vi "NIMS_NS_iir_comb.vi"(5 "Function name":string, 6 "Line number":i32, 7 "Number of outputs requested":i32, 8 "error in (no error)":errorcluster, 11 "[A]":variant[](array[variant])) -> (0 "error out":errorcluster, 3 "[funct(A)]":variant[](array[variant]))   [LabVIEW 2017]
uses:
  <vilib>/imath/engines/lvmath/Functions/Error Handling/error.ctl
  <instcachedir>/0/NIMS_RunTimeType_From StrictType (excl LVString)_1019F277F0A747EDBCA0F6C52CA54500.lvgen/NIMS_RunTimeType_From StrictType (excl LVString)_1019F277F0A747EDBCA0F6C52CA54500_000.vi
  <instcachedir>/0/NIMS_Get Scalar_w Error_1987D997E87247DDAC16EA23A5E9E4FC.lvgen/NIMS_Get Scalar_w Error_1987D997E87247DDAC16EA23A5E9E4FC_000.vi
  <instcachedir>/0/NIMS_Get Scalar_w Error_1987D997E87247DDAC16EA23A5E9E4FC.lvgen/NIMS_Get Scalar_w Error_1987D997E87247DDAC16EA23A5E9E4FC_003.vi
  <instcachedir>/0/NIMS_Get Row Vector_w Error - Matrix_7ECCFA0649AF47C08F6F0C496599EB01.lvgen/NIMS_Get Row Vector_w Error - Matrix_7ECCFA0649AF47C08F6F0C496599EB01_000.vi
  <instcachedir>/0/NIMS_Complex To Real_BE01396FDE034E8E94CEBBA1E368668D.lvgen/NIMS_Complex To Real_BE01396FDE034E8E94CEBBA1E368668D_000.vi
  <instcachedir>/0/NIMS_RunTimeType_To Numeric_1CBDAFC4EFAD4045A1DE52278D16738D.lvgen/NIMS_RunTimeType_To Numeric_1CBDAFC4EFAD4045A1DE52278D16738D_000.vi
  <vilib>/addons/Digital Filter Design/NI_DigFilter_MathScript.lvlib
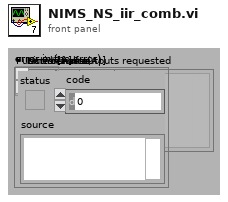
[diagram p1: front panel]
types:
  T1 = typedef "error.ctl" = enum16{"No Error", "Problem", "Input type must not be void", "Incorrect number of parameters", "Function not defined for non-numeric types", "An output variable of the user-defined function is undefined", "Function only defined for character arrays", "Function not defined for boolean, character, or single precision", "Function not defined for complex types", "Not a valid operation", "Inputs must be scalar", "Input matrices are not the same size", "Function only available on RT", "Input matrices must be nonnegative integers of the same type", "Arguments must be non-negative integers less than bitmax", "Number to complement must be less than 2^N", "Bit to get is outside range", "Bit to set is outside range", "Input must be real type ", "At least one parameter must be scalar", "Unable to display plug-in data on RT", "Function not defined for higher dimensional matrices", "Invalid attributes", "Wrong Type of Input Arguments", "Wrong Argument Option", "Invalid file identifier", "Indices must be real positive integers", "The variable is not a matrix data type.", "Number of elements must be the same for indices and values", "You cannot replace elements of a matrix with non-matrix data types.", "Cannot resize a 2D matrix with a linear index", "Unknown variable or symbol", "Indices out of range", "Empty matrix deletion can not be used with two indices", "Number of rows and columns must be the same for indices and values.", "Complex cannot be converted to Boolean", "Char cannot be converted to Boolean", "int64 cannot be converted to Boolean", "uint64 cannot be converted to Boolean", "You cannot convert a Boolean to a character.", "Incompatible input size in 3D surface function", "All rows must have the same number of columns", "Incompatible types", "Invalid matrix dimensions", "Dimension must be 1 or 2", "Base must be an integer between 2 and 36", "Invalid input", "Square matrix required", "Function 'timerstart' must be called before 'timerstop'", "Arguments must be positive real", "Step must not be zero", "Wrong number of input arguments", "Wrong number of output arguments", "Too many index arguments", "Input scalar must be >= 0", "Input scalar must be positive", "Input scalar must not be 0", "Input scalar must be in range [0,1]", "Can't use conditionally defined variable that's undefined", "Input must be a vector", "RT Exec Trace Toolkit not licensed", "Empty vector error", "All elements must be in domain [-1,1]", "All real elements of input vector must be >= 0", "All elements of input vector must be positive", "Values of input vectors are not compatible", "DAQmx not installed", "Input vector must be an increasing vector", "Dereferenced field does not exist within the struct", "A vector or matrix of structures must be indexed before it can be dereferenced", "Lenths of two input vectors are not compatible", "Invalid fieldname", "Empty matrix error", "Cannot use '.' on a type other than Struct", "Unused074", "Data type of the struct's field name is invalid", "Using . to dereference data that is not a struct", "Input struct contains invalid type ", "Size of input matrix is incompatible with input size", "Invalid format specifier", "Could not find field within struct", "Bad permutation array", "Mismatched fieldnames", "ode: User Function could not be opened", "ode: User Function signature does not meet ode requirements", "Unused085", "RunTime: MathScript could not be compiled", "Unknown function", "Only scalars and strings supported", "ode: User Function signature has incorrect number of inputs", "ode:User Function signature has incorrect number of outputs", "Range is too large", "End used without variable", "Function not available (RTE)", "Custom user error", "Arguments must be integers less than bitmax", "Shared library not found", "Header file not found", "Shared library already loaded", "Shared library not loaded", "Shared library function not found", "Shared library string return problem", "Problem calling shared library function", "Problem loading shared library from OS", "Problem parsing shared library header file", "Shared library incompatible types", "Shared library unsupported return type", "Shared library function not exported", "Shared library unsupported input type", "Problem unloading shared library from OS", "Function only available from UI", "Function specified in argument is missing", "An internal error has occurred", "Invalid object", "Invalid property", "Read-only property", "A break command has occurred", "A continue command has occurred", "A return command has occurred", "ode: times parameter invalid", "Function specified in argument has incorrect signature", "Function not found in file", "Reserved keyword cannot be defined as variable", "Reserved keyword cannot be defined as a function or script", "Arguments must be string literals", "Function not supported on this platform", "All columns must have the same number of rows", "Function ignored in RTE warning", "Cannot use : as a parameter that is not a variable", "Output can't be coerced to requested type", "Function not supported on current target", "Variable dependent on an unwired function input", "Unused132", "Unused133", "Unused134", "Unused135", "Unused136", "Unused137", "Unused138", "Unused139", "Global/Persistent must only take constants as arguments.", "Varargin must be last input in the function definition.", "Varargout must be last output in the function definition.", "Invalid output type. Cannot output a cell array of any type other than string.", "Invalid output type. Type is a dynamic struct.", "Invalid output type. Type is a struct that has a field whose type is not known until run-time", "Invalid output type. Type is a struct that has a field which is a plot object.", "MathScript parser DLL missing", "MathScript requires LabVIEW Full", "MathScript license is invalid or missing", "Varargout not supported except in assignments."}
  T2 = typedef "NIMS_CH_character datatype.ctl" = cluster{"Numeric":u8}
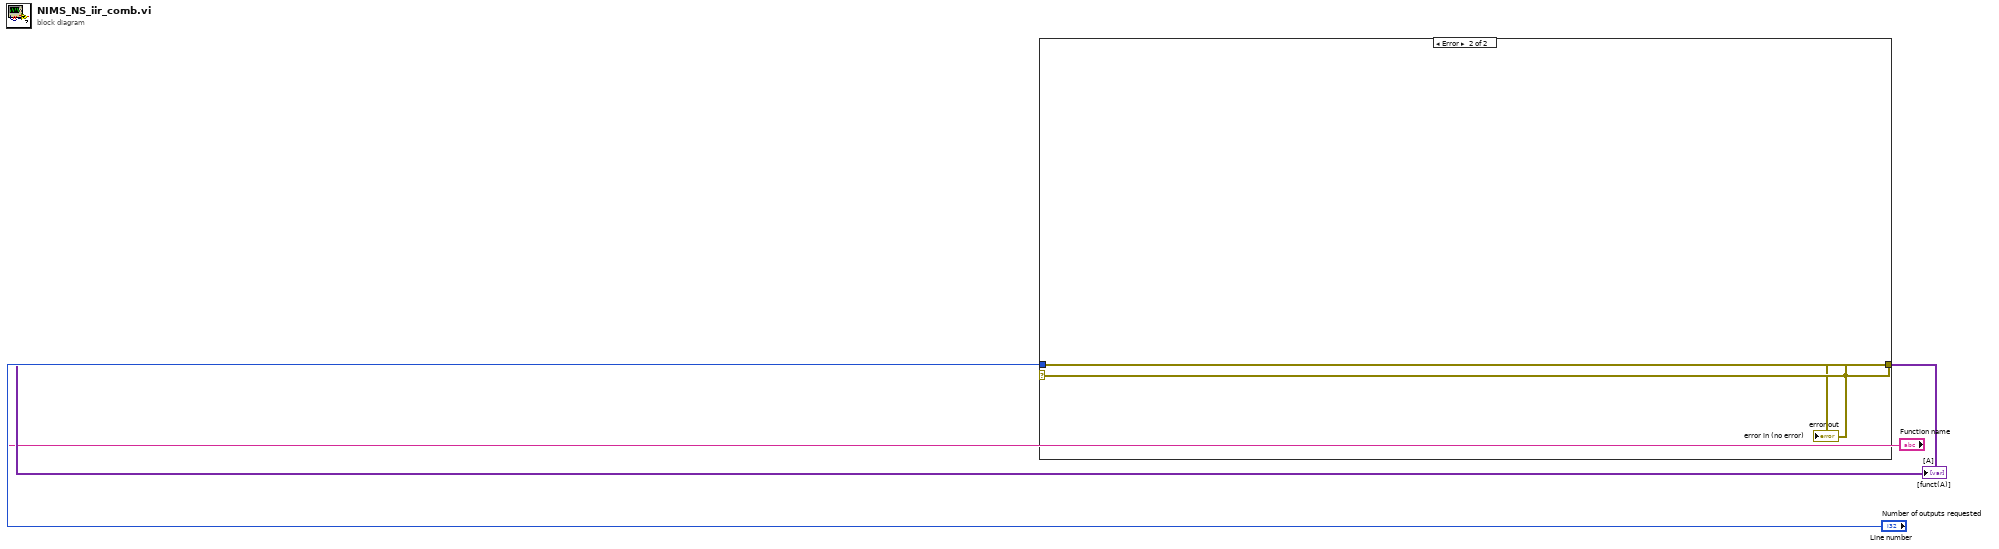
[diagram p0: block diagram]
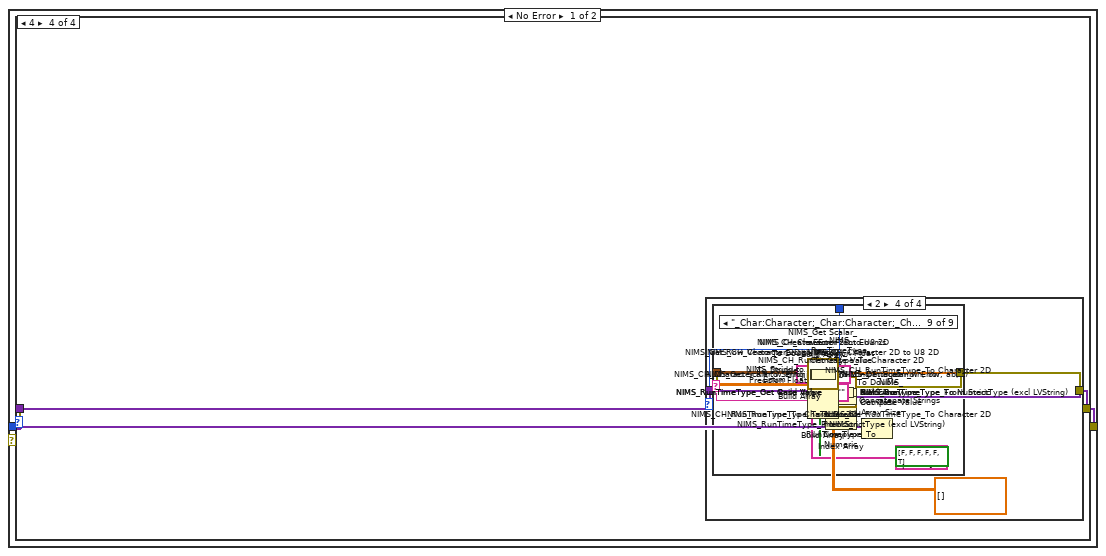
[diagram p2: hidden frame]
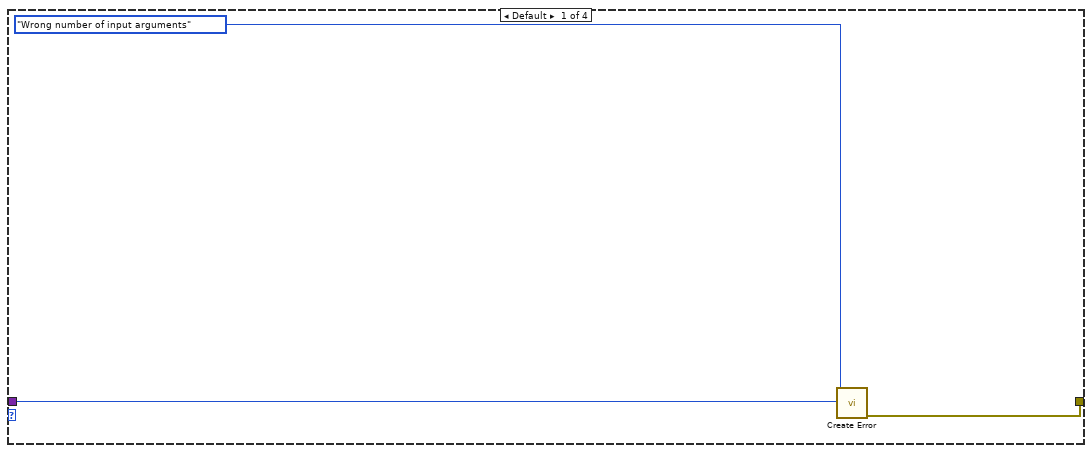
[diagram p3: hidden frame]
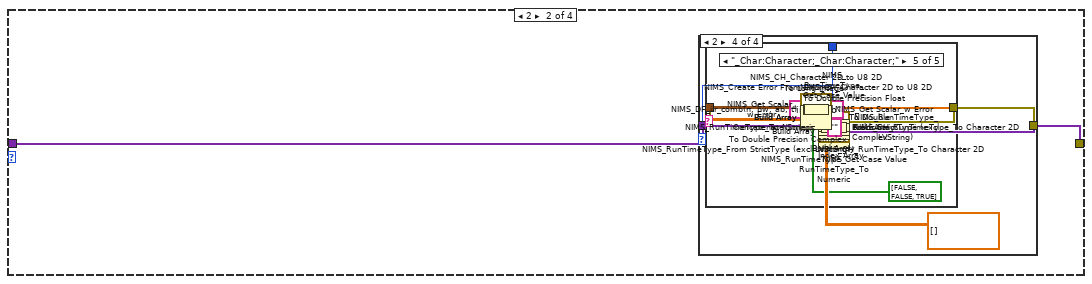
[diagram p4: hidden frame]
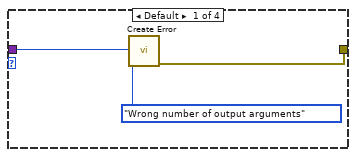
[diagram p5: hidden frame]
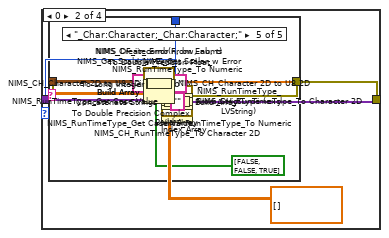
[diagram p6: hidden frame]
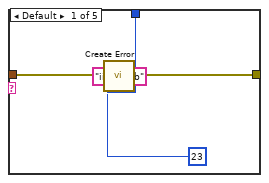
[diagram p7: hidden frame]
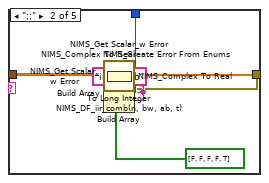
[diagram p8: hidden frame]
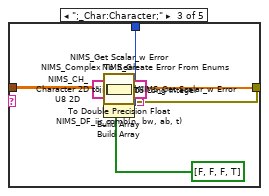
[diagram p9: hidden frame]
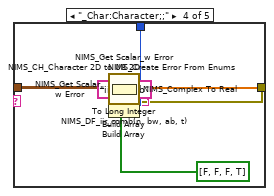
[diagram p10: hidden frame]
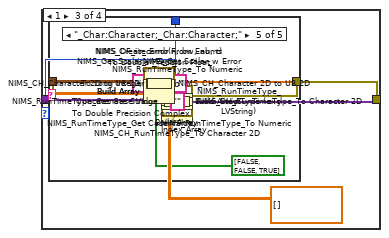
[diagram p11: hidden frame]
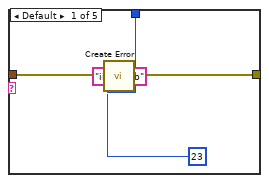
[diagram p12: hidden frame]
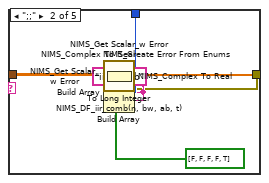
[diagram p13: hidden frame]
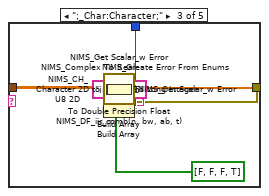
[diagram p14: hidden frame]
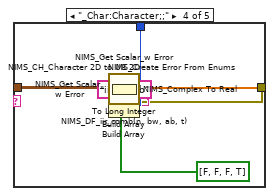
[diagram p15: hidden frame]
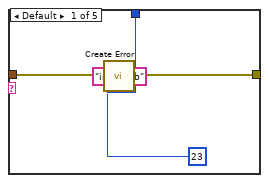
[diagram p16: hidden frame]
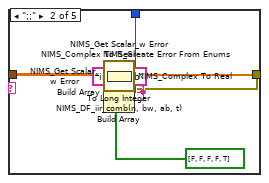
[diagram p17: hidden frame]
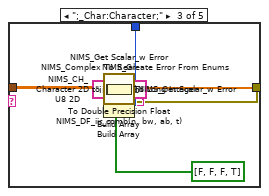
[diagram p18: hidden frame]
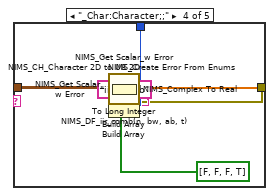
[diagram p19: hidden frame]
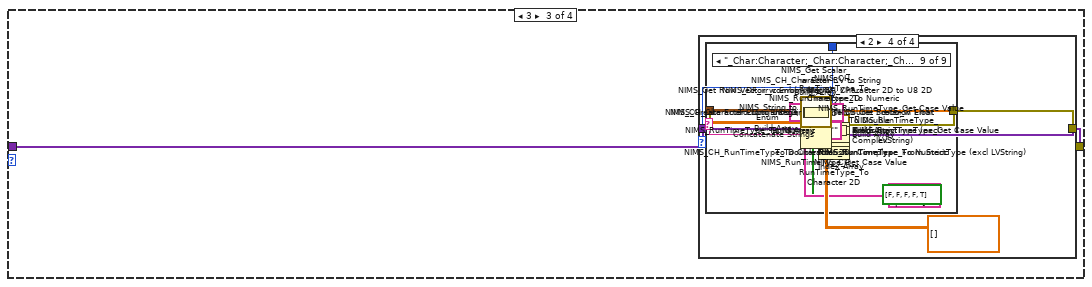
[diagram p20: hidden frame]
diagram:
  n1 = case shown="Error" "error in (no error)" {
    selector: "error in (no error)" -> [_ w2027]
    tunnel: [w15 _] -> w4
    tunnel: [w14 w2027] -> w3
    tunnel: "error in (no error)" -> [w13 _]
    tunnel: "Number of outputs requested" -> [w12 _]
    tunnel: "[A]" -> [w11 _]
    tunnel: "Function name" -> [w10 _]
    tunnel: "Line number" -> [w9 _]
    frame No Error {
      n2 = Array Size(array=w11) -> (size(s)=w8:i32)
      n3 = case shown="4" w8 {
        tunnel: [_ w27 w372 w1126] -> w15
        tunnel: w10 -> [w19 w24 w369 w1123]
        tunnel: w9 -> [w20 w25 w370 w1124]
        tunnel: w13 -> [w17 w23 w368 w1122]
        tunnel: [w16 w22 w367 w1121] -> w14
        tunnel: w12 -> [_ w21 w366 w1120]
        tunnel: w11 -> [_ w26 w371 w1125]
        frame Default {
          n4 = call <vilib>:"Create Error.vi"("Function name"=w19, "error in (no error)"=w17, "Error Enum"=error."Wrong number of input arguments", "Line number"=w20) -> ("error out"=w16:errorcluster)  [unwired: 6 in, 1 out]
        }
        frame 2 {
          n5 = case shown="2" w21 {
            tunnel: [_ w33 w141 w249] -> w27
            tunnel: w24 -> [w31 _ _ _]
            tunnel: w25 -> [w32 w52 w160 w273]
            tunnel: w23 -> [w29 w50 w158 w271]
            tunnel: [w28 w39 w147 w260] -> w22
            tunnel: w26 -> [_ w53 w161 w274]
            frame Default {
              n6 = call <vilib>:"Create Error.vi"("Function name"=w31, "error in (no error)"=w29, "Error Enum"=error."Wrong number of output arguments", "Line number"=w32) -> ("error out"=w28:errorcluster)  [unwired: 6 in, 1 out]
            }
            frame 0 {
              n7 = Index Array(array=w53) -> (element #1=w49:variant, element #2=w44:variant)  [unwired: 2 in]
              n8 = call <vilib>:"NIMS_RunTimeType_Get Case Value.vi"("Data In"=w44) -> ("Case Value"=w40:string)  [unwired: 9 in, 1 out]
              n9 = call <vilib>:"NIMS_CH_RunTimeType_To Character 2D.vi"("Variant"=w44) -> ("data"=w41:T2[][])  [unwired: 1 in]
              n10 = call-generic <vilib>:"NIMS_RunTimeType_To Numeric.vi"("DataType"=cdb[][] [], "Variant"=w44) -> ("data"=w42:cdb[][])  [unwired: 1 in]
              n11 = call <vilib>:"NIMS_RunTimeType_Get Case Value.vi"("Data In"=w49) -> ("Case Value"=w45:string)  [unwired: 9 in, 1 out]
              n12 = call <vilib>:"NIMS_CH_RunTimeType_To Character 2D.vi"("Variant"=w49) -> ("data"=w46:T2[][])  [unwired: 1 in]
              n13 = call-generic <vilib>:"NIMS_RunTimeType_To Numeric.vi"("DataType"=cdb[][] [], "Variant"=w49) -> ("data"=w47:cdb[][])  [unwired: 1 in]
              n14 = Concatenate Strings(w45, w40) -> (w51:string)
              n15 = case shown="\"_Char:Character;_Char:Character;\"" w51 {
                tunnel: w50 -> [w55 w64 w85 w106 w126]
                tunnel: [_ w59 w80 w101 w121] -> w38
                tunnel: [w54 w60 w81 w102 w122] -> w39
                tunnel: w47 -> [_ w78 w99 _ _]
                tunnel: w46 -> [_ _ _ w119 w139]
                tunnel: w42 -> [_ w74 _ w115 _]
                tunnel: w41 -> [_ _ w95 _ w135]
                tunnel: w52 -> [w58 w67 w88 w109 w129]
                frame Default {
                  n16 = call <vilib>:"Create Error.vi"("Function name"="iir_comb", "error in (no error)"=w55, "Error Enum"=23, "Line number"=w58) -> ("error out"=w54:errorcluster)  [unwired: 6 in, 1 out]
                }
                frame ";;" {
                  w62 = "iir_comb"
                  n17 = call-generic <vilib>:"NIMS_Complex To Real.vi"("A"=w74) -> ("Error Enum"=w70:T1, "Real(A)"=w73:dbl[][])  [unwired: 8 in, 1 out]
                  n18 = call-generic <vilib>:"NIMS_Get Scalar_w Error.vi"("A"=w73) -> ("Error Enum"=w69:T1, "Scalar"=w75:dbl)  [unwired: 8 in, 1 out]
                  n19 = call-generic <vilib>:"NIMS_Complex To Real.vi"("A"=w78) -> ("Error Enum"=w72:T1, "Real(A)"=w77:dbl[][])  [unwired: 8 in, 1 out]
                  n20 = To Long Integer(number=w77) -> (32bit integer=w76:i32[][])
                  n21 = call-generic <vilib>:"NIMS_Get Scalar_w Error.vi"("A"=w76) -> ("Error Enum"=w71:T1, "Scalar"=w79:i32)  [unwired: 8 in, 1 out]
                  n22 = call <vilib>:"NIMS_DF_iir_comb(n, bw, ab, t).vi"("bw"=w75, "n"=w79) -> ("error"=w68:i32, "b"=w59:dbl[])  [unwired: 7 in, 1 out]
                  n23 = Build Array(w62, w62, w62, w62, "iir_comb") -> (w65:string[])
                  n24 = Build Array(w72, w71, w70, w69, w68) -> (w66:i32[])
                  n25 = call <vilib>:"NIMS_Create Error From Enums.vi"("Error Code"=bool[] [FALSE, FALSE, FALSE, FALSE, TRUE], "error in (no error)"=w64, "Line no"=w67, "Error Enums"=w66, "Function names"=w65) -> ("error out"=w60:errorcluster)  [unwired: 6 in]
                }
                frame ";_Char:Character;" {
                  w83 = "iir_comb"
                  n26 = call <vilib>:"NIMS_CH_Character 2D to U8 2D.vi"("Character 2D array"=w95) -> ("U8 2D array"=w94:u8[][])  [unwired: 10 in]
                  n27 = To Double Precision Float(number=w94) -> (double precision float=w93:dbl[][])
                  n28 = call-generic <vilib>:"NIMS_Get Scalar_w Error.vi"("A"=w93) -> ("Error Enum"=w90:T1, "Scalar"=w96:dbl)  [unwired: 8 in, 1 out]
                  n29 = call-generic <vilib>:"NIMS_Complex To Real.vi"("A"=w99) -> ("Error Enum"=w92:T1, "Real(A)"=w98:dbl[][])  [unwired: 8 in, 1 out]
                  n30 = To Long Integer(number=w98) -> (32bit integer=w97:i32[][])
                  n31 = call-generic <vilib>:"NIMS_Get Scalar_w Error.vi"("A"=w97) -> ("Error Enum"=w91:T1, "Scalar"=w100:i32)  [unwired: 8 in, 1 out]
                  n32 = call <vilib>:"NIMS_DF_iir_comb(n, bw, ab, t).vi"("bw"=w96, "n"=w100) -> ("error"=w89:i32, "b"=w80:dbl[])  [unwired: 7 in, 1 out]
                  n33 = Build Array(w83, w83, w83, "iir_comb") -> (w86:string[])
                  n34 = Build Array(w92, w91, w90, w89) -> (w87:i32[])
                  n35 = call <vilib>:"NIMS_Create Error From Enums.vi"("Error Code"=bool[] [FALSE, FALSE, FALSE, TRUE], "error in (no error)"=w85, "Line no"=w88, "Error Enums"=w87, "Function names"=w86) -> ("error out"=w81:errorcluster)  [unwired: 6 in]
                }
                frame "_Char:Character;;" {
                  w104 = "iir_comb"
                  n36 = call-generic <vilib>:"NIMS_Complex To Real.vi"("A"=w115) -> ("Error Enum"=w112:T1, "Real(A)"=w114:dbl[][])  [unwired: 8 in, 1 out]
                  n37 = call-generic <vilib>:"NIMS_Get Scalar_w Error.vi"("A"=w114) -> ("Error Enum"=w111:T1, "Scalar"=w116:dbl)  [unwired: 8 in, 1 out]
                  n38 = call <vilib>:"NIMS_CH_Character 2D to U8 2D.vi"("Character 2D array"=w119) -> ("U8 2D array"=w118:u8[][])  [unwired: 10 in]
                  n39 = To Long Integer(number=w118) -> (32bit integer=w117:i32[][])
                  n40 = call-generic <vilib>:"NIMS_Get Scalar_w Error.vi"("A"=w117) -> ("Error Enum"=w113:T1, "Scalar"=w120:i32)  [unwired: 8 in, 1 out]
                  n41 = call <vilib>:"NIMS_DF_iir_comb(n, bw, ab, t).vi"("bw"=w116, "n"=w120) -> ("error"=w110:i32, "b"=w101:dbl[])  [unwired: 7 in, 1 out]
                  n42 = Build Array(w104, w104, w104, "iir_comb") -> (w107:string[])
                  n43 = Build Array(w113, w112, w111, w110) -> (w108:i32[])
                  n44 = call <vilib>:"NIMS_Create Error From Enums.vi"("Error Code"=bool[] [FALSE, FALSE, FALSE, TRUE], "error in (no error)"=w106, "Line no"=w109, "Error Enums"=w108, "Function names"=w107) -> ("error out"=w102:errorcluster)  [unwired: 6 in]
                }
                frame "_Char:Character;_Char:Character;" {
                  w124 = "iir_comb"
                  n45 = call <vilib>:"NIMS_CH_Character 2D to U8 2D.vi"("Character 2D array"=w135) -> ("U8 2D array"=w134:u8[][])  [unwired: 10 in]
                  n46 = To Double Precision Float(number=w134) -> (double precision float=w133:dbl[][])
                  n47 = call-generic <vilib>:"NIMS_Get Scalar_w Error.vi"("A"=w133) -> ("Error Enum"=w131:T1, "Scalar"=w136:dbl)  [unwired: 8 in, 1 out]
                  n48 = call <vilib>:"NIMS_CH_Character 2D to U8 2D.vi"("Character 2D array"=w139) -> ("U8 2D array"=w138:u8[][])  [unwired: 10 in]
                  n49 = To Long Integer(number=w138) -> (32bit integer=w137:i32[][])
                  n50 = call-generic <vilib>:"NIMS_Get Scalar_w Error.vi"("A"=w137) -> ("Error Enum"=w132:T1, "Scalar"=w140:i32)  [unwired: 8 in, 1 out]
                  n51 = call <vilib>:"NIMS_DF_iir_comb(n, bw, ab, t).vi"("bw"=w136, "n"=w140) -> ("error"=w130:i32, "b"=w121:dbl[])  [unwired: 7 in, 1 out]
                  n52 = Build Array(w124, w124, "iir_comb") -> (w127:string[])
                  n53 = Build Array(w132, w131, w130) -> (w128:i32[])
                  n54 = call <vilib>:"NIMS_Create Error From Enums.vi"("Error Code"=bool[] [FALSE, FALSE, TRUE], "error in (no error)"=w126, "Line no"=w129, "Error Enums"=w128, "Function names"=w127) -> ("error out"=w122:errorcluster)  [unwired: 6 in]
                }
              }
              n55 = Build Array(w38) -> (w37:dbl[][])
              n56 = To Double Precision Complex(1:w37) -> (0:w36:cdb[][])
              n57 = call-generic <vilib>:"NIMS_RunTimeType_From StrictType (excl LVString).vi"("Plug-In Name"="", "Data In"=w36) -> ("Data Out"=w34:variant)  [unwired: 2 in]
              n58 = Build Array(w34) -> (w33:variant[])
            }
            frame 1 {
              n59 = Index Array(array=w161) -> (element #1=w157:variant, element #2=w152:variant)  [unwired: 2 in]
              n60 = call <vilib>:"NIMS_RunTimeType_Get Case Value.vi"("Data In"=w152) -> ("Case Value"=w148:string)  [unwired: 9 in, 1 out]
              n61 = call <vilib>:"NIMS_CH_RunTimeType_To Character 2D.vi"("Variant"=w152) -> ("data"=w149:T2[][])  [unwired: 1 in]
              n62 = call-generic <vilib>:"NIMS_RunTimeType_To Numeric.vi"("DataType"=cdb[][] [], "Variant"=w152) -> ("data"=w150:cdb[][])  [unwired: 1 in]
              n63 = call <vilib>:"NIMS_RunTimeType_Get Case Value.vi"("Data In"=w157) -> ("Case Value"=w153:string)  [unwired: 9 in, 1 out]
              n64 = call <vilib>:"NIMS_CH_RunTimeType_To Character 2D.vi"("Variant"=w157) -> ("data"=w154:T2[][])  [unwired: 1 in]
              n65 = call-generic <vilib>:"NIMS_RunTimeType_To Numeric.vi"("DataType"=cdb[][] [], "Variant"=w157) -> ("data"=w155:cdb[][])  [unwired: 1 in]
              n66 = Concatenate Strings(w153, w148) -> (w159:string)
              n67 = case shown="\"_Char:Character;_Char:Character;\"" w159 {
                tunnel: w158 -> [w163 w172 w193 w214 w234]
                tunnel: [_ w167 w188 w209 w229] -> w146
                tunnel: [w162 w168 w189 w210 w230] -> w147
                tunnel: w155 -> [_ w186 w207 _ _]
                tunnel: w154 -> [_ _ _ w227 w247]
                tunnel: w150 -> [_ w182 _ w223 _]
                tunnel: w149 -> [_ _ w203 _ w243]
                tunnel: w160 -> [w166 w175 w196 w217 w237]
                frame Default {
                  n68 = call <vilib>:"Create Error.vi"("Function name"="iir_comb", "error in (no error)"=w163, "Error Enum"=23, "Line number"=w166) -> ("error out"=w162:errorcluster)  [unwired: 6 in, 1 out]
                }
                frame ";;" {
                  w170 = "iir_comb"
                  n69 = call-generic <vilib>:"NIMS_Complex To Real.vi"("A"=w182) -> ("Error Enum"=w178:T1, "Real(A)"=w181:dbl[][])  [unwired: 8 in, 1 out]
                  n70 = call-generic <vilib>:"NIMS_Get Scalar_w Error.vi"("A"=w181) -> ("Error Enum"=w177:T1, "Scalar"=w183:dbl)  [unwired: 8 in, 1 out]
                  n71 = call-generic <vilib>:"NIMS_Complex To Real.vi"("A"=w186) -> ("Error Enum"=w180:T1, "Real(A)"=w185:dbl[][])  [unwired: 8 in, 1 out]
                  n72 = To Long Integer(number=w185) -> (32bit integer=w184:i32[][])
                  n73 = call-generic <vilib>:"NIMS_Get Scalar_w Error.vi"("A"=w184) -> ("Error Enum"=w179:T1, "Scalar"=w187:i32)  [unwired: 8 in, 1 out]
                  n74 = call <vilib>:"NIMS_DF_iir_comb(n, bw, ab, t).vi"("bw"=w183, "n"=w187) -> ("error"=w176:i32, "b"=w167:dbl[])  [unwired: 7 in, 1 out]
                  n75 = Build Array(w170, w170, w170, w170, "iir_comb") -> (w173:string[])
                  n76 = Build Array(w180, w179, w178, w177, w176) -> (w174:i32[])
                  n77 = call <vilib>:"NIMS_Create Error From Enums.vi"("Error Code"=bool[] [FALSE, FALSE, FALSE, FALSE, TRUE], "error in (no error)"=w172, "Line no"=w175, "Error Enums"=w174, "Function names"=w173) -> ("error out"=w168:errorcluster)  [unwired: 6 in]
                }
                frame ";_Char:Character;" {
                  w191 = "iir_comb"
                  n78 = call <vilib>:"NIMS_CH_Character 2D to U8 2D.vi"("Character 2D array"=w203) -> ("U8 2D array"=w202:u8[][])  [unwired: 10 in]
                  n79 = To Double Precision Float(number=w202) -> (double precision float=w201:dbl[][])
                  n80 = call-generic <vilib>:"NIMS_Get Scalar_w Error.vi"("A"=w201) -> ("Error Enum"=w198:T1, "Scalar"=w204:dbl)  [unwired: 8 in, 1 out]
                  n81 = call-generic <vilib>:"NIMS_Complex To Real.vi"("A"=w207) -> ("Error Enum"=w200:T1, "Real(A)"=w206:dbl[][])  [unwired: 8 in, 1 out]
                  n82 = To Long Integer(number=w206) -> (32bit integer=w205:i32[][])
                  n83 = call-generic <vilib>:"NIMS_Get Scalar_w Error.vi"("A"=w205) -> ("Error Enum"=w199:T1, "Scalar"=w208:i32)  [unwired: 8 in, 1 out]
                  n84 = call <vilib>:"NIMS_DF_iir_comb(n, bw, ab, t).vi"("bw"=w204, "n"=w208) -> ("error"=w197:i32, "b"=w188:dbl[])  [unwired: 7 in, 1 out]
                  n85 = Build Array(w191, w191, w191, "iir_comb") -> (w194:string[])
                  n86 = Build Array(w200, w199, w198, w197) -> (w195:i32[])
                  n87 = call <vilib>:"NIMS_Create Error From Enums.vi"("Error Code"=bool[] [FALSE, FALSE, FALSE, TRUE], "error in (no error)"=w193, "Line no"=w196, "Error Enums"=w195, "Function names"=w194) -> ("error out"=w189:errorcluster)  [unwired: 6 in]
                }
                frame "_Char:Character;;" {
                  w212 = "iir_comb"
                  n88 = call-generic <vilib>:"NIMS_Complex To Real.vi"("A"=w223) -> ("Error Enum"=w220:T1, "Real(A)"=w222:dbl[][])  [unwired: 8 in, 1 out]
                  n89 = call-generic <vilib>:"NIMS_Get Scalar_w Error.vi"("A"=w222) -> ("Error Enum"=w219:T1, "Scalar"=w224:dbl)  [unwired: 8 in, 1 out]
                  n90 = call <vilib>:"NIMS_CH_Character 2D to U8 2D.vi"("Character 2D array"=w227) -> ("U8 2D array"=w226:u8[][])  [unwired: 10 in]
                  n91 = To Long Integer(number=w226) -> (32bit integer=w225:i32[][])
                  n92 = call-generic <vilib>:"NIMS_Get Scalar_w Error.vi"("A"=w225) -> ("Error Enum"=w221:T1, "Scalar"=w228:i32)  [unwired: 8 in, 1 out]
                  n93 = call <vilib>:"NIMS_DF_iir_comb(n, bw, ab, t).vi"("bw"=w224, "n"=w228) -> ("error"=w218:i32, "b"=w209:dbl[])  [unwired: 7 in, 1 out]
                  n94 = Build Array(w212, w212, w212, "iir_comb") -> (w215:string[])
                  n95 = Build Array(w221, w220, w219, w218) -> (w216:i32[])
                  n96 = call <vilib>:"NIMS_Create Error From Enums.vi"("Error Code"=bool[] [FALSE, FALSE, FALSE, TRUE], "error in (no error)"=w214, "Line no"=w217, "Error Enums"=w216, "Function names"=w215) -> ("error out"=w210:errorcluster)  [unwired: 6 in]
                }
                frame "_Char:Character;_Char:Character;" {
                  w232 = "iir_comb"
                  n97 = call <vilib>:"NIMS_CH_Character 2D to U8 2D.vi"("Character 2D array"=w243) -> ("U8 2D array"=w242:u8[][])  [unwired: 10 in]
                  n98 = To Double Precision Float(number=w242) -> (double precision float=w241:dbl[][])
                  n99 = call-generic <vilib>:"NIMS_Get Scalar_w Error.vi"("A"=w241) -> ("Error Enum"=w239:T1, "Scalar"=w244:dbl)  [unwired: 8 in, 1 out]
                  n100 = call <vilib>:"NIMS_CH_Character 2D to U8 2D.vi"("Character 2D array"=w247) -> ("U8 2D array"=w246:u8[][])  [unwired: 10 in]
                  n101 = To Long Integer(number=w246) -> (32bit integer=w245:i32[][])
                  n102 = call-generic <vilib>:"NIMS_Get Scalar_w Error.vi"("A"=w245) -> ("Error Enum"=w240:T1, "Scalar"=w248:i32)  [unwired: 8 in, 1 out]
                  n103 = call <vilib>:"NIMS_DF_iir_comb(n, bw, ab, t).vi"("bw"=w244, "n"=w248) -> ("error"=w238:i32, "b"=w229:dbl[])  [unwired: 7 in, 1 out]
                  n104 = Build Array(w232, w232, "iir_comb") -> (w235:string[])
                  n105 = Build Array(w240, w239, w238) -> (w236:i32[])
                  n106 = call <vilib>:"NIMS_Create Error From Enums.vi"("Error Code"=bool[] [FALSE, FALSE, TRUE], "error in (no error)"=w234, "Line no"=w237, "Error Enums"=w236, "Function names"=w235) -> ("error out"=w230:errorcluster)  [unwired: 6 in]
                }
              }
              n107 = Build Array(w146) -> (w145:dbl[][])
              n108 = To Double Precision Complex(1:w145) -> (0:w144:cdb[][])
              n109 = call-generic <vilib>:"NIMS_RunTimeType_From StrictType (excl LVString).vi"("Plug-In Name"="", "Data In"=w144) -> ("Data Out"=w142:variant)  [unwired: 2 in]
              n110 = Build Array(w142) -> (w141:variant[])
            }
            frame 2 {
              n111 = Index Array(array=w274) -> (element #1=w270:variant, element #2=w265:variant)  [unwired: 2 in]
              n112 = call <vilib>:"NIMS_RunTimeType_Get Case Value.vi"("Data In"=w265) -> ("Case Value"=w261:string)  [unwired: 9 in, 1 out]
              n113 = call <vilib>:"NIMS_CH_RunTimeType_To Character 2D.vi"("Variant"=w265) -> ("data"=w262:T2[][])  [unwired: 1 in]
              n114 = call-generic <vilib>:"NIMS_RunTimeType_To Numeric.vi"("DataType"=cdb[][] [], "Variant"=w265) -> ("data"=w263:cdb[][])  [unwired: 1 in]
              n115 = call <vilib>:"NIMS_RunTimeType_Get Case Value.vi"("Data In"=w270) -> ("Case Value"=w266:string)  [unwired: 9 in, 1 out]
              n116 = call <vilib>:"NIMS_CH_RunTimeType_To Character 2D.vi"("Variant"=w270) -> ("data"=w267:T2[][])  [unwired: 1 in]
              n117 = call-generic <vilib>:"NIMS_RunTimeType_To Numeric.vi"("DataType"=cdb[][] [], "Variant"=w270) -> ("data"=w268:cdb[][])  [unwired: 1 in]
              n118 = Concatenate Strings(w266, w261) -> (w272:string)
              n119 = case shown="\"_Char:Character;_Char:Character;\"" w272 {
                tunnel: w271 -> [w276 w286 w308 w330 w351]
                tunnel: [_ w281 w303 w325 w346] -> w259
                tunnel: [_ w280 w302 w324 w345] -> w255
                tunnel: [w275 w282 w304 w326 w347] -> w260
                tunnel: w268 -> [_ w300 w322 _ _]
                tunnel: w267 -> [_ _ _ w343 w364]
                tunnel: w263 -> [_ w296 _ w339 _]
                tunnel: w262 -> [_ _ w318 _ w360]
                tunnel: w273 -> [w279 w289 w311 w333 w354]
                frame Default {
                  n120 = call <vilib>:"Create Error.vi"("Function name"="iir_comb", "error in (no error)"=w276, "Error Enum"=23, "Line number"=w279) -> ("error out"=w275:errorcluster)  [unwired: 6 in, 1 out]
                }
                frame ";;" {
                  w284 = "iir_comb"
                  n121 = call-generic <vilib>:"NIMS_Complex To Real.vi"("A"=w296) -> ("Error Enum"=w292:T1, "Real(A)"=w295:dbl[][])  [unwired: 8 in, 1 out]
                  n122 = call-generic <vilib>:"NIMS_Get Scalar_w Error.vi"("A"=w295) -> ("Error Enum"=w291:T1, "Scalar"=w297:dbl)  [unwired: 8 in, 1 out]
                  n123 = call-generic <vilib>:"NIMS_Complex To Real.vi"("A"=w300) -> ("Error Enum"=w294:T1, "Real(A)"=w299:dbl[][])  [unwired: 8 in, 1 out]
                  n124 = To Long Integer(number=w299) -> (32bit integer=w298:i32[][])
                  n125 = call-generic <vilib>:"NIMS_Get Scalar_w Error.vi"("A"=w298) -> ("Error Enum"=w293:T1, "Scalar"=w301:i32)  [unwired: 8 in, 1 out]
                  n126 = call <vilib>:"NIMS_DF_iir_comb(n, bw, ab, t).vi"("bw"=w297, "n"=w301) -> ("error"=w290:i32, "a"=w280:dbl[], "b"=w281:dbl[])  [unwired: 7 in]
                  n127 = Build Array(w284, w284, w284, w284, "iir_comb") -> (w287:string[])
                  n128 = Build Array(w294, w293, w292, w291, w290) -> (w288:i32[])
                  n129 = call <vilib>:"NIMS_Create Error From Enums.vi"("Error Code"=bool[] [FALSE, FALSE, FALSE, FALSE, TRUE], "error in (no error)"=w286, "Line no"=w289, "Error Enums"=w288, "Function names"=w287) -> ("error out"=w282:errorcluster)  [unwired: 6 in]
                }
                frame ";_Char:Character;" {
                  w306 = "iir_comb"
                  n130 = call <vilib>:"NIMS_CH_Character 2D to U8 2D.vi"("Character 2D array"=w318) -> ("U8 2D array"=w317:u8[][])  [unwired: 10 in]
                  n131 = To Double Precision Float(number=w317) -> (double precision float=w316:dbl[][])
                  n132 = call-generic <vilib>:"NIMS_Get Scalar_w Error.vi"("A"=w316) -> ("Error Enum"=w313:T1, "Scalar"=w319:dbl)  [unwired: 8 in, 1 out]
                  n133 = call-generic <vilib>:"NIMS_Complex To Real.vi"("A"=w322) -> ("Error Enum"=w315:T1, "Real(A)"=w321:dbl[][])  [unwired: 8 in, 1 out]
                  n134 = To Long Integer(number=w321) -> (32bit integer=w320:i32[][])
                  n135 = call-generic <vilib>:"NIMS_Get Scalar_w Error.vi"("A"=w320) -> ("Error Enum"=w314:T1, "Scalar"=w323:i32)  [unwired: 8 in, 1 out]
                  n136 = call <vilib>:"NIMS_DF_iir_comb(n, bw, ab, t).vi"("bw"=w319, "n"=w323) -> ("error"=w312:i32, "a"=w302:dbl[], "b"=w303:dbl[])  [unwired: 7 in]
                  n137 = Build Array(w306, w306, w306, "iir_comb") -> (w309:string[])
                  n138 = Build Array(w315, w314, w313, w312) -> (w310:i32[])
                  n139 = call <vilib>:"NIMS_Create Error From Enums.vi"("Error Code"=bool[] [FALSE, FALSE, FALSE, TRUE], "error in (no error)"=w308, "Line no"=w311, "Error Enums"=w310, "Function names"=w309) -> ("error out"=w304:errorcluster)  [unwired: 6 in]
                }
                frame "_Char:Character;;" {
                  w328 = "iir_comb"
                  n140 = call-generic <vilib>:"NIMS_Complex To Real.vi"("A"=w339) -> ("Error Enum"=w336:T1, "Real(A)"=w338:dbl[][])  [unwired: 8 in, 1 out]
                  n141 = call-generic <vilib>:"NIMS_Get Scalar_w Error.vi"("A"=w338) -> ("Error Enum"=w335:T1, "Scalar"=w340:dbl)  [unwired: 8 in, 1 out]
                  n142 = call <vilib>:"NIMS_CH_Character 2D to U8 2D.vi"("Character 2D array"=w343) -> ("U8 2D array"=w342:u8[][])  [unwired: 10 in]
                  n143 = To Long Integer(number=w342) -> (32bit integer=w341:i32[][])
                  n144 = call-generic <vilib>:"NIMS_Get Scalar_w Error.vi"("A"=w341) -> ("Error Enum"=w337:T1, "Scalar"=w344:i32)  [unwired: 8 in, 1 out]
                  n145 = call <vilib>:"NIMS_DF_iir_comb(n, bw, ab, t).vi"("bw"=w340, "n"=w344) -> ("error"=w334:i32, "a"=w324:dbl[], "b"=w325:dbl[])  [unwired: 7 in]
                  n146 = Build Array(w328, w328, w328, "iir_comb") -> (w331:string[])
                  n147 = Build Array(w337, w336, w335, w334) -> (w332:i32[])
                  n148 = call <vilib>:"NIMS_Create Error From Enums.vi"("Error Code"=bool[] [FALSE, FALSE, FALSE, TRUE], "error in (no error)"=w330, "Line no"=w333, "Error Enums"=w332, "Function names"=w331) -> ("error out"=w326:errorcluster)  [unwired: 6 in]
                }
                frame "_Char:Character;_Char:Character;" {
                  w349 = "iir_comb"
                  n149 = call <vilib>:"NIMS_CH_Character 2D to U8 2D.vi"("Character 2D array"=w360) -> ("U8 2D array"=w359:u8[][])  [unwired: 10 in]
                  n150 = To Double Precision Float(number=w359) -> (double precision float=w358:dbl[][])
                  n151 = call-generic <vilib>:"NIMS_Get Scalar_w Error.vi"("A"=w358) -> ("Error Enum"=w356:T1, "Scalar"=w361:dbl)  [unwired: 8 in, 1 out]
                  n152 = call <vilib>:"NIMS_CH_Character 2D to U8 2D.vi"("Character 2D array"=w364) -> ("U8 2D array"=w363:u8[][])  [unwired: 10 in]
                  n153 = To Long Integer(number=w363) -> (32bit integer=w362:i32[][])
                  n154 = call-generic <vilib>:"NIMS_Get Scalar_w Error.vi"("A"=w362) -> ("Error Enum"=w357:T1, "Scalar"=w365:i32)  [unwired: 8 in, 1 out]
                  n155 = call <vilib>:"NIMS_DF_iir_comb(n, bw, ab, t).vi"("bw"=w361, "n"=w365) -> ("error"=w355:i32, "a"=w345:dbl[], "b"=w346:dbl[])  [unwired: 7 in]
                  n156 = Build Array(w349, w349, "iir_comb") -> (w352:string[])
                  n157 = Build Array(w357, w356, w355) -> (w353:i32[])
                  n158 = call <vilib>:"NIMS_Create Error From Enums.vi"("Error Code"=bool[] [FALSE, FALSE, TRUE], "error in (no error)"=w351, "Line no"=w354, "Error Enums"=w353, "Function names"=w352) -> ("error out"=w347:errorcluster)  [unwired: 6 in]
                }
              }
              n159 = Build Array(w255) -> (w254:dbl[][])
              n160 = To Double Precision Complex(1:w254) -> (0:w253:cdb[][])
              n161 = call-generic <vilib>:"NIMS_RunTimeType_From StrictType (excl LVString).vi"("Plug-In Name"="", "Data In"=w253) -> ("Data Out"=w250:variant)  [unwired: 2 in]
              n162 = Build Array(w259) -> (w258:dbl[][])
              n163 = To Double Precision Complex(1:w258) -> (0:w257:cdb[][])
              n164 = call-generic <vilib>:"NIMS_RunTimeType_From StrictType (excl LVString).vi"("Plug-In Name"="", "Data In"=w257) -> ("Data Out"=w251:variant)  [unwired: 2 in]
              n165 = Build Array(w251, w250) -> (w249:variant[])
            }
          }
        }
        frame 3 {
          n166 = case shown="2" w366 {
            tunnel: [_ w378 w621 w864] -> w372
            tunnel: w369 -> [w376 _ _ _]
            tunnel: w370 -> [w377 w402 w645 w893]
            tunnel: w368 -> [w374 w400 w643 w891]
            tunnel: [w373 w384 w627 w875] -> w367
            tunnel: w371 -> [_ w403 w646 w894]
            frame Default {
              n167 = call <vilib>:"Create Error.vi"("Function name"=w376, "error in (no error)"=w374, "Error Enum"=error."Wrong number of output arguments", "Line number"=w377) -> ("error out"=w373:errorcluster)  [unwired: 6 in, 1 out]
            }
            frame 0 {
              n168 = Index Array(array=w403) -> (element #1=w399:variant, element #2=w394:variant, element #3=w389:variant)  [unwired: 3 in]
              n169 = call <vilib>:"NIMS_RunTimeType_Get Case Value.vi"("Data In"=w389) -> ("Case Value"=w385:string)  [unwired: 9 in, 1 out]
              n170 = call <vilib>:"NIMS_CH_RunTimeType_To Character 2D.vi"("Variant"=w389) -> ("data"=w386:T2[][])  [unwired: 1 in]
              n171 = call-generic <vilib>:"NIMS_RunTimeType_To Numeric.vi"("DataType"=cdb[][] [], "Variant"=w389) -> ("data"=w387:cdb[][])  [unwired: 1 in]
              n172 = call <vilib>:"NIMS_RunTimeType_Get Case Value.vi"("Data In"=w394) -> ("Case Value"=w390:string)  [unwired: 9 in, 1 out]
              n173 = call <vilib>:"NIMS_CH_RunTimeType_To Character 2D.vi"("Variant"=w394) -> ("data"=w391:T2[][])  [unwired: 1 in]
              n174 = call-generic <vilib>:"NIMS_RunTimeType_To Numeric.vi"("DataType"=cdb[][] [], "Variant"=w394) -> ("data"=w392:cdb[][])  [unwired: 1 in]
              n175 = call <vilib>:"NIMS_RunTimeType_Get Case Value.vi"("Data In"=w399) -> ("Case Value"=w395:string)  [unwired: 9 in, 1 out]
              n176 = call <vilib>:"NIMS_CH_RunTimeType_To Character 2D.vi"("Variant"=w399) -> ("data"=w396:T2[][])  [unwired: 1 in]
              n177 = call-generic <vilib>:"NIMS_RunTimeType_To Numeric.vi"("DataType"=cdb[][] [], "Variant"=w399) -> ("data"=w397:cdb[][])  [unwired: 1 in]
              n178 = Concatenate Strings(w395, w390, w385) -> (w401:string)
              n179 = case shown="\"_Char:Character;_Char:Character;_Char:Character;\"" w401 {
                tunnel: w400 -> [w405 w414 w440 w468 w494 w522 w547 w574 w599]
                tunnel: [_ w409 w435 w463 w489 w517 w542 w569 w594] -> w383
                tunnel: [w404 w410 w436 w464 w490 w518 w543 w570 w595] -> w384
                tunnel: w397 -> [_ w433 w461 w487 w515 _ _ _ _]
                tunnel: w396 -> [_ _ _ _ _ w540 w567 w592 w619]
                tunnel: w392 -> [_ w429 w457 _ _ w536 w563 _ _]
                tunnel: w391 -> [_ _ _ w483 w511 _ _ w588 w615]
                tunnel: w387 -> [_ w426 _ w479 _ w533 _ w584 _]
                tunnel: w386 -> [_ _ w453 _ w506 _ w559 _ w610]
                tunnel: w402 -> [w408 w417 w443 w471 w497 w525 w550 w577 w602]
                frame Default {
                  n180 = call <vilib>:"Create Error.vi"("Function name"="iir_comb", "error in (no error)"=w405, "Error Enum"=23, "Line number"=w408) -> ("error out"=w404:errorcluster)  [unwired: 6 in, 1 out]
                }
                frame ";;;" {
                  w412 = "iir_comb"
                  n181 = call-generic <vilib>:"NIMS_Complex To Real.vi"("A"=w426) -> ("Error Enum"=w420:T1, "Real(A)"=w425:dbl[][])  [unwired: 8 in, 1 out]
                  n182 = call-generic <vilib>:"NIMS_Get Scalar_w Error.vi"("A"=w425) -> ("Error Enum"=w419:T1, "Scalar"=w427:dbl)  [unwired: 8 in, 1 out]
                  n183 = call-generic <vilib>:"NIMS_Complex To Real.vi"("A"=w429) -> ("Error Enum"=w422:T1, "Real(A)"=w428:dbl[][])  [unwired: 8 in, 1 out]
                  n184 = call-generic <vilib>:"NIMS_Get Scalar_w Error.vi"("A"=w428) -> ("Error Enum"=w421:T1, "Scalar"=w430:dbl)  [unwired: 8 in, 1 out]
                  n185 = call-generic <vilib>:"NIMS_Complex To Real.vi"("A"=w433) -> ("Error Enum"=w424:T1, "Real(A)"=w432:dbl[][])  [unwired: 8 in, 1 out]
                  n186 = To Long Integer(number=w432) -> (32bit integer=w431:i32[][])
                  n187 = call-generic <vilib>:"NIMS_Get Scalar_w Error.vi"("A"=w431) -> ("Error Enum"=w423:T1, "Scalar"=w434:i32)  [unwired: 8 in, 1 out]
                  n188 = call <vilib>:"NIMS_DF_iir_comb(n, bw, ab, t).vi"("ab"=w427, "bw"=w430, "n"=w434) -> ("error"=w418:i32, "b"=w409:dbl[])  [unwired: 6 in, 1 out]
                  n189 = Build Array(w412, w412, w412, w412, w412, w412, "iir_comb") -> (w415:string[])
                  n190 = Build Array(w424, w423, w422, w421, w420, w419, w418) -> (w416:i32[])
                  n191 = call <vilib>:"NIMS_Create Error From Enums.vi"("Error Code"=bool[] [FALSE, FALSE, FALSE, FALSE, FALSE, FALSE, TRUE], "error in (no error)"=w414, "Line no"=w417, "Error Enums"=w416, "Function names"=w415) -> ("error out"=w410:errorcluster)  [unwired: 6 in]
                }
                frame ";;_Char:Character;" {
                  w438 = "iir_comb"
                  n192 = call-generic <vilib>:"NIMS_Get Row Vector_w Error - Matrix.vi"("A"=w453) -> ("Error Enum"=w446:T1, "Row Vector"=w452:T2[])  [unwired: 8 in, 1 out]
                  n193 = call <vilib>:"NIMS_CH_Character RV to String.vi"("Character array"=w452) -> ("String"=w454:string)  [unwired: 10 in]
                  n194 = call <vilib>:"NIMS_String to Enum.vi"("Input String"=w454, "Enum choices"=string[] ["notch", "peak"] ("Enum Options")) -> ("Error Enum"=w445:T1, "Enum Index"=w455:i32)  [unwired: 8 in]
                  n195 = call-generic <vilib>:"NIMS_Complex To Real.vi"("A"=w457) -> ("Error Enum"=w448:T1, "Real(A)"=w456:dbl[][])  [unwired: 8 in, 1 out]
                  n196 = call-generic <vilib>:"NIMS_Get Scalar_w Error.vi"("A"=w456) -> ("Error Enum"=w447:T1, "Scalar"=w458:dbl)  [unwired: 8 in, 1 out]
                  n197 = call-generic <vilib>:"NIMS_Complex To Real.vi"("A"=w461) -> ("Error Enum"=w450:T1, "Real(A)"=w460:dbl[][])  [unwired: 8 in, 1 out]
                  n198 = To Long Integer(number=w460) -> (32bit integer=w459:i32[][])
                  n199 = call-generic <vilib>:"NIMS_Get Scalar_w Error.vi"("A"=w459) -> ("Error Enum"=w449:T1, "Scalar"=w462:i32)  [unwired: 8 in, 1 out]
                  n200 = call <vilib>:"NIMS_DF_iir_comb(n, bw, t).vi"("type"=w455, "bw"=w458, "n"=w462) -> ("error"=w444:i32, "b"=w435:dbl[])  [unwired: 6 in, 1 out]
                  n201 = Build Array(w438, w438, w438, w438, w438, w438, "iir_comb") -> (w441:string[])
                  n202 = Build Array(w450, w449, w448, w447, w446, w445, w444) -> (w442:i32[])
                  n203 = call <vilib>:"NIMS_Create Error From Enums.vi"("Error Code"=bool[] [FALSE, FALSE, FALSE, FALSE, FALSE, FALSE, TRUE], "error in (no error)"=w440, "Line no"=w443, "Error Enums"=w442, "Function names"=w441) -> ("error out"=w436:errorcluster)  [unwired: 6 in]
                }
                frame ";_Char:Character;;" {
                  w466 = "iir_comb"
                  n204 = call-generic <vilib>:"NIMS_Complex To Real.vi"("A"=w479) -> ("Error Enum"=w474:T1, "Real(A)"=w478:dbl[][])  [unwired: 8 in, 1 out]
                  n205 = call-generic <vilib>:"NIMS_Get Scalar_w Error.vi"("A"=w478) -> ("Error Enum"=w473:T1, "Scalar"=w480:dbl)  [unwired: 8 in, 1 out]
                  n206 = call <vilib>:"NIMS_CH_Character 2D to U8 2D.vi"("Character 2D array"=w483) -> ("U8 2D array"=w482:u8[][])  [unwired: 10 in]
                  n207 = To Double Precision Float(number=w482) -> (double precision float=w481:dbl[][])
                  n208 = call-generic <vilib>:"NIMS_Get Scalar_w Error.vi"("A"=w481) -> ("Error Enum"=w475:T1, "Scalar"=w484:dbl)  [unwired: 8 in, 1 out]
                  n209 = call-generic <vilib>:"NIMS_Complex To Real.vi"("A"=w487) -> ("Error Enum"=w477:T1, "Real(A)"=w486:dbl[][])  [unwired: 8 in, 1 out]
                  n210 = To Long Integer(number=w486) -> (32bit integer=w485:i32[][])
                  n211 = call-generic <vilib>:"NIMS_Get Scalar_w Error.vi"("A"=w485) -> ("Error Enum"=w476:T1, "Scalar"=w488:i32)  [unwired: 8 in, 1 out]
                  n212 = call <vilib>:"NIMS_DF_iir_comb(n, bw, ab, t).vi"("ab"=w480, "bw"=w484, "n"=w488) -> ("error"=w472:i32, "b"=w463:dbl[])  [unwired: 6 in, 1 out]
                  n213 = Build Array(w466, w466, w466, w466, w466, "iir_comb") -> (w469:string[])
                  n214 = Build Array(w477, w476, w475, w474, w473, w472) -> (w470:i32[])
                  n215 = call <vilib>:"NIMS_Create Error From Enums.vi"("Error Code"=bool[] [FALSE, FALSE, FALSE, FALSE, FALSE, TRUE], "error in (no error)"=w468, "Line no"=w471, "Error Enums"=w470, "Function names"=w469) -> ("error out"=w464:errorcluster)  [unwired: 6 in]
                }
                frame ";_Char:Character;_Char:Character;" {
                  w492 = "iir_comb"
                  n216 = call-generic <vilib>:"NIMS_Get Row Vector_w Error - Matrix.vi"("A"=w506) -> ("Error Enum"=w500:T1, "Row Vector"=w505:T2[])  [unwired: 8 in, 1 out]
                  n217 = call <vilib>:"NIMS_CH_Character RV to String.vi"("Character array"=w505) -> ("String"=w507:string)  [unwired: 10 in]
                  n218 = call <vilib>:"NIMS_String to Enum.vi"("Input String"=w507, "Enum choices"=string[] ["notch", "peak"] ("Enum Options")) -> ("Error Enum"=w499:T1, "Enum Index"=w508:i32)  [unwired: 8 in]
                  n219 = call <vilib>:"NIMS_CH_Character 2D to U8 2D.vi"("Character 2D array"=w511) -> ("U8 2D array"=w510:u8[][])  [unwired: 10 in]
                  n220 = To Double Precision Float(number=w510) -> (double precision float=w509:dbl[][])
                  n221 = call-generic <vilib>:"NIMS_Get Scalar_w Error.vi"("A"=w509) -> ("Error Enum"=w501:T1, "Scalar"=w512:dbl)  [unwired: 8 in, 1 out]
                  n222 = call-generic <vilib>:"NIMS_Complex To Real.vi"("A"=w515) -> ("Error Enum"=w503:T1, "Real(A)"=w514:dbl[][])  [unwired: 8 in, 1 out]
                  n223 = To Long Integer(number=w514) -> (32bit integer=w513:i32[][])
                  n224 = call-generic <vilib>:"NIMS_Get Scalar_w Error.vi"("A"=w513) -> ("Error Enum"=w502:T1, "Scalar"=w516:i32)  [unwired: 8 in, 1 out]
                  n225 = call <vilib>:"NIMS_DF_iir_comb(n, bw, t).vi"("type"=w508, "bw"=w512, "n"=w516) -> ("error"=w498:i32, "b"=w489:dbl[])  [unwired: 6 in, 1 out]
                  n226 = Build Array(w492, w492, w492, w492, w492, "iir_comb") -> (w495:string[])
                  n227 = Build Array(w503, w502, w501, w500, w499, w498) -> (w496:i32[])
                  n228 = call <vilib>:"NIMS_Create Error From Enums.vi"("Error Code"=bool[] [FALSE, FALSE, FALSE, FALSE, FALSE, TRUE], "error in (no error)"=w494, "Line no"=w497, "Error Enums"=w496, "Function names"=w495) -> ("error out"=w490:errorcluster)  [unwired: 6 in]
                }
                frame "_Char:Character;;;" {
                  w520 = "iir_comb"
                  n229 = call-generic <vilib>:"NIMS_Complex To Real.vi"("A"=w533) -> ("Error Enum"=w528:T1, "Real(A)"=w532:dbl[][])  [unwired: 8 in, 1 out]
                  n230 = call-generic <vilib>:"NIMS_Get Scalar_w Error.vi"("A"=w532) -> ("Error Enum"=w527:T1, "Scalar"=w534:dbl)  [unwired: 8 in, 1 out]
                  n231 = call-generic <vilib>:"NIMS_Complex To Real.vi"("A"=w536) -> ("Error Enum"=w530:T1, "Real(A)"=w535:dbl[][])  [unwired: 8 in, 1 out]
                  n232 = call-generic <vilib>:"NIMS_Get Scalar_w Error.vi"("A"=w535) -> ("Error Enum"=w529:T1, "Scalar"=w537:dbl)  [unwired: 8 in, 1 out]
                  n233 = call <vilib>:"NIMS_CH_Character 2D to U8 2D.vi"("Character 2D array"=w540) -> ("U8 2D array"=w539:u8[][])  [unwired: 10 in]
                  n234 = To Long Integer(number=w539) -> (32bit integer=w538:i32[][])
                  n235 = call-generic <vilib>:"NIMS_Get Scalar_w Error.vi"("A"=w538) -> ("Error Enum"=w531:T1, "Scalar"=w541:i32)  [unwired: 8 in, 1 out]
                  n236 = call <vilib>:"NIMS_DF_iir_comb(n, bw, ab, t).vi"("ab"=w534, "bw"=w537, "n"=w541) -> ("error"=w526:i32, "b"=w517:dbl[])  [unwired: 6 in, 1 out]
                  n237 = Build Array(w520, w520, w520, w520, w520, "iir_comb") -> (w523:string[])
                  n238 = Build Array(w531, w530, w529, w528, w527, w526) -> (w524:i32[])
                  n239 = call <vilib>:"NIMS_Create Error From Enums.vi"("Error Code"=bool[] [FALSE, FALSE, FALSE, FALSE, FALSE, TRUE], "error in (no error)"=w522, "Line no"=w525, "Error Enums"=w524, "Function names"=w523) -> ("error out"=w518:errorcluster)  [unwired: 6 in]
                }
                frame "_Char:Character;;_Char:Character;" {
                  w545 = "iir_comb"
                  n240 = call-generic <vilib>:"NIMS_Get Row Vector_w Error - Matrix.vi"("A"=w559) -> ("Error Enum"=w553:T1, "Row Vector"=w558:T2[])  [unwired: 8 in, 1 out]
                  n241 = call <vilib>:"NIMS_CH_Character RV to String.vi"("Character array"=w558) -> ("String"=w560:string)  [unwired: 10 in]
                  n242 = call <vilib>:"NIMS_String to Enum.vi"("Input String"=w560, "Enum choices"=string[] ["notch", "peak"] ("Enum Options")) -> ("Error Enum"=w552:T1, "Enum Index"=w561:i32)  [unwired: 8 in]
                  n243 = call-generic <vilib>:"NIMS_Complex To Real.vi"("A"=w563) -> ("Error Enum"=w555:T1, "Real(A)"=w562:dbl[][])  [unwired: 8 in, 1 out]
                  n244 = call-generic <vilib>:"NIMS_Get Scalar_w Error.vi"("A"=w562) -> ("Error Enum"=w554:T1, "Scalar"=w564:dbl)  [unwired: 8 in, 1 out]
                  n245 = call <vilib>:"NIMS_CH_Character 2D to U8 2D.vi"("Character 2D array"=w567) -> ("U8 2D array"=w566:u8[][])  [unwired: 10 in]
                  n246 = To Long Integer(number=w566) -> (32bit integer=w565:i32[][])
                  n247 = call-generic <vilib>:"NIMS_Get Scalar_w Error.vi"("A"=w565) -> ("Error Enum"=w556:T1, "Scalar"=w568:i32)  [unwired: 8 in, 1 out]
                  n248 = call <vilib>:"NIMS_DF_iir_comb(n, bw, t).vi"("type"=w561, "bw"=w564, "n"=w568) -> ("error"=w551:i32, "b"=w542:dbl[])  [unwired: 6 in, 1 out]
                  n249 = Build Array(w545, w545, w545, w545, w545, "iir_comb") -> (w548:string[])
                  n250 = Build Array(w556, w555, w554, w553, w552, w551) -> (w549:i32[])
                  n251 = call <vilib>:"NIMS_Create Error From Enums.vi"("Error Code"=bool[] [FALSE, FALSE, FALSE, FALSE, FALSE, TRUE], "error in (no error)"=w547, "Line no"=w550, "Error Enums"=w549, "Function names"=w548) -> ("error out"=w543:errorcluster)  [unwired: 6 in]
                }
                frame "_Char:Character;_Char:Character;;" {
                  w572 = "iir_comb"
                  n252 = call-generic <vilib>:"NIMS_Complex To Real.vi"("A"=w584) -> ("Error Enum"=w580:T1, "Real(A)"=w583:dbl[][])  [unwired: 8 in, 1 out]
                  n253 = call-generic <vilib>:"NIMS_Get Scalar_w Error.vi"("A"=w583) -> ("Error Enum"=w579:T1, "Scalar"=w585:dbl)  [unwired: 8 in, 1 out]
                  n254 = call <vilib>:"NIMS_CH_Character 2D to U8 2D.vi"("Character 2D array"=w588) -> ("U8 2D array"=w587:u8[][])  [unwired: 10 in]
                  n255 = To Double Precision Float(number=w587) -> (double precision float=w586:dbl[][])
                  n256 = call-generic <vilib>:"NIMS_Get Scalar_w Error.vi"("A"=w586) -> ("Error Enum"=w581:T1, "Scalar"=w589:dbl)  [unwired: 8 in, 1 out]
                  n257 = call <vilib>:"NIMS_CH_Character 2D to U8 2D.vi"("Character 2D array"=w592) -> ("U8 2D array"=w591:u8[][])  [unwired: 10 in]
                  n258 = To Long Integer(number=w591) -> (32bit integer=w590:i32[][])
                  n259 = call-generic <vilib>:"NIMS_Get Scalar_w Error.vi"("A"=w590) -> ("Error Enum"=w582:T1, "Scalar"=w593:i32)  [unwired: 8 in, 1 out]
                  n260 = call <vilib>:"NIMS_DF_iir_comb(n, bw, ab, t).vi"("ab"=w585, "bw"=w589, "n"=w593) -> ("error"=w578:i32, "b"=w569:dbl[])  [unwired: 6 in, 1 out]
                  n261 = Build Array(w572, w572, w572, w572, "iir_comb") -> (w575:string[])
                  n262 = Build Array(w582, w581, w580, w579, w578) -> (w576:i32[])
                  n263 = call <vilib>:"NIMS_Create Error From Enums.vi"("Error Code"=bool[] [FALSE, FALSE, FALSE, FALSE, TRUE], "error in (no error)"=w574, "Line no"=w577, "Error Enums"=w576, "Function names"=w575) -> ("error out"=w570:errorcluster)  [unwired: 6 in]
                }
                frame "_Char:Character;_Char:Character;_Char:Character;" {
                  w597 = "iir_comb"
                  n264 = call-generic <vilib>:"NIMS_Get Row Vector_w Error - Matrix.vi"("A"=w610) -> ("Error Enum"=w605:T1, "Row Vector"=w609:T2[])  [unwired: 8 in, 1 out]
                  n265 = call <vilib>:"NIMS_CH_Character RV to String.vi"("Character array"=w609) -> ("String"=w611:string)  [unwired: 10 in]
                  n266 = call <vilib>:"NIMS_String to Enum.vi"("Input String"=w611, "Enum choices"=string[] ["notch", "peak"] ("Enum Options")) -> ("Error Enum"=w604:T1, "Enum Index"=w612:i32)  [unwired: 8 in]
                  n267 = call <vilib>:"NIMS_CH_Character 2D to U8 2D.vi"("Character 2D array"=w615) -> ("U8 2D array"=w614:u8[][])  [unwired: 10 in]
                  n268 = To Double Precision Float(number=w614) -> (double precision float=w613:dbl[][])
                  n269 = call-generic <vilib>:"NIMS_Get Scalar_w Error.vi"("A"=w613) -> ("Error Enum"=w606:T1, "Scalar"=w616:dbl)  [unwired: 8 in, 1 out]
                  n270 = call <vilib>:"NIMS_CH_Character 2D to U8 2D.vi"("Character 2D array"=w619) -> ("U8 2D array"=w618:u8[][])  [unwired: 10 in]
                  n271 = To Long Integer(number=w618) -> (32bit integer=w617:i32[][])
                  n272 = call-generic <vilib>:"NIMS_Get Scalar_w Error.vi"("A"=w617) -> ("Error Enum"=w607:T1, "Scalar"=w620:i32)  [unwired: 8 in, 1 out]
                  n273 = call <vilib>:"NIMS_DF_iir_comb(n, bw, t).vi"("type"=w612, "bw"=w616, "n"=w620) -> ("error"=w603:i32, "b"=w594:dbl[])  [unwired: 6 in, 1 out]
                  n274 = Build Array(w597, w597, w597, w597, "iir_comb") -> (w600:string[])
                  n275 = Build Array(w607, w606, w605, w604, w603) -> (w601:i32[])
                  n276 = call <vilib>:"NIMS_Create Error From Enums.vi"("Error Code"=bool[] [FALSE, FALSE, FALSE, FALSE, TRUE], "error in (no error)"=w599, "Line no"=w602, "Error Enums"=w601, "Function names"=w600) -> ("error out"=w595:errorcluster)  [unwired: 6 in]
                }
              }
              n277 = Build Array(w383) -> (w382:dbl[][])
              n278 = To Double Precision Complex(1:w382) -> (0:w381:cdb[][])
              n279 = call-generic <vilib>:"NIMS_RunTimeType_From StrictType (excl LVString).vi"("Plug-In Name"="", "Data In"=w381) -> ("Data Out"=w379:variant)  [unwired: 2 in]
              n280 = Build Array(w379) -> (w378:variant[])
            }
            frame 1 {
              n281 = Index Array(array=w646) -> (element #1=w642:variant, element #2=w637:variant, element #3=w632:variant)  [unwired: 3 in]
              n282 = call <vilib>:"NIMS_RunTimeType_Get Case Value.vi"("Data In"=w632) -> ("Case Value"=w628:string)  [unwired: 9 in, 1 out]
              n283 = call <vilib>:"NIMS_CH_RunTimeType_To Character 2D.vi"("Variant"=w632) -> ("data"=w629:T2[][])  [unwired: 1 in]
              n284 = call-generic <vilib>:"NIMS_RunTimeType_To Numeric.vi"("DataType"=cdb[][] [], "Variant"=w632) -> ("data"=w630:cdb[][])  [unwired: 1 in]
              n285 = call <vilib>:"NIMS_RunTimeType_Get Case Value.vi"("Data In"=w637) -> ("Case Value"=w633:string)  [unwired: 9 in, 1 out]
              n286 = call <vilib>:"NIMS_CH_RunTimeType_To Character 2D.vi"("Variant"=w637) -> ("data"=w634:T2[][])  [unwired: 1 in]
              n287 = call-generic <vilib>:"NIMS_RunTimeType_To Numeric.vi"("DataType"=cdb[][] [], "Variant"=w637) -> ("data"=w635:cdb[][])  [unwired: 1 in]
              n288 = call <vilib>:"NIMS_RunTimeType_Get Case Value.vi"("Data In"=w642) -> ("Case Value"=w638:string)  [unwired: 9 in, 1 out]
              n289 = call <vilib>:"NIMS_CH_RunTimeType_To Character 2D.vi"("Variant"=w642) -> ("data"=w639:T2[][])  [unwired: 1 in]
              n290 = call-generic <vilib>:"NIMS_RunTimeType_To Numeric.vi"("DataType"=cdb[][] [], "Variant"=w642) -> ("data"=w640:cdb[][])  [unwired: 1 in]
              n291 = Concatenate Strings(w638, w633, w628) -> (w644:string)
              n292 = case shown="\"_Char:Character;_Char:Character;_Char:Character;\"" w644 {
                tunnel: w643 -> [w648 w657 w683 w711 w737 w765 w790 w817 w842]
                tunnel: [_ w652 w678 w706 w732 w760 w785 w812 w837] -> w626
                tunnel: [w647 w653 w679 w707 w733 w761 w786 w813 w838] -> w627
                tunnel: w640 -> [_ w676 w704 w730 w758 _ _ _ _]
                tunnel: w639 -> [_ _ _ _ _ w783 w810 w835 w862]
                tunnel: w635 -> [_ w672 w700 _ _ w779 w806 _ _]
                tunnel: w634 -> [_ _ _ w726 w754 _ _ w831 w858]
                tunnel: w630 -> [_ w669 _ w722 _ w776 _ w827 _]
                tunnel: w629 -> [_ _ w696 _ w749 _ w802 _ w853]
                tunnel: w645 -> [w651 w660 w686 w714 w740 w768 w793 w820 w845]
                frame Default {
                  n293 = call <vilib>:"Create Error.vi"("Function name"="iir_comb", "error in (no error)"=w648, "Error Enum"=23, "Line number"=w651) -> ("error out"=w647:errorcluster)  [unwired: 6 in, 1 out]
                }
                frame ";;;" {
                  w655 = "iir_comb"
                  n294 = call-generic <vilib>:"NIMS_Complex To Real.vi"("A"=w669) -> ("Error Enum"=w663:T1, "Real(A)"=w668:dbl[][])  [unwired: 8 in, 1 out]
                  n295 = call-generic <vilib>:"NIMS_Get Scalar_w Error.vi"("A"=w668) -> ("Error Enum"=w662:T1, "Scalar"=w670:dbl)  [unwired: 8 in, 1 out]
                  n296 = call-generic <vilib>:"NIMS_Complex To Real.vi"("A"=w672) -> ("Error Enum"=w665:T1, "Real(A)"=w671:dbl[][])  [unwired: 8 in, 1 out]
                  n297 = call-generic <vilib>:"NIMS_Get Scalar_w Error.vi"("A"=w671) -> ("Error Enum"=w664:T1, "Scalar"=w673:dbl)  [unwired: 8 in, 1 out]
                  n298 = call-generic <vilib>:"NIMS_Complex To Real.vi"("A"=w676) -> ("Error Enum"=w667:T1, "Real(A)"=w675:dbl[][])  [unwired: 8 in, 1 out]
                  n299 = To Long Integer(number=w675) -> (32bit integer=w674:i32[][])
                  n300 = call-generic <vilib>:"NIMS_Get Scalar_w Error.vi"("A"=w674) -> ("Error Enum"=w666:T1, "Scalar"=w677:i32)  [unwired: 8 in, 1 out]
                  n301 = call <vilib>:"NIMS_DF_iir_comb(n, bw, ab, t).vi"("ab"=w670, "bw"=w673, "n"=w677) -> ("error"=w661:i32, "b"=w652:dbl[])  [unwired: 6 in, 1 out]
                  n302 = Build Array(w655, w655, w655, w655, w655, w655, "iir_comb") -> (w658:string[])
                  n303 = Build Array(w667, w666, w665, w664, w663, w662, w661) -> (w659:i32[])
                  n304 = call <vilib>:"NIMS_Create Error From Enums.vi"("Error Code"=bool[] [FALSE, FALSE, FALSE, FALSE, FALSE, FALSE, TRUE], "error in (no error)"=w657, "Line no"=w660, "Error Enums"=w659, "Function names"=w658) -> ("error out"=w653:errorcluster)  [unwired: 6 in]
                }
                frame ";;_Char:Character;" {
                  w681 = "iir_comb"
                  n305 = call-generic <vilib>:"NIMS_Get Row Vector_w Error - Matrix.vi"("A"=w696) -> ("Error Enum"=w689:T1, "Row Vector"=w695:T2[])  [unwired: 8 in, 1 out]
                  n306 = call <vilib>:"NIMS_CH_Character RV to String.vi"("Character array"=w695) -> ("String"=w697:string)  [unwired: 10 in]
                  n307 = call <vilib>:"NIMS_String to Enum.vi"("Input String"=w697, "Enum choices"=string[] ["notch", "peak"] ("Enum Options")) -> ("Error Enum"=w688:T1, "Enum Index"=w698:i32)  [unwired: 8 in]
                  n308 = call-generic <vilib>:"NIMS_Complex To Real.vi"("A"=w700) -> ("Error Enum"=w691:T1, "Real(A)"=w699:dbl[][])  [unwired: 8 in, 1 out]
                  n309 = call-generic <vilib>:"NIMS_Get Scalar_w Error.vi"("A"=w699) -> ("Error Enum"=w690:T1, "Scalar"=w701:dbl)  [unwired: 8 in, 1 out]
                  n310 = call-generic <vilib>:"NIMS_Complex To Real.vi"("A"=w704) -> ("Error Enum"=w693:T1, "Real(A)"=w703:dbl[][])  [unwired: 8 in, 1 out]
                  n311 = To Long Integer(number=w703) -> (32bit integer=w702:i32[][])
                  n312 = call-generic <vilib>:"NIMS_Get Scalar_w Error.vi"("A"=w702) -> ("Error Enum"=w692:T1, "Scalar"=w705:i32)  [unwired: 8 in, 1 out]
                  n313 = call <vilib>:"NIMS_DF_iir_comb(n, bw, t).vi"("type"=w698, "bw"=w701, "n"=w705) -> ("error"=w687:i32, "b"=w678:dbl[])  [unwired: 6 in, 1 out]
                  n314 = Build Array(w681, w681, w681, w681, w681, w681, "iir_comb") -> (w684:string[])
                  n315 = Build Array(w693, w692, w691, w690, w689, w688, w687) -> (w685:i32[])
                  n316 = call <vilib>:"NIMS_Create Error From Enums.vi"("Error Code"=bool[] [FALSE, FALSE, FALSE, FALSE, FALSE, FALSE, TRUE], "error in (no error)"=w683, "Line no"=w686, "Error Enums"=w685, "Function names"=w684) -> ("error out"=w679:errorcluster)  [unwired: 6 in]
                }
                frame ";_Char:Character;;" {
                  w709 = "iir_comb"
                  n317 = call-generic <vilib>:"NIMS_Complex To Real.vi"("A"=w722) -> ("Error Enum"=w717:T1, "Real(A)"=w721:dbl[][])  [unwired: 8 in, 1 out]
                  n318 = call-generic <vilib>:"NIMS_Get Scalar_w Error.vi"("A"=w721) -> ("Error Enum"=w716:T1, "Scalar"=w723:dbl)  [unwired: 8 in, 1 out]
                  n319 = call <vilib>:"NIMS_CH_Character 2D to U8 2D.vi"("Character 2D array"=w726) -> ("U8 2D array"=w725:u8[][])  [unwired: 10 in]
                  n320 = To Double Precision Float(number=w725) -> (double precision float=w724:dbl[][])
                  n321 = call-generic <vilib>:"NIMS_Get Scalar_w Error.vi"("A"=w724) -> ("Error Enum"=w718:T1, "Scalar"=w727:dbl)  [unwired: 8 in, 1 out]
                  n322 = call-generic <vilib>:"NIMS_Complex To Real.vi"("A"=w730) -> ("Error Enum"=w720:T1, "Real(A)"=w729:dbl[][])  [unwired: 8 in, 1 out]
                  n323 = To Long Integer(number=w729) -> (32bit integer=w728:i32[][])
                  n324 = call-generic <vilib>:"NIMS_Get Scalar_w Error.vi"("A"=w728) -> ("Error Enum"=w719:T1, "Scalar"=w731:i32)  [unwired: 8 in, 1 out]
                  n325 = call <vilib>:"NIMS_DF_iir_comb(n, bw, ab, t).vi"("ab"=w723, "bw"=w727, "n"=w731) -> ("error"=w715:i32, "b"=w706:dbl[])  [unwired: 6 in, 1 out]
                  n326 = Build Array(w709, w709, w709, w709, w709, "iir_comb") -> (w712:string[])
                  n327 = Build Array(w720, w719, w718, w717, w716, w715) -> (w713:i32[])
                  n328 = call <vilib>:"NIMS_Create Error From Enums.vi"("Error Code"=bool[] [FALSE, FALSE, FALSE, FALSE, FALSE, TRUE], "error in (no error)"=w711, "Line no"=w714, "Error Enums"=w713, "Function names"=w712) -> ("error out"=w707:errorcluster)  [unwired: 6 in]
                }
                frame ";_Char:Character;_Char:Character;" {
                  w735 = "iir_comb"
                  n329 = call-generic <vilib>:"NIMS_Get Row Vector_w Error - Matrix.vi"("A"=w749) -> ("Error Enum"=w743:T1, "Row Vector"=w748:T2[])  [unwired: 8 in, 1 out]
                  n330 = call <vilib>:"NIMS_CH_Character RV to String.vi"("Character array"=w748) -> ("String"=w750:string)  [unwired: 10 in]
                  n331 = call <vilib>:"NIMS_String to Enum.vi"("Input String"=w750, "Enum choices"=string[] ["notch", "peak"] ("Enum Options")) -> ("Error Enum"=w742:T1, "Enum Index"=w751:i32)  [unwired: 8 in]
                  n332 = call <vilib>:"NIMS_CH_Character 2D to U8 2D.vi"("Character 2D array"=w754) -> ("U8 2D array"=w753:u8[][])  [unwired: 10 in]
                  n333 = To Double Precision Float(number=w753) -> (double precision float=w752:dbl[][])
                  n334 = call-generic <vilib>:"NIMS_Get Scalar_w Error.vi"("A"=w752) -> ("Error Enum"=w744:T1, "Scalar"=w755:dbl)  [unwired: 8 in, 1 out]
                  n335 = call-generic <vilib>:"NIMS_Complex To Real.vi"("A"=w758) -> ("Error Enum"=w746:T1, "Real(A)"=w757:dbl[][])  [unwired: 8 in, 1 out]
                  n336 = To Long Integer(number=w757) -> (32bit integer=w756:i32[][])
                  n337 = call-generic <vilib>:"NIMS_Get Scalar_w Error.vi"("A"=w756) -> ("Error Enum"=w745:T1, "Scalar"=w759:i32)  [unwired: 8 in, 1 out]
                  n338 = call <vilib>:"NIMS_DF_iir_comb(n, bw, t).vi"("type"=w751, "bw"=w755, "n"=w759) -> ("error"=w741:i32, "b"=w732:dbl[])  [unwired: 6 in, 1 out]
                  n339 = Build Array(w735, w735, w735, w735, w735, "iir_comb") -> (w738:string[])
                  n340 = Build Array(w746, w745, w744, w743, w742, w741) -> (w739:i32[])
                  n341 = call <vilib>:"NIMS_Create Error From Enums.vi"("Error Code"=bool[] [FALSE, FALSE, FALSE, FALSE, FALSE, TRUE], "error in (no error)"=w737, "Line no"=w740, "Error Enums"=w739, "Function names"=w738) -> ("error out"=w733:errorcluster)  [unwired: 6 in]
                }
                frame "_Char:Character;;;" {
                  w763 = "iir_comb"
                  n342 = call-generic <vilib>:"NIMS_Complex To Real.vi"("A"=w776) -> ("Error Enum"=w771:T1, "Real(A)"=w775:dbl[][])  [unwired: 8 in, 1 out]
                  n343 = call-generic <vilib>:"NIMS_Get Scalar_w Error.vi"("A"=w775) -> ("Error Enum"=w770:T1, "Scalar"=w777:dbl)  [unwired: 8 in, 1 out]
                  n344 = call-generic <vilib>:"NIMS_Complex To Real.vi"("A"=w779) -> ("Error Enum"=w773:T1, "Real(A)"=w778:dbl[][])  [unwired: 8 in, 1 out]
                  n345 = call-generic <vilib>:"NIMS_Get Scalar_w Error.vi"("A"=w778) -> ("Error Enum"=w772:T1, "Scalar"=w780:dbl)  [unwired: 8 in, 1 out]
                  n346 = call <vilib>:"NIMS_CH_Character 2D to U8 2D.vi"("Character 2D array"=w783) -> ("U8 2D array"=w782:u8[][])  [unwired: 10 in]
                  n347 = To Long Integer(number=w782) -> (32bit integer=w781:i32[][])
                  n348 = call-generic <vilib>:"NIMS_Get Scalar_w Error.vi"("A"=w781) -> ("Error Enum"=w774:T1, "Scalar"=w784:i32)  [unwired: 8 in, 1 out]
                  n349 = call <vilib>:"NIMS_DF_iir_comb(n, bw, ab, t).vi"("ab"=w777, "bw"=w780, "n"=w784) -> ("error"=w769:i32, "b"=w760:dbl[])  [unwired: 6 in, 1 out]
                  n350 = Build Array(w763, w763, w763, w763, w763, "iir_comb") -> (w766:string[])
                  n351 = Build Array(w774, w773, w772, w771, w770, w769) -> (w767:i32[])
                  n352 = call <vilib>:"NIMS_Create Error From Enums.vi"("Error Code"=bool[] [FALSE, FALSE, FALSE, FALSE, FALSE, TRUE], "error in (no error)"=w765, "Line no"=w768, "Error Enums"=w767, "Function names"=w766) -> ("error out"=w761:errorcluster)  [unwired: 6 in]
                }
                frame "_Char:Character;;_Char:Character;" {
                  w788 = "iir_comb"
                  n353 = call-generic <vilib>:"NIMS_Get Row Vector_w Error - Matrix.vi"("A"=w802) -> ("Error Enum"=w796:T1, "Row Vector"=w801:T2[])  [unwired: 8 in, 1 out]
                  n354 = call <vilib>:"NIMS_CH_Character RV to String.vi"("Character array"=w801) -> ("String"=w803:string)  [unwired: 10 in]
                  n355 = call <vilib>:"NIMS_String to Enum.vi"("Input String"=w803, "Enum choices"=string[] ["notch", "peak"] ("Enum Options")) -> ("Error Enum"=w795:T1, "Enum Index"=w804:i32)  [unwired: 8 in]
                  n356 = call-generic <vilib>:"NIMS_Complex To Real.vi"("A"=w806) -> ("Error Enum"=w798:T1, "Real(A)"=w805:dbl[][])  [unwired: 8 in, 1 out]
                  n357 = call-generic <vilib>:"NIMS_Get Scalar_w Error.vi"("A"=w805) -> ("Error Enum"=w797:T1, "Scalar"=w807:dbl)  [unwired: 8 in, 1 out]
                  n358 = call <vilib>:"NIMS_CH_Character 2D to U8 2D.vi"("Character 2D array"=w810) -> ("U8 2D array"=w809:u8[][])  [unwired: 10 in]
                  n359 = To Long Integer(number=w809) -> (32bit integer=w808:i32[][])
                  n360 = call-generic <vilib>:"NIMS_Get Scalar_w Error.vi"("A"=w808) -> ("Error Enum"=w799:T1, "Scalar"=w811:i32)  [unwired: 8 in, 1 out]
                  n361 = call <vilib>:"NIMS_DF_iir_comb(n, bw, t).vi"("type"=w804, "bw"=w807, "n"=w811) -> ("error"=w794:i32, "b"=w785:dbl[])  [unwired: 6 in, 1 out]
                  n362 = Build Array(w788, w788, w788, w788, w788, "iir_comb") -> (w791:string[])
                  n363 = Build Array(w799, w798, w797, w796, w795, w794) -> (w792:i32[])
                  n364 = call <vilib>:"NIMS_Create Error From Enums.vi"("Error Code"=bool[] [FALSE, FALSE, FALSE, FALSE, FALSE, TRUE], "error in (no error)"=w790, "Line no"=w793, "Error Enums"=w792, "Function names"=w791) -> ("error out"=w786:errorcluster)  [unwired: 6 in]
                }
                frame "_Char:Character;_Char:Character;;" {
                  w815 = "iir_comb"
                  n365 = call-generic <vilib>:"NIMS_Complex To Real.vi"("A"=w827) -> ("Error Enum"=w823:T1, "Real(A)"=w826:dbl[][])  [unwired: 8 in, 1 out]
                  n366 = call-generic <vilib>:"NIMS_Get Scalar_w Error.vi"("A"=w826) -> ("Error Enum"=w822:T1, "Scalar"=w828:dbl)  [unwired: 8 in, 1 out]
                  n367 = call <vilib>:"NIMS_CH_Character 2D to U8 2D.vi"("Character 2D array"=w831) -> ("U8 2D array"=w830:u8[][])  [unwired: 10 in]
                  n368 = To Double Precision Float(number=w830) -> (double precision float=w829:dbl[][])
                  n369 = call-generic <vilib>:"NIMS_Get Scalar_w Error.vi"("A"=w829) -> ("Error Enum"=w824:T1, "Scalar"=w832:dbl)  [unwired: 8 in, 1 out]
                  n370 = call <vilib>:"NIMS_CH_Character 2D to U8 2D.vi"("Character 2D array"=w835) -> ("U8 2D array"=w834:u8[][])  [unwired: 10 in]
                  n371 = To Long Integer(number=w834) -> (32bit integer=w833:i32[][])
                  n372 = call-generic <vilib>:"NIMS_Get Scalar_w Error.vi"("A"=w833) -> ("Error Enum"=w825:T1, "Scalar"=w836:i32)  [unwired: 8 in, 1 out]
                  n373 = call <vilib>:"NIMS_DF_iir_comb(n, bw, ab, t).vi"("ab"=w828, "bw"=w832, "n"=w836) -> ("error"=w821:i32, "b"=w812:dbl[])  [unwired: 6 in, 1 out]
                  n374 = Build Array(w815, w815, w815, w815, "iir_comb") -> (w818:string[])
                  n375 = Build Array(w825, w824, w823, w822, w821) -> (w819:i32[])
                  n376 = call <vilib>:"NIMS_Create Error From Enums.vi"("Error Code"=bool[] [FALSE, FALSE, FALSE, FALSE, TRUE], "error in (no error)"=w817, "Line no"=w820, "Error Enums"=w819, "Function names"=w818) -> ("error out"=w813:errorcluster)  [unwired: 6 in]
                }
                frame "_Char:Character;_Char:Character;_Char:Character;" {
                  w840 = "iir_comb"
                  n377 = call-generic <vilib>:"NIMS_Get Row Vector_w Error - Matrix.vi"("A"=w853) -> ("Error Enum"=w848:T1, "Row Vector"=w852:T2[])  [unwired: 8 in, 1 out]
                  n378 = call <vilib>:"NIMS_CH_Character RV to String.vi"("Character array"=w852) -> ("String"=w854:string)  [unwired: 10 in]
                  n379 = call <vilib>:"NIMS_String to Enum.vi"("Input String"=w854, "Enum choices"=string[] ["notch", "peak"] ("Enum Options")) -> ("Error Enum"=w847:T1, "Enum Index"=w855:i32)  [unwired: 8 in]
                  n380 = call <vilib>:"NIMS_CH_Character 2D to U8 2D.vi"("Character 2D array"=w858) -> ("U8 2D array"=w857:u8[][])  [unwired: 10 in]
                  n381 = To Double Precision Float(number=w857) -> (double precision float=w856:dbl[][])
                  n382 = call-generic <vilib>:"NIMS_Get Scalar_w Error.vi"("A"=w856) -> ("Error Enum"=w849:T1, "Scalar"=w859:dbl)  [unwired: 8 in, 1 out]
                  n383 = call <vilib>:"NIMS_CH_Character 2D to U8 2D.vi"("Character 2D array"=w862) -> ("U8 2D array"=w861:u8[][])  [unwired: 10 in]
                  n384 = To Long Integer(number=w861) -> (32bit integer=w860:i32[][])
                  n385 = call-generic <vilib>:"NIMS_Get Scalar_w Error.vi"("A"=w860) -> ("Error Enum"=w850:T1, "Scalar"=w863:i32)  [unwired: 8 in, 1 out]
                  n386 = call <vilib>:"NIMS_DF_iir_comb(n, bw, t).vi"("type"=w855, "bw"=w859, "n"=w863) -> ("error"=w846:i32, "b"=w837:dbl[])  [unwired: 6 in, 1 out]
                  n387 = Build Array(w840, w840, w840, w840, "iir_comb") -> (w843:string[])
                  n388 = Build Array(w850, w849, w848, w847, w846) -> (w844:i32[])
                  n389 = call <vilib>:"NIMS_Create Error From Enums.vi"("Error Code"=bool[] [FALSE, FALSE, FALSE, FALSE, TRUE], "error in (no error)"=w842, "Line no"=w845, "Error Enums"=w844, "Function names"=w843) -> ("error out"=w838:errorcluster)  [unwired: 6 in]
                }
              }
              n390 = Build Array(w626) -> (w625:dbl[][])
              n391 = To Double Precision Complex(1:w625) -> (0:w624:cdb[][])
              n392 = call-generic <vilib>:"NIMS_RunTimeType_From StrictType (excl LVString).vi"("Plug-In Name"="", "Data In"=w624) -> ("Data Out"=w622:variant)  [unwired: 2 in]
              n393 = Build Array(w622) -> (w621:variant[])
            }
            frame 2 {
              n394 = Index Array(array=w894) -> (element #1=w890:variant, element #2=w885:variant, element #3=w880:variant)  [unwired: 3 in]
              n395 = call <vilib>:"NIMS_RunTimeType_Get Case Value.vi"("Data In"=w880) -> ("Case Value"=w876:string)  [unwired: 9 in, 1 out]
              n396 = call <vilib>:"NIMS_CH_RunTimeType_To Character 2D.vi"("Variant"=w880) -> ("data"=w877:T2[][])  [unwired: 1 in]
              n397 = call-generic <vilib>:"NIMS_RunTimeType_To Numeric.vi"("DataType"=cdb[][] [], "Variant"=w880) -> ("data"=w878:cdb[][])  [unwired: 1 in]
              n398 = call <vilib>:"NIMS_RunTimeType_Get Case Value.vi"("Data In"=w885) -> ("Case Value"=w881:string)  [unwired: 9 in, 1 out]
              n399 = call <vilib>:"NIMS_CH_RunTimeType_To Character 2D.vi"("Variant"=w885) -> ("data"=w882:T2[][])  [unwired: 1 in]
              n400 = call-generic <vilib>:"NIMS_RunTimeType_To Numeric.vi"("DataType"=cdb[][] [], "Variant"=w885) -> ("data"=w883:cdb[][])  [unwired: 1 in]
              n401 = call <vilib>:"NIMS_RunTimeType_Get Case Value.vi"("Data In"=w890) -> ("Case Value"=w886:string)  [unwired: 9 in, 1 out]
              n402 = call <vilib>:"NIMS_CH_RunTimeType_To Character 2D.vi"("Variant"=w890) -> ("data"=w887:T2[][])  [unwired: 1 in]
              n403 = call-generic <vilib>:"NIMS_RunTimeType_To Numeric.vi"("DataType"=cdb[][] [], "Variant"=w890) -> ("data"=w888:cdb[][])  [unwired: 1 in]
              n404 = Concatenate Strings(w886, w881, w876) -> (w892:string)
              n405 = case shown="\"_Char:Character;_Char:Character;_Char:Character;\"" w892 {
                tunnel: w891 -> [w896 w906 w933 w962 w989 w1018 w1044 w1072 w1098]
                tunnel: [_ w901 w928 w957 w984 w1013 w1039 w1067 w1093] -> w874
                tunnel: [_ w900 w927 w956 w983 w1012 w1038 w1066 w1092] -> w870
                tunnel: [w895 w902 w929 w958 w985 w1014 w1040 w1068 w1094] -> w875
                tunnel: w888 -> [_ w925 w954 w981 w1010 _ _ _ _]
                tunnel: w887 -> [_ _ _ _ _ w1036 w1064 w1090 w1118]
                tunnel: w883 -> [_ w921 w950 _ _ w1032 w1060 _ _]
                tunnel: w882 -> [_ _ _ w977 w1006 _ _ w1086 w1114]
                tunnel: w878 -> [_ w918 _ w973 _ w1029 _ w1082 _]
                tunnel: w877 -> [_ _ w946 _ w1001 _ w1056 _ w1109]
                tunnel: w893 -> [w899 w909 w936 w965 w992 w1021 w1047 w1075 w1101]
                frame Default {
                  n406 = call <vilib>:"Create Error.vi"("Function name"="iir_comb", "error in (no error)"=w896, "Error Enum"=23, "Line number"=w899) -> ("error out"=w895:errorcluster)  [unwired: 6 in, 1 out]
                }
                frame ";;;" {
                  w904 = "iir_comb"
                  n407 = call-generic <vilib>:"NIMS_Complex To Real.vi"("A"=w918) -> ("Error Enum"=w912:T1, "Real(A)"=w917:dbl[][])  [unwired: 8 in, 1 out]
                  n408 = call-generic <vilib>:"NIMS_Get Scalar_w Error.vi"("A"=w917) -> ("Error Enum"=w911:T1, "Scalar"=w919:dbl)  [unwired: 8 in, 1 out]
                  n409 = call-generic <vilib>:"NIMS_Complex To Real.vi"("A"=w921) -> ("Error Enum"=w914:T1, "Real(A)"=w920:dbl[][])  [unwired: 8 in, 1 out]
                  n410 = call-generic <vilib>:"NIMS_Get Scalar_w Error.vi"("A"=w920) -> ("Error Enum"=w913:T1, "Scalar"=w922:dbl)  [unwired: 8 in, 1 out]
                  n411 = call-generic <vilib>:"NIMS_Complex To Real.vi"("A"=w925) -> ("Error Enum"=w916:T1, "Real(A)"=w924:dbl[][])  [unwired: 8 in, 1 out]
                  n412 = To Long Integer(number=w924) -> (32bit integer=w923:i32[][])
                  n413 = call-generic <vilib>:"NIMS_Get Scalar_w Error.vi"("A"=w923) -> ("Error Enum"=w915:T1, "Scalar"=w926:i32)  [unwired: 8 in, 1 out]
                  n414 = call <vilib>:"NIMS_DF_iir_comb(n, bw, ab, t).vi"("ab"=w919, "bw"=w922, "n"=w926) -> ("error"=w910:i32, "a"=w900:dbl[], "b"=w901:dbl[])  [unwired: 6 in]
                  n415 = Build Array(w904, w904, w904, w904, w904, w904, "iir_comb") -> (w907:string[])
                  n416 = Build Array(w916, w915, w914, w913, w912, w911, w910) -> (w908:i32[])
                  n417 = call <vilib>:"NIMS_Create Error From Enums.vi"("Error Code"=bool[] [FALSE, FALSE, FALSE, FALSE, FALSE, FALSE, TRUE], "error in (no error)"=w906, "Line no"=w909, "Error Enums"=w908, "Function names"=w907) -> ("error out"=w902:errorcluster)  [unwired: 6 in]
                }
                frame ";;_Char:Character;" {
                  w931 = "iir_comb"
                  n418 = call-generic <vilib>:"NIMS_Get Row Vector_w Error - Matrix.vi"("A"=w946) -> ("Error Enum"=w939:T1, "Row Vector"=w945:T2[])  [unwired: 8 in, 1 out]
                  n419 = call <vilib>:"NIMS_CH_Character RV to String.vi"("Character array"=w945) -> ("String"=w947:string)  [unwired: 10 in]
                  n420 = call <vilib>:"NIMS_String to Enum.vi"("Input String"=w947, "Enum choices"=string[] ["notch", "peak"] ("Enum Options")) -> ("Error Enum"=w938:T1, "Enum Index"=w948:i32)  [unwired: 8 in]
                  n421 = call-generic <vilib>:"NIMS_Complex To Real.vi"("A"=w950) -> ("Error Enum"=w941:T1, "Real(A)"=w949:dbl[][])  [unwired: 8 in, 1 out]
                  n422 = call-generic <vilib>:"NIMS_Get Scalar_w Error.vi"("A"=w949) -> ("Error Enum"=w940:T1, "Scalar"=w951:dbl)  [unwired: 8 in, 1 out]
                  n423 = call-generic <vilib>:"NIMS_Complex To Real.vi"("A"=w954) -> ("Error Enum"=w943:T1, "Real(A)"=w953:dbl[][])  [unwired: 8 in, 1 out]
                  n424 = To Long Integer(number=w953) -> (32bit integer=w952:i32[][])
                  n425 = call-generic <vilib>:"NIMS_Get Scalar_w Error.vi"("A"=w952) -> ("Error Enum"=w942:T1, "Scalar"=w955:i32)  [unwired: 8 in, 1 out]
                  n426 = call <vilib>:"NIMS_DF_iir_comb(n, bw, t).vi"("type"=w948, "bw"=w951, "n"=w955) -> ("error"=w937:i32, "a"=w927:dbl[], "b"=w928:dbl[])  [unwired: 6 in]
                  n427 = Build Array(w931, w931, w931, w931, w931, w931, "iir_comb") -> (w934:string[])
                  n428 = Build Array(w943, w942, w941, w940, w939, w938, w937) -> (w935:i32[])
                  n429 = call <vilib>:"NIMS_Create Error From Enums.vi"("Error Code"=bool[] [FALSE, FALSE, FALSE, FALSE, FALSE, FALSE, TRUE], "error in (no error)"=w933, "Line no"=w936, "Error Enums"=w935, "Function names"=w934) -> ("error out"=w929:errorcluster)  [unwired: 6 in]
                }
                frame ";_Char:Character;;" {
                  w960 = "iir_comb"
                  n430 = call-generic <vilib>:"NIMS_Complex To Real.vi"("A"=w973) -> ("Error Enum"=w968:T1, "Real(A)"=w972:dbl[][])  [unwired: 8 in, 1 out]
                  n431 = call-generic <vilib>:"NIMS_Get Scalar_w Error.vi"("A"=w972) -> ("Error Enum"=w967:T1, "Scalar"=w974:dbl)  [unwired: 8 in, 1 out]
                  n432 = call <vilib>:"NIMS_CH_Character 2D to U8 2D.vi"("Character 2D array"=w977) -> ("U8 2D array"=w976:u8[][])  [unwired: 10 in]
                  n433 = To Double Precision Float(number=w976) -> (double precision float=w975:dbl[][])
                  n434 = call-generic <vilib>:"NIMS_Get Scalar_w Error.vi"("A"=w975) -> ("Error Enum"=w969:T1, "Scalar"=w978:dbl)  [unwired: 8 in, 1 out]
                  n435 = call-generic <vilib>:"NIMS_Complex To Real.vi"("A"=w981) -> ("Error Enum"=w971:T1, "Real(A)"=w980:dbl[][])  [unwired: 8 in, 1 out]
                  n436 = To Long Integer(number=w980) -> (32bit integer=w979:i32[][])
                  n437 = call-generic <vilib>:"NIMS_Get Scalar_w Error.vi"("A"=w979) -> ("Error Enum"=w970:T1, "Scalar"=w982:i32)  [unwired: 8 in, 1 out]
                  n438 = call <vilib>:"NIMS_DF_iir_comb(n, bw, ab, t).vi"("ab"=w974, "bw"=w978, "n"=w982) -> ("error"=w966:i32, "a"=w956:dbl[], "b"=w957:dbl[])  [unwired: 6 in]
                  n439 = Build Array(w960, w960, w960, w960, w960, "iir_comb") -> (w963:string[])
                  n440 = Build Array(w971, w970, w969, w968, w967, w966) -> (w964:i32[])
                  n441 = call <vilib>:"NIMS_Create Error From Enums.vi"("Error Code"=bool[] [FALSE, FALSE, FALSE, FALSE, FALSE, TRUE], "error in (no error)"=w962, "Line no"=w965, "Error Enums"=w964, "Function names"=w963) -> ("error out"=w958:errorcluster)  [unwired: 6 in]
                }
                frame ";_Char:Character;_Char:Character;" {
                  w987 = "iir_comb"
                  n442 = call-generic <vilib>:"NIMS_Get Row Vector_w Error - Matrix.vi"("A"=w1001) -> ("Error Enum"=w995:T1, "Row Vector"=w1000:T2[])  [unwired: 8 in, 1 out]
                  n443 = call <vilib>:"NIMS_CH_Character RV to String.vi"("Character array"=w1000) -> ("String"=w1002:string)  [unwired: 10 in]
                  n444 = call <vilib>:"NIMS_String to Enum.vi"("Input String"=w1002, "Enum choices"=string[] ["notch", "peak"] ("Enum Options")) -> ("Error Enum"=w994:T1, "Enum Index"=w1003:i32)  [unwired: 8 in]
                  n445 = call <vilib>:"NIMS_CH_Character 2D to U8 2D.vi"("Character 2D array"=w1006) -> ("U8 2D array"=w1005:u8[][])  [unwired: 10 in]
                  n446 = To Double Precision Float(number=w1005) -> (double precision float=w1004:dbl[][])
                  n447 = call-generic <vilib>:"NIMS_Get Scalar_w Error.vi"("A"=w1004) -> ("Error Enum"=w996:T1, "Scalar"=w1007:dbl)  [unwired: 8 in, 1 out]
                  n448 = call-generic <vilib>:"NIMS_Complex To Real.vi"("A"=w1010) -> ("Error Enum"=w998:T1, "Real(A)"=w1009:dbl[][])  [unwired: 8 in, 1 out]
                  n449 = To Long Integer(number=w1009) -> (32bit integer=w1008:i32[][])
                  n450 = call-generic <vilib>:"NIMS_Get Scalar_w Error.vi"("A"=w1008) -> ("Error Enum"=w997:T1, "Scalar"=w1011:i32)  [unwired: 8 in, 1 out]
                  n451 = call <vilib>:"NIMS_DF_iir_comb(n, bw, t).vi"("type"=w1003, "bw"=w1007, "n"=w1011) -> ("error"=w993:i32, "a"=w983:dbl[], "b"=w984:dbl[])  [unwired: 6 in]
                  n452 = Build Array(w987, w987, w987, w987, w987, "iir_comb") -> (w990:string[])
                  n453 = Build Array(w998, w997, w996, w995, w994, w993) -> (w991:i32[])
                  n454 = call <vilib>:"NIMS_Create Error From Enums.vi"("Error Code"=bool[] [FALSE, FALSE, FALSE, FALSE, FALSE, TRUE], "error in (no error)"=w989, "Line no"=w992, "Error Enums"=w991, "Function names"=w990) -> ("error out"=w985:errorcluster)  [unwired: 6 in]
                }
                frame "_Char:Character;;;" {
                  w1016 = "iir_comb"
                  n455 = call-generic <vilib>:"NIMS_Complex To Real.vi"("A"=w1029) -> ("Error Enum"=w1024:T1, "Real(A)"=w1028:dbl[][])  [unwired: 8 in, 1 out]
                  n456 = call-generic <vilib>:"NIMS_Get Scalar_w Error.vi"("A"=w1028) -> ("Error Enum"=w1023:T1, "Scalar"=w1030:dbl)  [unwired: 8 in, 1 out]
                  n457 = call-generic <vilib>:"NIMS_Complex To Real.vi"("A"=w1032) -> ("Error Enum"=w1026:T1, "Real(A)"=w1031:dbl[][])  [unwired: 8 in, 1 out]
                  n458 = call-generic <vilib>:"NIMS_Get Scalar_w Error.vi"("A"=w1031) -> ("Error Enum"=w1025:T1, "Scalar"=w1033:dbl)  [unwired: 8 in, 1 out]
                  n459 = call <vilib>:"NIMS_CH_Character 2D to U8 2D.vi"("Character 2D array"=w1036) -> ("U8 2D array"=w1035:u8[][])  [unwired: 10 in]
                  n460 = To Long Integer(number=w1035) -> (32bit integer=w1034:i32[][])
                  n461 = call-generic <vilib>:"NIMS_Get Scalar_w Error.vi"("A"=w1034) -> ("Error Enum"=w1027:T1, "Scalar"=w1037:i32)  [unwired: 8 in, 1 out]
                  n462 = call <vilib>:"NIMS_DF_iir_comb(n, bw, ab, t).vi"("ab"=w1030, "bw"=w1033, "n"=w1037) -> ("error"=w1022:i32, "a"=w1012:dbl[], "b"=w1013:dbl[])  [unwired: 6 in]
                  n463 = Build Array(w1016, w1016, w1016, w1016, w1016, "iir_comb") -> (w1019:string[])
                  n464 = Build Array(w1027, w1026, w1025, w1024, w1023, w1022) -> (w1020:i32[])
                  n465 = call <vilib>:"NIMS_Create Error From Enums.vi"("Error Code"=bool[] [FALSE, FALSE, FALSE, FALSE, FALSE, TRUE], "error in (no error)"=w1018, "Line no"=w1021, "Error Enums"=w1020, "Function names"=w1019) -> ("error out"=w1014:errorcluster)  [unwired: 6 in]
                }
                frame "_Char:Character;;_Char:Character;" {
                  w1042 = "iir_comb"
                  n466 = call-generic <vilib>:"NIMS_Get Row Vector_w Error - Matrix.vi"("A"=w1056) -> ("Error Enum"=w1050:T1, "Row Vector"=w1055:T2[])  [unwired: 8 in, 1 out]
                  n467 = call <vilib>:"NIMS_CH_Character RV to String.vi"("Character array"=w1055) -> ("String"=w1057:string)  [unwired: 10 in]
                  n468 = call <vilib>:"NIMS_String to Enum.vi"("Input String"=w1057, "Enum choices"=string[] ["notch", "peak"] ("Enum Options")) -> ("Error Enum"=w1049:T1, "Enum Index"=w1058:i32)  [unwired: 8 in]
                  n469 = call-generic <vilib>:"NIMS_Complex To Real.vi"("A"=w1060) -> ("Error Enum"=w1052:T1, "Real(A)"=w1059:dbl[][])  [unwired: 8 in, 1 out]
                  n470 = call-generic <vilib>:"NIMS_Get Scalar_w Error.vi"("A"=w1059) -> ("Error Enum"=w1051:T1, "Scalar"=w1061:dbl)  [unwired: 8 in, 1 out]
                  n471 = call <vilib>:"NIMS_CH_Character 2D to U8 2D.vi"("Character 2D array"=w1064) -> ("U8 2D array"=w1063:u8[][])  [unwired: 10 in]
                  n472 = To Long Integer(number=w1063) -> (32bit integer=w1062:i32[][])
                  n473 = call-generic <vilib>:"NIMS_Get Scalar_w Error.vi"("A"=w1062) -> ("Error Enum"=w1053:T1, "Scalar"=w1065:i32)  [unwired: 8 in, 1 out]
                  n474 = call <vilib>:"NIMS_DF_iir_comb(n, bw, t).vi"("type"=w1058, "bw"=w1061, "n"=w1065) -> ("error"=w1048:i32, "a"=w1038:dbl[], "b"=w1039:dbl[])  [unwired: 6 in]
                  n475 = Build Array(w1042, w1042, w1042, w1042, w1042, "iir_comb") -> (w1045:string[])
                  n476 = Build Array(w1053, w1052, w1051, w1050, w1049, w1048) -> (w1046:i32[])
                  n477 = call <vilib>:"NIMS_Create Error From Enums.vi"("Error Code"=bool[] [FALSE, FALSE, FALSE, FALSE, FALSE, TRUE], "error in (no error)"=w1044, "Line no"=w1047, "Error Enums"=w1046, "Function names"=w1045) -> ("error out"=w1040:errorcluster)  [unwired: 6 in]
                }
                frame "_Char:Character;_Char:Character;;" {
                  w1070 = "iir_comb"
                  n478 = call-generic <vilib>:"NIMS_Complex To Real.vi"("A"=w1082) -> ("Error Enum"=w1078:T1, "Real(A)"=w1081:dbl[][])  [unwired: 8 in, 1 out]
                  n479 = call-generic <vilib>:"NIMS_Get Scalar_w Error.vi"("A"=w1081) -> ("Error Enum"=w1077:T1, "Scalar"=w1083:dbl)  [unwired: 8 in, 1 out]
                  n480 = call <vilib>:"NIMS_CH_Character 2D to U8 2D.vi"("Character 2D array"=w1086) -> ("U8 2D array"=w1085:u8[][])  [unwired: 10 in]
                  n481 = To Double Precision Float(number=w1085) -> (double precision float=w1084:dbl[][])
                  n482 = call-generic <vilib>:"NIMS_Get Scalar_w Error.vi"("A"=w1084) -> ("Error Enum"=w1079:T1, "Scalar"=w1087:dbl)  [unwired: 8 in, 1 out]
                  n483 = call <vilib>:"NIMS_CH_Character 2D to U8 2D.vi"("Character 2D array"=w1090) -> ("U8 2D array"=w1089:u8[][])  [unwired: 10 in]
                  n484 = To Long Integer(number=w1089) -> (32bit integer=w1088:i32[][])
                  n485 = call-generic <vilib>:"NIMS_Get Scalar_w Error.vi"("A"=w1088) -> ("Error Enum"=w1080:T1, "Scalar"=w1091:i32)  [unwired: 8 in, 1 out]
                  n486 = call <vilib>:"NIMS_DF_iir_comb(n, bw, ab, t).vi"("ab"=w1083, "bw"=w1087, "n"=w1091) -> ("error"=w1076:i32, "a"=w1066:dbl[], "b"=w1067:dbl[])  [unwired: 6 in]
                  n487 = Build Array(w1070, w1070, w1070, w1070, "iir_comb") -> (w1073:string[])
                  n488 = Build Array(w1080, w1079, w1078, w1077, w1076) -> (w1074:i32[])
                  n489 = call <vilib>:"NIMS_Create Error From Enums.vi"("Error Code"=bool[] [FALSE, FALSE, FALSE, FALSE, TRUE], "error in (no error)"=w1072, "Line no"=w1075, "Error Enums"=w1074, "Function names"=w1073) -> ("error out"=w1068:errorcluster)  [unwired: 6 in]
                }
                frame "_Char:Character;_Char:Character;_Char:Character;" {
                  w1096 = "iir_comb"
                  n490 = call-generic <vilib>:"NIMS_Get Row Vector_w Error - Matrix.vi"("A"=w1109) -> ("Error Enum"=w1104:T1, "Row Vector"=w1108:T2[])  [unwired: 8 in, 1 out]
                  n491 = call <vilib>:"NIMS_CH_Character RV to String.vi"("Character array"=w1108) -> ("String"=w1110:string)  [unwired: 10 in]
                  n492 = call <vilib>:"NIMS_String to Enum.vi"("Input String"=w1110, "Enum choices"=string[] ["notch", "peak"] ("Enum Options")) -> ("Error Enum"=w1103:T1, "Enum Index"=w1111:i32)  [unwired: 8 in]
                  n493 = call <vilib>:"NIMS_CH_Character 2D to U8 2D.vi"("Character 2D array"=w1114) -> ("U8 2D array"=w1113:u8[][])  [unwired: 10 in]
                  n494 = To Double Precision Float(number=w1113) -> (double precision float=w1112:dbl[][])
                  n495 = call-generic <vilib>:"NIMS_Get Scalar_w Error.vi"("A"=w1112) -> ("Error Enum"=w1105:T1, "Scalar"=w1115:dbl)  [unwired: 8 in, 1 out]
                  n496 = call <vilib>:"NIMS_CH_Character 2D to U8 2D.vi"("Character 2D array"=w1118) -> ("U8 2D array"=w1117:u8[][])  [unwired: 10 in]
                  n497 = To Long Integer(number=w1117) -> (32bit integer=w1116:i32[][])
                  n498 = call-generic <vilib>:"NIMS_Get Scalar_w Error.vi"("A"=w1116) -> ("Error Enum"=w1106:T1, "Scalar"=w1119:i32)  [unwired: 8 in, 1 out]
                  n499 = call <vilib>:"NIMS_DF_iir_comb(n, bw, t).vi"("type"=w1111, "bw"=w1115, "n"=w1119) -> ("error"=w1102:i32, "a"=w1092:dbl[], "b"=w1093:dbl[])  [unwired: 6 in]
                  n500 = Build Array(w1096, w1096, w1096, w1096, "iir_comb") -> (w1099:string[])
                  n501 = Build Array(w1106, w1105, w1104, w1103, w1102) -> (w1100:i32[])
                  n502 = call <vilib>:"NIMS_Create Error From Enums.vi"("Error Code"=bool[] [FALSE, FALSE, FALSE, FALSE, TRUE], "error in (no error)"=w1098, "Line no"=w1101, "Error Enums"=w1100, "Function names"=w1099) -> ("error out"=w1094:errorcluster)  [unwired: 6 in]
                }
              }
              n503 = Build Array(w870) -> (w869:dbl[][])
              n504 = To Double Precision Complex(1:w869) -> (0:w868:cdb[][])
              n505 = call-generic <vilib>:"NIMS_RunTimeType_From StrictType (excl LVString).vi"("Plug-In Name"="", "Data In"=w868) -> ("Data Out"=w865:variant)  [unwired: 2 in]
              n506 = Build Array(w874) -> (w873:dbl[][])
              n507 = To Double Precision Complex(1:w873) -> (0:w872:cdb[][])
              n508 = call-generic <vilib>:"NIMS_RunTimeType_From StrictType (excl LVString).vi"("Plug-In Name"="", "Data In"=w872) -> ("Data Out"=w866:variant)  [unwired: 2 in]
              n509 = Build Array(w866, w865) -> (w864:variant[])
            }
          }
        }
        frame 4 {
          n510 = case shown="2" w1120 {
            tunnel: [_ w1132 w1426 w1720] -> w1126
            tunnel: w1123 -> [w1130 _ _ _]
            tunnel: w1124 -> [w1131 w1159 w1453 w1752]
            tunnel: w1122 -> [w1128 w1157 w1451 w1750]
            tunnel: [w1127 w1138 w1432 w1731] -> w1121
            tunnel: w1125 -> [_ w1160 w1454 w1753]
            frame Default {
              n511 = call <vilib>:"Create Error.vi"("Function name"=w1130, "error in (no error)"=w1128, "Error Enum"=error."Wrong number of output arguments", "Line number"=w1131) -> ("error out"=w1127:errorcluster)  [unwired: 6 in, 1 out]
            }
            frame 0 {
              n512 = Index Array(array=w1160) -> (element #1=w1156:variant, element #2=w1151:variant, element #3=w1146:variant, element #4=w1141:variant)  [unwired: 4 in]
              n513 = call <vilib>:"NIMS_RunTimeType_Get Case Value.vi"("Data In"=w1141) -> ("Case Value"=w1139:string)  [unwired: 9 in, 1 out]
              n514 = call <vilib>:"NIMS_CH_RunTimeType_To Character 2D.vi"("Variant"=w1141) -> ("data"=w1140:T2[][])  [unwired: 1 in]
              n515 = call <vilib>:"NIMS_RunTimeType_Get Case Value.vi"("Data In"=w1146) -> ("Case Value"=w1142:string)  [unwired: 9 in, 1 out]
              n516 = call <vilib>:"NIMS_CH_RunTimeType_To Character 2D.vi"("Variant"=w1146) -> ("data"=w1143:T2[][])  [unwired: 1 in]
              n517 = call-generic <vilib>:"NIMS_RunTimeType_To Numeric.vi"("DataType"=cdb[][] [], "Variant"=w1146) -> ("data"=w1144:cdb[][])  [unwired: 1 in]
              n518 = call <vilib>:"NIMS_RunTimeType_Get Case Value.vi"("Data In"=w1151) -> ("Case Value"=w1147:string)  [unwired: 9 in, 1 out]
              n519 = call <vilib>:"NIMS_CH_RunTimeType_To Character 2D.vi"("Variant"=w1151) -> ("data"=w1148:T2[][])  [unwired: 1 in]
              n520 = call-generic <vilib>:"NIMS_RunTimeType_To Numeric.vi"("DataType"=cdb[][] [], "Variant"=w1151) -> ("data"=w1149:cdb[][])  [unwired: 1 in]
              n521 = call <vilib>:"NIMS_RunTimeType_Get Case Value.vi"("Data In"=w1156) -> ("Case Value"=w1152:string)  [unwired: 9 in, 1 out]
              n522 = call <vilib>:"NIMS_CH_RunTimeType_To Character 2D.vi"("Variant"=w1156) -> ("data"=w1153:T2[][])  [unwired: 1 in]
              n523 = call-generic <vilib>:"NIMS_RunTimeType_To Numeric.vi"("DataType"=cdb[][] [], "Variant"=w1156) -> ("data"=w1154:cdb[][])  [unwired: 1 in]
              n524 = Concatenate Strings(w1152, w1147, w1142, w1139) -> (w1158:string)
              n525 = case shown="\"_Char:Character;_Char:Character;_Char:Character;_Char:Character;\"" w1158 {
                tunnel: w1157 -> [w1162 w1171 w1204 w1237 w1270 w1303 w1335 w1367 w1399]
                tunnel: [_ w1166 w1199 w1232 w1265 w1298 w1330 w1362 w1394] -> w1137
                tunnel: [w1161 w1167 w1200 w1233 w1266 w1299 w1331 w1363 w1395] -> w1138
                tunnel: w1154 -> [_ w1197 w1230 w1263 w1296 _ _ _ _]
                tunnel: w1153 -> [_ _ _ _ _ w1328 w1360 w1392 w1424]
                tunnel: w1149 -> [_ w1193 w1226 _ _ w1324 w1356 _ _]
                tunnel: w1148 -> [_ _ _ w1259 w1292 _ _ w1388 w1420]
                tunnel: w1144 -> [_ w1190 _ w1255 _ w1321 _ w1384 _]
                tunnel: w1143 -> [_ _ w1223 _ w1288 _ w1353 _ w1416]
                tunnel: w1140 -> [_ w1186 w1218 w1251 w1283 w1317 w1348 w1380 w1411]
                tunnel: w1159 -> [w1165 w1174 w1207 w1240 w1273 w1306 w1338 w1370 w1402]
                frame Default {
                  n526 = call <vilib>:"Create Error.vi"("Function name"="iir_comb", "error in (no error)"=w1162, "Error Enum"=23, "Line number"=w1165) -> ("error out"=w1161:errorcluster)  [unwired: 6 in, 1 out]
                }
                frame ";;;_Char:Character;" {
                  w1169 = "iir_comb"
                  n527 = call-generic <vilib>:"NIMS_Get Row Vector_w Error - Matrix.vi"("A"=w1186) -> ("Error Enum"=w1177:T1, "Row Vector"=w1185:T2[])  [unwired: 8 in, 1 out]
                  n528 = call <vilib>:"NIMS_CH_Character RV to String.vi"("Character array"=w1185) -> ("String"=w1187:string)  [unwired: 10 in]
                  n529 = call <vilib>:"NIMS_String to Enum.vi"("Input String"=w1187, "Enum choices"=string[] ["notch", "peak"] ("Enum Options")) -> ("Error Enum"=w1176:T1, "Enum Index"=w1188:i32)  [unwired: 8 in]
                  n530 = call-generic <vilib>:"NIMS_Complex To Real.vi"("A"=w1190) -> ("Error Enum"=w1179:T1, "Real(A)"=w1189:dbl[][])  [unwired: 8 in, 1 out]
                  n531 = call-generic <vilib>:"NIMS_Get Scalar_w Error.vi"("A"=w1189) -> ("Error Enum"=w1178:T1, "Scalar"=w1191:dbl)  [unwired: 8 in, 1 out]
                  n532 = call-generic <vilib>:"NIMS_Complex To Real.vi"("A"=w1193) -> ("Error Enum"=w1181:T1, "Real(A)"=w1192:dbl[][])  [unwired: 8 in, 1 out]
                  n533 = call-generic <vilib>:"NIMS_Get Scalar_w Error.vi"("A"=w1192) -> ("Error Enum"=w1180:T1, "Scalar"=w1194:dbl)  [unwired: 8 in, 1 out]
                  n534 = call-generic <vilib>:"NIMS_Complex To Real.vi"("A"=w1197) -> ("Error Enum"=w1183:T1, "Real(A)"=w1196:dbl[][])  [unwired: 8 in, 1 out]
                  n535 = To Long Integer(number=w1196) -> (32bit integer=w1195:i32[][])
                  n536 = call-generic <vilib>:"NIMS_Get Scalar_w Error.vi"("A"=w1195) -> ("Error Enum"=w1182:T1, "Scalar"=w1198:i32)  [unwired: 8 in, 1 out]
                  n537 = call <vilib>:"NIMS_DF_iir_comb(n, bw, ab, t).vi"("type"=w1188, "ab"=w1191, "bw"=w1194, "n"=w1198) -> ("error"=w1175:i32, "b"=w1166:dbl[])  [unwired: 5 in, 1 out]
                  n538 = Build Array(w1169, w1169, w1169, w1169, w1169, w1169, w1169, w1169, "iir_comb") -> (w1172:string[])
                  n539 = Build Array(w1183, w1182, w1181, w1180, w1179, w1178, w1177, w1176, w1175) -> (w1173:i32[])
                  n540 = call <vilib>:"NIMS_Create Error From Enums.vi"("Error Code"=bool[] [FALSE, FALSE, FALSE, FALSE, FALSE, FALSE, FALSE, FALSE, TRUE], "error in (no error)"=w1171, "Line no"=w1174, "Error Enums"=w1173, "Function names"=w1172) -> ("error out"=w1167:errorcluster)  [unwired: 6 in]
                }
                frame ";;_Char:Character;_Char:Character;" {
                  w1202 = "iir_comb"
                  n541 = call-generic <vilib>:"NIMS_Get Row Vector_w Error - Matrix.vi"("A"=w1218) -> ("Error Enum"=w1210:T1, "Row Vector"=w1217:T2[])  [unwired: 8 in, 1 out]
                  n542 = call <vilib>:"NIMS_CH_Character RV to String.vi"("Character array"=w1217) -> ("String"=w1219:string)  [unwired: 10 in]
                  n543 = call <vilib>:"NIMS_String to Enum.vi"("Input String"=w1219, "Enum choices"=string[] ["notch", "peak"] ("Enum Options")) -> ("Error Enum"=w1209:T1, "Enum Index"=w1220:i32)  [unwired: 8 in]
                  n544 = call <vilib>:"NIMS_CH_Character 2D to U8 2D.vi"("Character 2D array"=w1223) -> ("U8 2D array"=w1222:u8[][])  [unwired: 10 in]
                  n545 = To Double Precision Float(number=w1222) -> (double precision float=w1221:dbl[][])
                  n546 = call-generic <vilib>:"NIMS_Get Scalar_w Error.vi"("A"=w1221) -> ("Error Enum"=w1211:T1, "Scalar"=w1224:dbl)  [unwired: 8 in, 1 out]
                  n547 = call-generic <vilib>:"NIMS_Complex To Real.vi"("A"=w1226) -> ("Error Enum"=w1213:T1, "Real(A)"=w1225:dbl[][])  [unwired: 8 in, 1 out]
                  n548 = call-generic <vilib>:"NIMS_Get Scalar_w Error.vi"("A"=w1225) -> ("Error Enum"=w1212:T1, "Scalar"=w1227:dbl)  [unwired: 8 in, 1 out]
                  n549 = call-generic <vilib>:"NIMS_Complex To Real.vi"("A"=w1230) -> ("Error Enum"=w1215:T1, "Real(A)"=w1229:dbl[][])  [unwired: 8 in, 1 out]
                  n550 = To Long Integer(number=w1229) -> (32bit integer=w1228:i32[][])
                  n551 = call-generic <vilib>:"NIMS_Get Scalar_w Error.vi"("A"=w1228) -> ("Error Enum"=w1214:T1, "Scalar"=w1231:i32)  [unwired: 8 in, 1 out]
                  n552 = call <vilib>:"NIMS_DF_iir_comb(n, bw, ab, t).vi"("type"=w1220, "ab"=w1224, "bw"=w1227, "n"=w1231) -> ("error"=w1208:i32, "b"=w1199:dbl[])  [unwired: 5 in, 1 out]
                  n553 = Build Array(w1202, w1202, w1202, w1202, w1202, w1202, w1202, "iir_comb") -> (w1205:string[])
                  n554 = Build Array(w1215, w1214, w1213, w1212, w1211, w1210, w1209, w1208) -> (w1206:i32[])
                  n555 = call <vilib>:"NIMS_Create Error From Enums.vi"("Error Code"=bool[] [FALSE, FALSE, FALSE, FALSE, FALSE, FALSE, FALSE, TRUE], "error in (no error)"=w1204, "Line no"=w1207, "Error Enums"=w1206, "Function names"=w1205) -> ("error out"=w1200:errorcluster)  [unwired: 6 in]
                }
                frame ";_Char:Character;;_Char:Character;" {
                  w1235 = "iir_comb"
                  n556 = call-generic <vilib>:"NIMS_Get Row Vector_w Error - Matrix.vi"("A"=w1251) -> ("Error Enum"=w1243:T1, "Row Vector"=w1250:T2[])  [unwired: 8 in, 1 out]
                  n557 = call <vilib>:"NIMS_CH_Character RV to String.vi"("Character array"=w1250) -> ("String"=w1252:string)  [unwired: 10 in]
                  n558 = call <vilib>:"NIMS_String to Enum.vi"("Input String"=w1252, "Enum choices"=string[] ["notch", "peak"] ("Enum Options")) -> ("Error Enum"=w1242:T1, "Enum Index"=w1253:i32)  [unwired: 8 in]
                  n559 = call-generic <vilib>:"NIMS_Complex To Real.vi"("A"=w1255) -> ("Error Enum"=w1245:T1, "Real(A)"=w1254:dbl[][])  [unwired: 8 in, 1 out]
                  n560 = call-generic <vilib>:"NIMS_Get Scalar_w Error.vi"("A"=w1254) -> ("Error Enum"=w1244:T1, "Scalar"=w1256:dbl)  [unwired: 8 in, 1 out]
                  n561 = call <vilib>:"NIMS_CH_Character 2D to U8 2D.vi"("Character 2D array"=w1259) -> ("U8 2D array"=w1258:u8[][])  [unwired: 10 in]
                  n562 = To Double Precision Float(number=w1258) -> (double precision float=w1257:dbl[][])
                  n563 = call-generic <vilib>:"NIMS_Get Scalar_w Error.vi"("A"=w1257) -> ("Error Enum"=w1246:T1, "Scalar"=w1260:dbl)  [unwired: 8 in, 1 out]
                  n564 = call-generic <vilib>:"NIMS_Complex To Real.vi"("A"=w1263) -> ("Error Enum"=w1248:T1, "Real(A)"=w1262:dbl[][])  [unwired: 8 in, 1 out]
                  n565 = To Long Integer(number=w1262) -> (32bit integer=w1261:i32[][])
                  n566 = call-generic <vilib>:"NIMS_Get Scalar_w Error.vi"("A"=w1261) -> ("Error Enum"=w1247:T1, "Scalar"=w1264:i32)  [unwired: 8 in, 1 out]
                  n567 = call <vilib>:"NIMS_DF_iir_comb(n, bw, ab, t).vi"("type"=w1253, "ab"=w1256, "bw"=w1260, "n"=w1264) -> ("error"=w1241:i32, "b"=w1232:dbl[])  [unwired: 5 in, 1 out]
                  n568 = Build Array(w1235, w1235, w1235, w1235, w1235, w1235, w1235, "iir_comb") -> (w1238:string[])
                  n569 = Build Array(w1248, w1247, w1246, w1245, w1244, w1243, w1242, w1241) -> (w1239:i32[])
                  n570 = call <vilib>:"NIMS_Create Error From Enums.vi"("Error Code"=bool[] [FALSE, FALSE, FALSE, FALSE, FALSE, FALSE, FALSE, TRUE], "error in (no error)"=w1237, "Line no"=w1240, "Error Enums"=w1239, "Function names"=w1238) -> ("error out"=w1233:errorcluster)  [unwired: 6 in]
                }
                frame ";_Char:Character;_Char:Character;_Char:Character;" {
                  w1268 = "iir_comb"
                  n571 = call-generic <vilib>:"NIMS_Get Row Vector_w Error - Matrix.vi"("A"=w1283) -> ("Error Enum"=w1276:T1, "Row Vector"=w1282:T2[])  [unwired: 8 in, 1 out]
                  n572 = call <vilib>:"NIMS_CH_Character RV to String.vi"("Character array"=w1282) -> ("String"=w1284:string)  [unwired: 10 in]
                  n573 = call <vilib>:"NIMS_String to Enum.vi"("Input String"=w1284, "Enum choices"=string[] ["notch", "peak"] ("Enum Options")) -> ("Error Enum"=w1275:T1, "Enum Index"=w1285:i32)  [unwired: 8 in]
                  n574 = call <vilib>:"NIMS_CH_Character 2D to U8 2D.vi"("Character 2D array"=w1288) -> ("U8 2D array"=w1287:u8[][])  [unwired: 10 in]
                  n575 = To Double Precision Float(number=w1287) -> (double precision float=w1286:dbl[][])
                  n576 = call-generic <vilib>:"NIMS_Get Scalar_w Error.vi"("A"=w1286) -> ("Error Enum"=w1277:T1, "Scalar"=w1289:dbl)  [unwired: 8 in, 1 out]
                  n577 = call <vilib>:"NIMS_CH_Character 2D to U8 2D.vi"("Character 2D array"=w1292) -> ("U8 2D array"=w1291:u8[][])  [unwired: 10 in]
                  n578 = To Double Precision Float(number=w1291) -> (double precision float=w1290:dbl[][])
                  n579 = call-generic <vilib>:"NIMS_Get Scalar_w Error.vi"("A"=w1290) -> ("Error Enum"=w1278:T1, "Scalar"=w1293:dbl)  [unwired: 8 in, 1 out]
                  n580 = call-generic <vilib>:"NIMS_Complex To Real.vi"("A"=w1296) -> ("Error Enum"=w1280:T1, "Real(A)"=w1295:dbl[][])  [unwired: 8 in, 1 out]
                  n581 = To Long Integer(number=w1295) -> (32bit integer=w1294:i32[][])
                  n582 = call-generic <vilib>:"NIMS_Get Scalar_w Error.vi"("A"=w1294) -> ("Error Enum"=w1279:T1, "Scalar"=w1297:i32)  [unwired: 8 in, 1 out]
                  n583 = call <vilib>:"NIMS_DF_iir_comb(n, bw, ab, t).vi"("type"=w1285, "ab"=w1289, "bw"=w1293, "n"=w1297) -> ("error"=w1274:i32, "b"=w1265:dbl[])  [unwired: 5 in, 1 out]
                  n584 = Build Array(w1268, w1268, w1268, w1268, w1268, w1268, "iir_comb") -> (w1271:string[])
                  n585 = Build Array(w1280, w1279, w1278, w1277, w1276, w1275, w1274) -> (w1272:i32[])
                  n586 = call <vilib>:"NIMS_Create Error From Enums.vi"("Error Code"=bool[] [FALSE, FALSE, FALSE, FALSE, FALSE, FALSE, TRUE], "error in (no error)"=w1270, "Line no"=w1273, "Error Enums"=w1272, "Function names"=w1271) -> ("error out"=w1266:errorcluster)  [unwired: 6 in]
                }
                frame "_Char:Character;;;_Char:Character;" {
                  w1301 = "iir_comb"
                  n587 = call-generic <vilib>:"NIMS_Get Row Vector_w Error - Matrix.vi"("A"=w1317) -> ("Error Enum"=w1309:T1, "Row Vector"=w1316:T2[])  [unwired: 8 in, 1 out]
                  n588 = call <vilib>:"NIMS_CH_Character RV to String.vi"("Character array"=w1316) -> ("String"=w1318:string)  [unwired: 10 in]
                  n589 = call <vilib>:"NIMS_String to Enum.vi"("Input String"=w1318, "Enum choices"=string[] ["notch", "peak"] ("Enum Options")) -> ("Error Enum"=w1308:T1, "Enum Index"=w1319:i32)  [unwired: 8 in]
                  n590 = call-generic <vilib>:"NIMS_Complex To Real.vi"("A"=w1321) -> ("Error Enum"=w1311:T1, "Real(A)"=w1320:dbl[][])  [unwired: 8 in, 1 out]
                  n591 = call-generic <vilib>:"NIMS_Get Scalar_w Error.vi"("A"=w1320) -> ("Error Enum"=w1310:T1, "Scalar"=w1322:dbl)  [unwired: 8 in, 1 out]
                  n592 = call-generic <vilib>:"NIMS_Complex To Real.vi"("A"=w1324) -> ("Error Enum"=w1313:T1, "Real(A)"=w1323:dbl[][])  [unwired: 8 in, 1 out]
                  n593 = call-generic <vilib>:"NIMS_Get Scalar_w Error.vi"("A"=w1323) -> ("Error Enum"=w1312:T1, "Scalar"=w1325:dbl)  [unwired: 8 in, 1 out]
                  n594 = call <vilib>:"NIMS_CH_Character 2D to U8 2D.vi"("Character 2D array"=w1328) -> ("U8 2D array"=w1327:u8[][])  [unwired: 10 in]
                  n595 = To Long Integer(number=w1327) -> (32bit integer=w1326:i32[][])
                  n596 = call-generic <vilib>:"NIMS_Get Scalar_w Error.vi"("A"=w1326) -> ("Error Enum"=w1314:T1, "Scalar"=w1329:i32)  [unwired: 8 in, 1 out]
                  n597 = call <vilib>:"NIMS_DF_iir_comb(n, bw, ab, t).vi"("type"=w1319, "ab"=w1322, "bw"=w1325, "n"=w1329) -> ("error"=w1307:i32, "b"=w1298:dbl[])  [unwired: 5 in, 1 out]
                  n598 = Build Array(w1301, w1301, w1301, w1301, w1301, w1301, w1301, "iir_comb") -> (w1304:string[])
                  n599 = Build Array(w1314, w1313, w1312, w1311, w1310, w1309, w1308, w1307) -> (w1305:i32[])
                  n600 = call <vilib>:"NIMS_Create Error From Enums.vi"("Error Code"=bool[] [FALSE, FALSE, FALSE, FALSE, FALSE, FALSE, FALSE, TRUE], "error in (no error)"=w1303, "Line no"=w1306, "Error Enums"=w1305, "Function names"=w1304) -> ("error out"=w1299:errorcluster)  [unwired: 6 in]
                }
                frame "_Char:Character;;_Char:Character;_Char:Character;" {
                  w1333 = "iir_comb"
                  n601 = call-generic <vilib>:"NIMS_Get Row Vector_w Error - Matrix.vi"("A"=w1348) -> ("Error Enum"=w1341:T1, "Row Vector"=w1347:T2[])  [unwired: 8 in, 1 out]
                  n602 = call <vilib>:"NIMS_CH_Character RV to String.vi"("Character array"=w1347) -> ("String"=w1349:string)  [unwired: 10 in]
                  n603 = call <vilib>:"NIMS_String to Enum.vi"("Input String"=w1349, "Enum choices"=string[] ["notch", "peak"] ("Enum Options")) -> ("Error Enum"=w1340:T1, "Enum Index"=w1350:i32)  [unwired: 8 in]
                  n604 = call <vilib>:"NIMS_CH_Character 2D to U8 2D.vi"("Character 2D array"=w1353) -> ("U8 2D array"=w1352:u8[][])  [unwired: 10 in]
                  n605 = To Double Precision Float(number=w1352) -> (double precision float=w1351:dbl[][])
                  n606 = call-generic <vilib>:"NIMS_Get Scalar_w Error.vi"("A"=w1351) -> ("Error Enum"=w1342:T1, "Scalar"=w1354:dbl)  [unwired: 8 in, 1 out]
                  n607 = call-generic <vilib>:"NIMS_Complex To Real.vi"("A"=w1356) -> ("Error Enum"=w1344:T1, "Real(A)"=w1355:dbl[][])  [unwired: 8 in, 1 out]
                  n608 = call-generic <vilib>:"NIMS_Get Scalar_w Error.vi"("A"=w1355) -> ("Error Enum"=w1343:T1, "Scalar"=w1357:dbl)  [unwired: 8 in, 1 out]
                  n609 = call <vilib>:"NIMS_CH_Character 2D to U8 2D.vi"("Character 2D array"=w1360) -> ("U8 2D array"=w1359:u8[][])  [unwired: 10 in]
                  n610 = To Long Integer(number=w1359) -> (32bit integer=w1358:i32[][])
                  n611 = call-generic <vilib>:"NIMS_Get Scalar_w Error.vi"("A"=w1358) -> ("Error Enum"=w1345:T1, "Scalar"=w1361:i32)  [unwired: 8 in, 1 out]
                  n612 = call <vilib>:"NIMS_DF_iir_comb(n, bw, ab, t).vi"("type"=w1350, "ab"=w1354, "bw"=w1357, "n"=w1361) -> ("error"=w1339:i32, "b"=w1330:dbl[])  [unwired: 5 in, 1 out]
                  n613 = Build Array(w1333, w1333, w1333, w1333, w1333, w1333, "iir_comb") -> (w1336:string[])
                  n614 = Build Array(w1345, w1344, w1343, w1342, w1341, w1340, w1339) -> (w1337:i32[])
                  n615 = call <vilib>:"NIMS_Create Error From Enums.vi"("Error Code"=bool[] [FALSE, FALSE, FALSE, FALSE, FALSE, FALSE, TRUE], "error in (no error)"=w1335, "Line no"=w1338, "Error Enums"=w1337, "Function names"=w1336) -> ("error out"=w1331:errorcluster)  [unwired: 6 in]
                }
                frame "_Char:Character;_Char:Character;;_Char:Character;" {
                  w1365 = "iir_comb"
                  n616 = call-generic <vilib>:"NIMS_Get Row Vector_w Error - Matrix.vi"("A"=w1380) -> ("Error Enum"=w1373:T1, "Row Vector"=w1379:T2[])  [unwired: 8 in, 1 out]
                  n617 = call <vilib>:"NIMS_CH_Character RV to String.vi"("Character array"=w1379) -> ("String"=w1381:string)  [unwired: 10 in]
                  n618 = call <vilib>:"NIMS_String to Enum.vi"("Input String"=w1381, "Enum choices"=string[] ["notch", "peak"] ("Enum Options")) -> ("Error Enum"=w1372:T1, "Enum Index"=w1382:i32)  [unwired: 8 in]
                  n619 = call-generic <vilib>:"NIMS_Complex To Real.vi"("A"=w1384) -> ("Error Enum"=w1375:T1, "Real(A)"=w1383:dbl[][])  [unwired: 8 in, 1 out]
                  n620 = call-generic <vilib>:"NIMS_Get Scalar_w Error.vi"("A"=w1383) -> ("Error Enum"=w1374:T1, "Scalar"=w1385:dbl)  [unwired: 8 in, 1 out]
                  n621 = call <vilib>:"NIMS_CH_Character 2D to U8 2D.vi"("Character 2D array"=w1388) -> ("U8 2D array"=w1387:u8[][])  [unwired: 10 in]
                  n622 = To Double Precision Float(number=w1387) -> (double precision float=w1386:dbl[][])
                  n623 = call-generic <vilib>:"NIMS_Get Scalar_w Error.vi"("A"=w1386) -> ("Error Enum"=w1376:T1, "Scalar"=w1389:dbl)  [unwired: 8 in, 1 out]
                  n624 = call <vilib>:"NIMS_CH_Character 2D to U8 2D.vi"("Character 2D array"=w1392) -> ("U8 2D array"=w1391:u8[][])  [unwired: 10 in]
                  n625 = To Long Integer(number=w1391) -> (32bit integer=w1390:i32[][])
                  n626 = call-generic <vilib>:"NIMS_Get Scalar_w Error.vi"("A"=w1390) -> ("Error Enum"=w1377:T1, "Scalar"=w1393:i32)  [unwired: 8 in, 1 out]
                  n627 = call <vilib>:"NIMS_DF_iir_comb(n, bw, ab, t).vi"("type"=w1382, "ab"=w1385, "bw"=w1389, "n"=w1393) -> ("error"=w1371:i32, "b"=w1362:dbl[])  [unwired: 5 in, 1 out]
                  n628 = Build Array(w1365, w1365, w1365, w1365, w1365, w1365, "iir_comb") -> (w1368:string[])
                  n629 = Build Array(w1377, w1376, w1375, w1374, w1373, w1372, w1371) -> (w1369:i32[])
                  n630 = call <vilib>:"NIMS_Create Error From Enums.vi"("Error Code"=bool[] [FALSE, FALSE, FALSE, FALSE, FALSE, FALSE, TRUE], "error in (no error)"=w1367, "Line no"=w1370, "Error Enums"=w1369, "Function names"=w1368) -> ("error out"=w1363:errorcluster)  [unwired: 6 in]
                }
                frame "_Char:Character;_Char:Character;_Char:Character;_Char:Character;" {
                  w1397 = "iir_comb"
                  n631 = call-generic <vilib>:"NIMS_Get Row Vector_w Error - Matrix.vi"("A"=w1411) -> ("Error Enum"=w1405:T1, "Row Vector"=w1410:T2[])  [unwired: 8 in, 1 out]
                  n632 = call <vilib>:"NIMS_CH_Character RV to String.vi"("Character array"=w1410) -> ("String"=w1412:string)  [unwired: 10 in]
                  n633 = call <vilib>:"NIMS_String to Enum.vi"("Input String"=w1412, "Enum choices"=string[] ["notch", "peak"] ("Enum Options")) -> ("Error Enum"=w1404:T1, "Enum Index"=w1413:i32)  [unwired: 8 in]
                  n634 = call <vilib>:"NIMS_CH_Character 2D to U8 2D.vi"("Character 2D array"=w1416) -> ("U8 2D array"=w1415:u8[][])  [unwired: 10 in]
                  n635 = To Double Precision Float(number=w1415) -> (double precision float=w1414:dbl[][])
                  n636 = call-generic <vilib>:"NIMS_Get Scalar_w Error.vi"("A"=w1414) -> ("Error Enum"=w1406:T1, "Scalar"=w1417:dbl)  [unwired: 8 in, 1 out]
                  n637 = call <vilib>:"NIMS_CH_Character 2D to U8 2D.vi"("Character 2D array"=w1420) -> ("U8 2D array"=w1419:u8[][])  [unwired: 10 in]
                  n638 = To Double Precision Float(number=w1419) -> (double precision float=w1418:dbl[][])
                  n639 = call-generic <vilib>:"NIMS_Get Scalar_w Error.vi"("A"=w1418) -> ("Error Enum"=w1407:T1, "Scalar"=w1421:dbl)  [unwired: 8 in, 1 out]
                  n640 = call <vilib>:"NIMS_CH_Character 2D to U8 2D.vi"("Character 2D array"=w1424) -> ("U8 2D array"=w1423:u8[][])  [unwired: 10 in]
                  n641 = To Long Integer(number=w1423) -> (32bit integer=w1422:i32[][])
                  n642 = call-generic <vilib>:"NIMS_Get Scalar_w Error.vi"("A"=w1422) -> ("Error Enum"=w1408:T1, "Scalar"=w1425:i32)  [unwired: 8 in, 1 out]
                  n643 = call <vilib>:"NIMS_DF_iir_comb(n, bw, ab, t).vi"("type"=w1413, "ab"=w1417, "bw"=w1421, "n"=w1425) -> ("error"=w1403:i32, "b"=w1394:dbl[])  [unwired: 5 in, 1 out]
                  n644 = Build Array(w1397, w1397, w1397, w1397, w1397, "iir_comb") -> (w1400:string[])
                  n645 = Build Array(w1408, w1407, w1406, w1405, w1404, w1403) -> (w1401:i32[])
                  n646 = call <vilib>:"NIMS_Create Error From Enums.vi"("Error Code"=bool[] [FALSE, FALSE, FALSE, FALSE, FALSE, TRUE], "error in (no error)"=w1399, "Line no"=w1402, "Error Enums"=w1401, "Function names"=w1400) -> ("error out"=w1395:errorcluster)  [unwired: 6 in]
                }
              }
              n647 = Build Array(w1137) -> (w1136:dbl[][])
              n648 = To Double Precision Complex(1:w1136) -> (0:w1135:cdb[][])
              n649 = call-generic <vilib>:"NIMS_RunTimeType_From StrictType (excl LVString).vi"("Plug-In Name"="", "Data In"=w1135) -> ("Data Out"=w1133:variant)  [unwired: 2 in]
              n650 = Build Array(w1133) -> (w1132:variant[])
            }
            frame 1 {
              n651 = Index Array(array=w1454) -> (element #1=w1450:variant, element #2=w1445:variant, element #3=w1440:variant, element #4=w1435:variant)  [unwired: 4 in]
              n652 = call <vilib>:"NIMS_RunTimeType_Get Case Value.vi"("Data In"=w1435) -> ("Case Value"=w1433:string)  [unwired: 9 in, 1 out]
              n653 = call <vilib>:"NIMS_CH_RunTimeType_To Character 2D.vi"("Variant"=w1435) -> ("data"=w1434:T2[][])  [unwired: 1 in]
              n654 = call <vilib>:"NIMS_RunTimeType_Get Case Value.vi"("Data In"=w1440) -> ("Case Value"=w1436:string)  [unwired: 9 in, 1 out]
              n655 = call <vilib>:"NIMS_CH_RunTimeType_To Character 2D.vi"("Variant"=w1440) -> ("data"=w1437:T2[][])  [unwired: 1 in]
              n656 = call-generic <vilib>:"NIMS_RunTimeType_To Numeric.vi"("DataType"=cdb[][] [], "Variant"=w1440) -> ("data"=w1438:cdb[][])  [unwired: 1 in]
              n657 = call <vilib>:"NIMS_RunTimeType_Get Case Value.vi"("Data In"=w1445) -> ("Case Value"=w1441:string)  [unwired: 9 in, 1 out]
              n658 = call <vilib>:"NIMS_CH_RunTimeType_To Character 2D.vi"("Variant"=w1445) -> ("data"=w1442:T2[][])  [unwired: 1 in]
              n659 = call-generic <vilib>:"NIMS_RunTimeType_To Numeric.vi"("DataType"=cdb[][] [], "Variant"=w1445) -> ("data"=w1443:cdb[][])  [unwired: 1 in]
              n660 = call <vilib>:"NIMS_RunTimeType_Get Case Value.vi"("Data In"=w1450) -> ("Case Value"=w1446:string)  [unwired: 9 in, 1 out]
              n661 = call <vilib>:"NIMS_CH_RunTimeType_To Character 2D.vi"("Variant"=w1450) -> ("data"=w1447:T2[][])  [unwired: 1 in]
              n662 = call-generic <vilib>:"NIMS_RunTimeType_To Numeric.vi"("DataType"=cdb[][] [], "Variant"=w1450) -> ("data"=w1448:cdb[][])  [unwired: 1 in]
              n663 = Concatenate Strings(w1446, w1441, w1436, w1433) -> (w1452:string)
              n664 = case shown="\"_Char:Character;_Char:Character;_Char:Character;_Char:Character;\"" w1452 {
                tunnel: w1451 -> [w1456 w1465 w1498 w1531 w1564 w1597 w1629 w1661 w1693]
                tunnel: [_ w1460 w1493 w1526 w1559 w1592 w1624 w1656 w1688] -> w1431
                tunnel: [w1455 w1461 w1494 w1527 w1560 w1593 w1625 w1657 w1689] -> w1432
                tunnel: w1448 -> [_ w1491 w1524 w1557 w1590 _ _ _ _]
                tunnel: w1447 -> [_ _ _ _ _ w1622 w1654 w1686 w1718]
                tunnel: w1443 -> [_ w1487 w1520 _ _ w1618 w1650 _ _]
                tunnel: w1442 -> [_ _ _ w1553 w1586 _ _ w1682 w1714]
                tunnel: w1438 -> [_ w1484 _ w1549 _ w1615 _ w1678 _]
                tunnel: w1437 -> [_ _ w1517 _ w1582 _ w1647 _ w1710]
                tunnel: w1434 -> [_ w1480 w1512 w1545 w1577 w1611 w1642 w1674 w1705]
                tunnel: w1453 -> [w1459 w1468 w1501 w1534 w1567 w1600 w1632 w1664 w1696]
                frame Default {
                  n665 = call <vilib>:"Create Error.vi"("Function name"="iir_comb", "error in (no error)"=w1456, "Error Enum"=23, "Line number"=w1459) -> ("error out"=w1455:errorcluster)  [unwired: 6 in, 1 out]
                }
                frame ";;;_Char:Character;" {
                  w1463 = "iir_comb"
                  n666 = call-generic <vilib>:"NIMS_Get Row Vector_w Error - Matrix.vi"("A"=w1480) -> ("Error Enum"=w1471:T1, "Row Vector"=w1479:T2[])  [unwired: 8 in, 1 out]
                  n667 = call <vilib>:"NIMS_CH_Character RV to String.vi"("Character array"=w1479) -> ("String"=w1481:string)  [unwired: 10 in]
                  n668 = call <vilib>:"NIMS_String to Enum.vi"("Input String"=w1481, "Enum choices"=string[] ["notch", "peak"] ("Enum Options")) -> ("Error Enum"=w1470:T1, "Enum Index"=w1482:i32)  [unwired: 8 in]
                  n669 = call-generic <vilib>:"NIMS_Complex To Real.vi"("A"=w1484) -> ("Error Enum"=w1473:T1, "Real(A)"=w1483:dbl[][])  [unwired: 8 in, 1 out]
                  n670 = call-generic <vilib>:"NIMS_Get Scalar_w Error.vi"("A"=w1483) -> ("Error Enum"=w1472:T1, "Scalar"=w1485:dbl)  [unwired: 8 in, 1 out]
                  n671 = call-generic <vilib>:"NIMS_Complex To Real.vi"("A"=w1487) -> ("Error Enum"=w1475:T1, "Real(A)"=w1486:dbl[][])  [unwired: 8 in, 1 out]
                  n672 = call-generic <vilib>:"NIMS_Get Scalar_w Error.vi"("A"=w1486) -> ("Error Enum"=w1474:T1, "Scalar"=w1488:dbl)  [unwired: 8 in, 1 out]
                  n673 = call-generic <vilib>:"NIMS_Complex To Real.vi"("A"=w1491) -> ("Error Enum"=w1477:T1, "Real(A)"=w1490:dbl[][])  [unwired: 8 in, 1 out]
                  n674 = To Long Integer(number=w1490) -> (32bit integer=w1489:i32[][])
                  n675 = call-generic <vilib>:"NIMS_Get Scalar_w Error.vi"("A"=w1489) -> ("Error Enum"=w1476:T1, "Scalar"=w1492:i32)  [unwired: 8 in, 1 out]
                  n676 = call <vilib>:"NIMS_DF_iir_comb(n, bw, ab, t).vi"("type"=w1482, "ab"=w1485, "bw"=w1488, "n"=w1492) -> ("error"=w1469:i32, "b"=w1460:dbl[])  [unwired: 5 in, 1 out]
                  n677 = Build Array(w1463, w1463, w1463, w1463, w1463, w1463, w1463, w1463, "iir_comb") -> (w1466:string[])
                  n678 = Build Array(w1477, w1476, w1475, w1474, w1473, w1472, w1471, w1470, w1469) -> (w1467:i32[])
                  n679 = call <vilib>:"NIMS_Create Error From Enums.vi"("Error Code"=bool[] [FALSE, FALSE, FALSE, FALSE, FALSE, FALSE, FALSE, FALSE, TRUE], "error in (no error)"=w1465, "Line no"=w1468, "Error Enums"=w1467, "Function names"=w1466) -> ("error out"=w1461:errorcluster)  [unwired: 6 in]
                }
                frame ";;_Char:Character;_Char:Character;" {
                  w1496 = "iir_comb"
                  n680 = call-generic <vilib>:"NIMS_Get Row Vector_w Error - Matrix.vi"("A"=w1512) -> ("Error Enum"=w1504:T1, "Row Vector"=w1511:T2[])  [unwired: 8 in, 1 out]
                  n681 = call <vilib>:"NIMS_CH_Character RV to String.vi"("Character array"=w1511) -> ("String"=w1513:string)  [unwired: 10 in]
                  n682 = call <vilib>:"NIMS_String to Enum.vi"("Input String"=w1513, "Enum choices"=string[] ["notch", "peak"] ("Enum Options")) -> ("Error Enum"=w1503:T1, "Enum Index"=w1514:i32)  [unwired: 8 in]
                  n683 = call <vilib>:"NIMS_CH_Character 2D to U8 2D.vi"("Character 2D array"=w1517) -> ("U8 2D array"=w1516:u8[][])  [unwired: 10 in]
                  n684 = To Double Precision Float(number=w1516) -> (double precision float=w1515:dbl[][])
                  n685 = call-generic <vilib>:"NIMS_Get Scalar_w Error.vi"("A"=w1515) -> ("Error Enum"=w1505:T1, "Scalar"=w1518:dbl)  [unwired: 8 in, 1 out]
                  n686 = call-generic <vilib>:"NIMS_Complex To Real.vi"("A"=w1520) -> ("Error Enum"=w1507:T1, "Real(A)"=w1519:dbl[][])  [unwired: 8 in, 1 out]
                  n687 = call-generic <vilib>:"NIMS_Get Scalar_w Error.vi"("A"=w1519) -> ("Error Enum"=w1506:T1, "Scalar"=w1521:dbl)  [unwired: 8 in, 1 out]
                  n688 = call-generic <vilib>:"NIMS_Complex To Real.vi"("A"=w1524) -> ("Error Enum"=w1509:T1, "Real(A)"=w1523:dbl[][])  [unwired: 8 in, 1 out]
                  n689 = To Long Integer(number=w1523) -> (32bit integer=w1522:i32[][])
                  n690 = call-generic <vilib>:"NIMS_Get Scalar_w Error.vi"("A"=w1522) -> ("Error Enum"=w1508:T1, "Scalar"=w1525:i32)  [unwired: 8 in, 1 out]
                  n691 = call <vilib>:"NIMS_DF_iir_comb(n, bw, ab, t).vi"("type"=w1514, "ab"=w1518, "bw"=w1521, "n"=w1525) -> ("error"=w1502:i32, "b"=w1493:dbl[])  [unwired: 5 in, 1 out]
                  n692 = Build Array(w1496, w1496, w1496, w1496, w1496, w1496, w1496, "iir_comb") -> (w1499:string[])
                  n693 = Build Array(w1509, w1508, w1507, w1506, w1505, w1504, w1503, w1502) -> (w1500:i32[])
                  n694 = call <vilib>:"NIMS_Create Error From Enums.vi"("Error Code"=bool[] [FALSE, FALSE, FALSE, FALSE, FALSE, FALSE, FALSE, TRUE], "error in (no error)"=w1498, "Line no"=w1501, "Error Enums"=w1500, "Function names"=w1499) -> ("error out"=w1494:errorcluster)  [unwired: 6 in]
                }
                frame ";_Char:Character;;_Char:Character;" {
                  w1529 = "iir_comb"
                  n695 = call-generic <vilib>:"NIMS_Get Row Vector_w Error - Matrix.vi"("A"=w1545) -> ("Error Enum"=w1537:T1, "Row Vector"=w1544:T2[])  [unwired: 8 in, 1 out]
                  n696 = call <vilib>:"NIMS_CH_Character RV to String.vi"("Character array"=w1544) -> ("String"=w1546:string)  [unwired: 10 in]
                  n697 = call <vilib>:"NIMS_String to Enum.vi"("Input String"=w1546, "Enum choices"=string[] ["notch", "peak"] ("Enum Options")) -> ("Error Enum"=w1536:T1, "Enum Index"=w1547:i32)  [unwired: 8 in]
                  n698 = call-generic <vilib>:"NIMS_Complex To Real.vi"("A"=w1549) -> ("Error Enum"=w1539:T1, "Real(A)"=w1548:dbl[][])  [unwired: 8 in, 1 out]
                  n699 = call-generic <vilib>:"NIMS_Get Scalar_w Error.vi"("A"=w1548) -> ("Error Enum"=w1538:T1, "Scalar"=w1550:dbl)  [unwired: 8 in, 1 out]
                  n700 = call <vilib>:"NIMS_CH_Character 2D to U8 2D.vi"("Character 2D array"=w1553) -> ("U8 2D array"=w1552:u8[][])  [unwired: 10 in]
                  n701 = To Double Precision Float(number=w1552) -> (double precision float=w1551:dbl[][])
                  n702 = call-generic <vilib>:"NIMS_Get Scalar_w Error.vi"("A"=w1551) -> ("Error Enum"=w1540:T1, "Scalar"=w1554:dbl)  [unwired: 8 in, 1 out]
                  n703 = call-generic <vilib>:"NIMS_Complex To Real.vi"("A"=w1557) -> ("Error Enum"=w1542:T1, "Real(A)"=w1556:dbl[][])  [unwired: 8 in, 1 out]
                  n704 = To Long Integer(number=w1556) -> (32bit integer=w1555:i32[][])
                  n705 = call-generic <vilib>:"NIMS_Get Scalar_w Error.vi"("A"=w1555) -> ("Error Enum"=w1541:T1, "Scalar"=w1558:i32)  [unwired: 8 in, 1 out]
                  n706 = call <vilib>:"NIMS_DF_iir_comb(n, bw, ab, t).vi"("type"=w1547, "ab"=w1550, "bw"=w1554, "n"=w1558) -> ("error"=w1535:i32, "b"=w1526:dbl[])  [unwired: 5 in, 1 out]
                  n707 = Build Array(w1529, w1529, w1529, w1529, w1529, w1529, w1529, "iir_comb") -> (w1532:string[])
                  n708 = Build Array(w1542, w1541, w1540, w1539, w1538, w1537, w1536, w1535) -> (w1533:i32[])
                  n709 = call <vilib>:"NIMS_Create Error From Enums.vi"("Error Code"=bool[] [FALSE, FALSE, FALSE, FALSE, FALSE, FALSE, FALSE, TRUE], "error in (no error)"=w1531, "Line no"=w1534, "Error Enums"=w1533, "Function names"=w1532) -> ("error out"=w1527:errorcluster)  [unwired: 6 in]
                }
                frame ";_Char:Character;_Char:Character;_Char:Character;" {
                  w1562 = "iir_comb"
                  n710 = call-generic <vilib>:"NIMS_Get Row Vector_w Error - Matrix.vi"("A"=w1577) -> ("Error Enum"=w1570:T1, "Row Vector"=w1576:T2[])  [unwired: 8 in, 1 out]
                  n711 = call <vilib>:"NIMS_CH_Character RV to String.vi"("Character array"=w1576) -> ("String"=w1578:string)  [unwired: 10 in]
                  n712 = call <vilib>:"NIMS_String to Enum.vi"("Input String"=w1578, "Enum choices"=string[] ["notch", "peak"] ("Enum Options")) -> ("Error Enum"=w1569:T1, "Enum Index"=w1579:i32)  [unwired: 8 in]
                  n713 = call <vilib>:"NIMS_CH_Character 2D to U8 2D.vi"("Character 2D array"=w1582) -> ("U8 2D array"=w1581:u8[][])  [unwired: 10 in]
                  n714 = To Double Precision Float(number=w1581) -> (double precision float=w1580:dbl[][])
                  n715 = call-generic <vilib>:"NIMS_Get Scalar_w Error.vi"("A"=w1580) -> ("Error Enum"=w1571:T1, "Scalar"=w1583:dbl)  [unwired: 8 in, 1 out]
                  n716 = call <vilib>:"NIMS_CH_Character 2D to U8 2D.vi"("Character 2D array"=w1586) -> ("U8 2D array"=w1585:u8[][])  [unwired: 10 in]
                  n717 = To Double Precision Float(number=w1585) -> (double precision float=w1584:dbl[][])
                  n718 = call-generic <vilib>:"NIMS_Get Scalar_w Error.vi"("A"=w1584) -> ("Error Enum"=w1572:T1, "Scalar"=w1587:dbl)  [unwired: 8 in, 1 out]
                  n719 = call-generic <vilib>:"NIMS_Complex To Real.vi"("A"=w1590) -> ("Error Enum"=w1574:T1, "Real(A)"=w1589:dbl[][])  [unwired: 8 in, 1 out]
                  n720 = To Long Integer(number=w1589) -> (32bit integer=w1588:i32[][])
                  n721 = call-generic <vilib>:"NIMS_Get Scalar_w Error.vi"("A"=w1588) -> ("Error Enum"=w1573:T1, "Scalar"=w1591:i32)  [unwired: 8 in, 1 out]
                  n722 = call <vilib>:"NIMS_DF_iir_comb(n, bw, ab, t).vi"("type"=w1579, "ab"=w1583, "bw"=w1587, "n"=w1591) -> ("error"=w1568:i32, "b"=w1559:dbl[])  [unwired: 5 in, 1 out]
                  n723 = Build Array(w1562, w1562, w1562, w1562, w1562, w1562, "iir_comb") -> (w1565:string[])
                  n724 = Build Array(w1574, w1573, w1572, w1571, w1570, w1569, w1568) -> (w1566:i32[])
                  n725 = call <vilib>:"NIMS_Create Error From Enums.vi"("Error Code"=bool[] [FALSE, FALSE, FALSE, FALSE, FALSE, FALSE, TRUE], "error in (no error)"=w1564, "Line no"=w1567, "Error Enums"=w1566, "Function names"=w1565) -> ("error out"=w1560:errorcluster)  [unwired: 6 in]
                }
                frame "_Char:Character;;;_Char:Character;" {
                  w1595 = "iir_comb"
                  n726 = call-generic <vilib>:"NIMS_Get Row Vector_w Error - Matrix.vi"("A"=w1611) -> ("Error Enum"=w1603:T1, "Row Vector"=w1610:T2[])  [unwired: 8 in, 1 out]
                  n727 = call <vilib>:"NIMS_CH_Character RV to String.vi"("Character array"=w1610) -> ("String"=w1612:string)  [unwired: 10 in]
                  n728 = call <vilib>:"NIMS_String to Enum.vi"("Input String"=w1612, "Enum choices"=string[] ["notch", "peak"] ("Enum Options")) -> ("Error Enum"=w1602:T1, "Enum Index"=w1613:i32)  [unwired: 8 in]
                  n729 = call-generic <vilib>:"NIMS_Complex To Real.vi"("A"=w1615) -> ("Error Enum"=w1605:T1, "Real(A)"=w1614:dbl[][])  [unwired: 8 in, 1 out]
                  n730 = call-generic <vilib>:"NIMS_Get Scalar_w Error.vi"("A"=w1614) -> ("Error Enum"=w1604:T1, "Scalar"=w1616:dbl)  [unwired: 8 in, 1 out]
                  n731 = call-generic <vilib>:"NIMS_Complex To Real.vi"("A"=w1618) -> ("Error Enum"=w1607:T1, "Real(A)"=w1617:dbl[][])  [unwired: 8 in, 1 out]
                  n732 = call-generic <vilib>:"NIMS_Get Scalar_w Error.vi"("A"=w1617) -> ("Error Enum"=w1606:T1, "Scalar"=w1619:dbl)  [unwired: 8 in, 1 out]
                  n733 = call <vilib>:"NIMS_CH_Character 2D to U8 2D.vi"("Character 2D array"=w1622) -> ("U8 2D array"=w1621:u8[][])  [unwired: 10 in]
                  n734 = To Long Integer(number=w1621) -> (32bit integer=w1620:i32[][])
                  n735 = call-generic <vilib>:"NIMS_Get Scalar_w Error.vi"("A"=w1620) -> ("Error Enum"=w1608:T1, "Scalar"=w1623:i32)  [unwired: 8 in, 1 out]
                  n736 = call <vilib>:"NIMS_DF_iir_comb(n, bw, ab, t).vi"("type"=w1613, "ab"=w1616, "bw"=w1619, "n"=w1623) -> ("error"=w1601:i32, "b"=w1592:dbl[])  [unwired: 5 in, 1 out]
                  n737 = Build Array(w1595, w1595, w1595, w1595, w1595, w1595, w1595, "iir_comb") -> (w1598:string[])
                  n738 = Build Array(w1608, w1607, w1606, w1605, w1604, w1603, w1602, w1601) -> (w1599:i32[])
                  n739 = call <vilib>:"NIMS_Create Error From Enums.vi"("Error Code"=bool[] [FALSE, FALSE, FALSE, FALSE, FALSE, FALSE, FALSE, TRUE], "error in (no error)"=w1597, "Line no"=w1600, "Error Enums"=w1599, "Function names"=w1598) -> ("error out"=w1593:errorcluster)  [unwired: 6 in]
                }
                frame "_Char:Character;;_Char:Character;_Char:Character;" {
                  w1627 = "iir_comb"
                  n740 = call-generic <vilib>:"NIMS_Get Row Vector_w Error - Matrix.vi"("A"=w1642) -> ("Error Enum"=w1635:T1, "Row Vector"=w1641:T2[])  [unwired: 8 in, 1 out]
                  n741 = call <vilib>:"NIMS_CH_Character RV to String.vi"("Character array"=w1641) -> ("String"=w1643:string)  [unwired: 10 in]
                  n742 = call <vilib>:"NIMS_String to Enum.vi"("Input String"=w1643, "Enum choices"=string[] ["notch", "peak"] ("Enum Options")) -> ("Error Enum"=w1634:T1, "Enum Index"=w1644:i32)  [unwired: 8 in]
                  n743 = call <vilib>:"NIMS_CH_Character 2D to U8 2D.vi"("Character 2D array"=w1647) -> ("U8 2D array"=w1646:u8[][])  [unwired: 10 in]
                  n744 = To Double Precision Float(number=w1646) -> (double precision float=w1645:dbl[][])
                  n745 = call-generic <vilib>:"NIMS_Get Scalar_w Error.vi"("A"=w1645) -> ("Error Enum"=w1636:T1, "Scalar"=w1648:dbl)  [unwired: 8 in, 1 out]
                  n746 = call-generic <vilib>:"NIMS_Complex To Real.vi"("A"=w1650) -> ("Error Enum"=w1638:T1, "Real(A)"=w1649:dbl[][])  [unwired: 8 in, 1 out]
                  n747 = call-generic <vilib>:"NIMS_Get Scalar_w Error.vi"("A"=w1649) -> ("Error Enum"=w1637:T1, "Scalar"=w1651:dbl)  [unwired: 8 in, 1 out]
                  n748 = call <vilib>:"NIMS_CH_Character 2D to U8 2D.vi"("Character 2D array"=w1654) -> ("U8 2D array"=w1653:u8[][])  [unwired: 10 in]
                  n749 = To Long Integer(number=w1653) -> (32bit integer=w1652:i32[][])
                  n750 = call-generic <vilib>:"NIMS_Get Scalar_w Error.vi"("A"=w1652) -> ("Error Enum"=w1639:T1, "Scalar"=w1655:i32)  [unwired: 8 in, 1 out]
                  n751 = call <vilib>:"NIMS_DF_iir_comb(n, bw, ab, t).vi"("type"=w1644, "ab"=w1648, "bw"=w1651, "n"=w1655) -> ("error"=w1633:i32, "b"=w1624:dbl[])  [unwired: 5 in, 1 out]
                  n752 = Build Array(w1627, w1627, w1627, w1627, w1627, w1627, "iir_comb") -> (w1630:string[])
                  n753 = Build Array(w1639, w1638, w1637, w1636, w1635, w1634, w1633) -> (w1631:i32[])
                  n754 = call <vilib>:"NIMS_Create Error From Enums.vi"("Error Code"=bool[] [FALSE, FALSE, FALSE, FALSE, FALSE, FALSE, TRUE], "error in (no error)"=w1629, "Line no"=w1632, "Error Enums"=w1631, "Function names"=w1630) -> ("error out"=w1625:errorcluster)  [unwired: 6 in]
                }
                frame "_Char:Character;_Char:Character;;_Char:Character;" {
                  w1659 = "iir_comb"
                  n755 = call-generic <vilib>:"NIMS_Get Row Vector_w Error - Matrix.vi"("A"=w1674) -> ("Error Enum"=w1667:T1, "Row Vector"=w1673:T2[])  [unwired: 8 in, 1 out]
                  n756 = call <vilib>:"NIMS_CH_Character RV to String.vi"("Character array"=w1673) -> ("String"=w1675:string)  [unwired: 10 in]
                  n757 = call <vilib>:"NIMS_String to Enum.vi"("Input String"=w1675, "Enum choices"=string[] ["notch", "peak"] ("Enum Options")) -> ("Error Enum"=w1666:T1, "Enum Index"=w1676:i32)  [unwired: 8 in]
                  n758 = call-generic <vilib>:"NIMS_Complex To Real.vi"("A"=w1678) -> ("Error Enum"=w1669:T1, "Real(A)"=w1677:dbl[][])  [unwired: 8 in, 1 out]
                  n759 = call-generic <vilib>:"NIMS_Get Scalar_w Error.vi"("A"=w1677) -> ("Error Enum"=w1668:T1, "Scalar"=w1679:dbl)  [unwired: 8 in, 1 out]
                  n760 = call <vilib>:"NIMS_CH_Character 2D to U8 2D.vi"("Character 2D array"=w1682) -> ("U8 2D array"=w1681:u8[][])  [unwired: 10 in]
                  n761 = To Double Precision Float(number=w1681) -> (double precision float=w1680:dbl[][])
                  n762 = call-generic <vilib>:"NIMS_Get Scalar_w Error.vi"("A"=w1680) -> ("Error Enum"=w1670:T1, "Scalar"=w1683:dbl)  [unwired: 8 in, 1 out]
                  n763 = call <vilib>:"NIMS_CH_Character 2D to U8 2D.vi"("Character 2D array"=w1686) -> ("U8 2D array"=w1685:u8[][])  [unwired: 10 in]
                  n764 = To Long Integer(number=w1685) -> (32bit integer=w1684:i32[][])
                  n765 = call-generic <vilib>:"NIMS_Get Scalar_w Error.vi"("A"=w1684) -> ("Error Enum"=w1671:T1, "Scalar"=w1687:i32)  [unwired: 8 in, 1 out]
                  n766 = call <vilib>:"NIMS_DF_iir_comb(n, bw, ab, t).vi"("type"=w1676, "ab"=w1679, "bw"=w1683, "n"=w1687) -> ("error"=w1665:i32, "b"=w1656:dbl[])  [unwired: 5 in, 1 out]
                  n767 = Build Array(w1659, w1659, w1659, w1659, w1659, w1659, "iir_comb") -> (w1662:string[])
                  n768 = Build Array(w1671, w1670, w1669, w1668, w1667, w1666, w1665) -> (w1663:i32[])
                  n769 = call <vilib>:"NIMS_Create Error From Enums.vi"("Error Code"=bool[] [FALSE, FALSE, FALSE, FALSE, FALSE, FALSE, TRUE], "error in (no error)"=w1661, "Line no"=w1664, "Error Enums"=w1663, "Function names"=w1662) -> ("error out"=w1657:errorcluster)  [unwired: 6 in]
                }
                frame "_Char:Character;_Char:Character;_Char:Character;_Char:Character;" {
                  w1691 = "iir_comb"
                  n770 = call-generic <vilib>:"NIMS_Get Row Vector_w Error - Matrix.vi"("A"=w1705) -> ("Error Enum"=w1699:T1, "Row Vector"=w1704:T2[])  [unwired: 8 in, 1 out]
                  n771 = call <vilib>:"NIMS_CH_Character RV to String.vi"("Character array"=w1704) -> ("String"=w1706:string)  [unwired: 10 in]
                  n772 = call <vilib>:"NIMS_String to Enum.vi"("Input String"=w1706, "Enum choices"=string[] ["notch", "peak"] ("Enum Options")) -> ("Error Enum"=w1698:T1, "Enum Index"=w1707:i32)  [unwired: 8 in]
                  n773 = call <vilib>:"NIMS_CH_Character 2D to U8 2D.vi"("Character 2D array"=w1710) -> ("U8 2D array"=w1709:u8[][])  [unwired: 10 in]
                  n774 = To Double Precision Float(number=w1709) -> (double precision float=w1708:dbl[][])
                  n775 = call-generic <vilib>:"NIMS_Get Scalar_w Error.vi"("A"=w1708) -> ("Error Enum"=w1700:T1, "Scalar"=w1711:dbl)  [unwired: 8 in, 1 out]
                  n776 = call <vilib>:"NIMS_CH_Character 2D to U8 2D.vi"("Character 2D array"=w1714) -> ("U8 2D array"=w1713:u8[][])  [unwired: 10 in]
                  n777 = To Double Precision Float(number=w1713) -> (double precision float=w1712:dbl[][])
                  n778 = call-generic <vilib>:"NIMS_Get Scalar_w Error.vi"("A"=w1712) -> ("Error Enum"=w1701:T1, "Scalar"=w1715:dbl)  [unwired: 8 in, 1 out]
                  n779 = call <vilib>:"NIMS_CH_Character 2D to U8 2D.vi"("Character 2D array"=w1718) -> ("U8 2D array"=w1717:u8[][])  [unwired: 10 in]
                  n780 = To Long Integer(number=w1717) -> (32bit integer=w1716:i32[][])
                  n781 = call-generic <vilib>:"NIMS_Get Scalar_w Error.vi"("A"=w1716) -> ("Error Enum"=w1702:T1, "Scalar"=w1719:i32)  [unwired: 8 in, 1 out]
                  n782 = call <vilib>:"NIMS_DF_iir_comb(n, bw, ab, t).vi"("type"=w1707, "ab"=w1711, "bw"=w1715, "n"=w1719) -> ("error"=w1697:i32, "b"=w1688:dbl[])  [unwired: 5 in, 1 out]
                  n783 = Build Array(w1691, w1691, w1691, w1691, w1691, "iir_comb") -> (w1694:string[])
                  n784 = Build Array(w1702, w1701, w1700, w1699, w1698, w1697) -> (w1695:i32[])
                  n785 = call <vilib>:"NIMS_Create Error From Enums.vi"("Error Code"=bool[] [FALSE, FALSE, FALSE, FALSE, FALSE, TRUE], "error in (no error)"=w1693, "Line no"=w1696, "Error Enums"=w1695, "Function names"=w1694) -> ("error out"=w1689:errorcluster)  [unwired: 6 in]
                }
              }
              n786 = Build Array(w1431) -> (w1430:dbl[][])
              n787 = To Double Precision Complex(1:w1430) -> (0:w1429:cdb[][])
              n788 = call-generic <vilib>:"NIMS_RunTimeType_From StrictType (excl LVString).vi"("Plug-In Name"="", "Data In"=w1429) -> ("Data Out"=w1427:variant)  [unwired: 2 in]
              n789 = Build Array(w1427) -> (w1426:variant[])
            }
            frame 2 {
              n790 = Index Array(array=w1753) -> (element #1=w1749:variant, element #2=w1744:variant, element #3=w1739:variant, element #4=w1734:variant)  [unwired: 4 in]
              n791 = call <vilib>:"NIMS_RunTimeType_Get Case Value.vi"("Data In"=w1734) -> ("Case Value"=w1732:string)  [unwired: 9 in, 1 out]
              n792 = call <vilib>:"NIMS_CH_RunTimeType_To Character 2D.vi"("Variant"=w1734) -> ("data"=w1733:T2[][])  [unwired: 1 in]
              n793 = call <vilib>:"NIMS_RunTimeType_Get Case Value.vi"("Data In"=w1739) -> ("Case Value"=w1735:string)  [unwired: 9 in, 1 out]
              n794 = call <vilib>:"NIMS_CH_RunTimeType_To Character 2D.vi"("Variant"=w1739) -> ("data"=w1736:T2[][])  [unwired: 1 in]
              n795 = call-generic <vilib>:"NIMS_RunTimeType_To Numeric.vi"("DataType"=cdb[][] [], "Variant"=w1739) -> ("data"=w1737:cdb[][])  [unwired: 1 in]
              n796 = call <vilib>:"NIMS_RunTimeType_Get Case Value.vi"("Data In"=w1744) -> ("Case Value"=w1740:string)  [unwired: 9 in, 1 out]
              n797 = call <vilib>:"NIMS_CH_RunTimeType_To Character 2D.vi"("Variant"=w1744) -> ("data"=w1741:T2[][])  [unwired: 1 in]
              n798 = call-generic <vilib>:"NIMS_RunTimeType_To Numeric.vi"("DataType"=cdb[][] [], "Variant"=w1744) -> ("data"=w1742:cdb[][])  [unwired: 1 in]
              n799 = call <vilib>:"NIMS_RunTimeType_Get Case Value.vi"("Data In"=w1749) -> ("Case Value"=w1745:string)  [unwired: 9 in, 1 out]
              n800 = call <vilib>:"NIMS_CH_RunTimeType_To Character 2D.vi"("Variant"=w1749) -> ("data"=w1746:T2[][])  [unwired: 1 in]
              n801 = call-generic <vilib>:"NIMS_RunTimeType_To Numeric.vi"("DataType"=cdb[][] [], "Variant"=w1749) -> ("data"=w1747:cdb[][])  [unwired: 1 in]
              n802 = Concatenate Strings(w1745, w1740, w1735, w1732) -> (w1751:string)
              n803 = case shown="\"_Char:Character;_Char:Character;_Char:Character;_Char:Character;\"" w1751 {
                tunnel: w1750 -> [w1755 w1765 w1799 w1833 w1867 w1901 w1934 w1967 w2000]
                tunnel: [_ w1760 w1794 w1828 w1862 w1896 w1929 w1962 w1995] -> w1730
                tunnel: [_ w1759 w1793 w1827 w1861 w1895 w1928 w1961 w1994] -> w1726
                tunnel: [w1754 w1761 w1795 w1829 w1863 w1897 w1930 w1963 w1996] -> w1731
                tunnel: w1747 -> [_ w1791 w1825 w1859 w1893 _ _ _ _]
                tunnel: w1746 -> [_ _ _ _ _ w1926 w1959 w1992 w2025]
                tunnel: w1742 -> [_ w1787 w1821 _ _ w1922 w1955 _ _]
                tunnel: w1741 -> [_ _ _ w1855 w1889 _ _ w1988 w2021]
                tunnel: w1737 -> [_ w1784 _ w1851 _ w1919 _ w1984 _]
                tunnel: w1736 -> [_ _ w1818 _ w1885 _ w1952 _ w2017]
                tunnel: w1733 -> [_ w1780 w1813 w1847 w1880 w1915 w1947 w1980 w2012]
                tunnel: w1752 -> [w1758 w1768 w1802 w1836 w1870 w1904 w1937 w1970 w2003]
                frame Default {
                  n804 = call <vilib>:"Create Error.vi"("Function name"="iir_comb", "error in (no error)"=w1755, "Error Enum"=23, "Line number"=w1758) -> ("error out"=w1754:errorcluster)  [unwired: 6 in, 1 out]
                }
                frame ";;;_Char:Character;" {
                  w1763 = "iir_comb"
                  n805 = call-generic <vilib>:"NIMS_Get Row Vector_w Error - Matrix.vi"("A"=w1780) -> ("Error Enum"=w1771:T1, "Row Vector"=w1779:T2[])  [unwired: 8 in, 1 out]
                  n806 = call <vilib>:"NIMS_CH_Character RV to String.vi"("Character array"=w1779) -> ("String"=w1781:string)  [unwired: 10 in]
                  n807 = call <vilib>:"NIMS_String to Enum.vi"("Input String"=w1781, "Enum choices"=string[] ["notch", "peak"] ("Enum Options")) -> ("Error Enum"=w1770:T1, "Enum Index"=w1782:i32)  [unwired: 8 in]
                  n808 = call-generic <vilib>:"NIMS_Complex To Real.vi"("A"=w1784) -> ("Error Enum"=w1773:T1, "Real(A)"=w1783:dbl[][])  [unwired: 8 in, 1 out]
                  n809 = call-generic <vilib>:"NIMS_Get Scalar_w Error.vi"("A"=w1783) -> ("Error Enum"=w1772:T1, "Scalar"=w1785:dbl)  [unwired: 8 in, 1 out]
                  n810 = call-generic <vilib>:"NIMS_Complex To Real.vi"("A"=w1787) -> ("Error Enum"=w1775:T1, "Real(A)"=w1786:dbl[][])  [unwired: 8 in, 1 out]
                  n811 = call-generic <vilib>:"NIMS_Get Scalar_w Error.vi"("A"=w1786) -> ("Error Enum"=w1774:T1, "Scalar"=w1788:dbl)  [unwired: 8 in, 1 out]
                  n812 = call-generic <vilib>:"NIMS_Complex To Real.vi"("A"=w1791) -> ("Error Enum"=w1777:T1, "Real(A)"=w1790:dbl[][])  [unwired: 8 in, 1 out]
                  n813 = To Long Integer(number=w1790) -> (32bit integer=w1789:i32[][])
                  n814 = call-generic <vilib>:"NIMS_Get Scalar_w Error.vi"("A"=w1789) -> ("Error Enum"=w1776:T1, "Scalar"=w1792:i32)  [unwired: 8 in, 1 out]
                  n815 = call <vilib>:"NIMS_DF_iir_comb(n, bw, ab, t).vi"("type"=w1782, "ab"=w1785, "bw"=w1788, "n"=w1792) -> ("error"=w1769:i32, "a"=w1759:dbl[], "b"=w1760:dbl[])  [unwired: 5 in]
                  n816 = Build Array(w1763, w1763, w1763, w1763, w1763, w1763, w1763, w1763, "iir_comb") -> (w1766:string[])
                  n817 = Build Array(w1777, w1776, w1775, w1774, w1773, w1772, w1771, w1770, w1769) -> (w1767:i32[])
                  n818 = call <vilib>:"NIMS_Create Error From Enums.vi"("Error Code"=bool[] [FALSE, FALSE, FALSE, FALSE, FALSE, FALSE, FALSE, FALSE, TRUE], "error in (no error)"=w1765, "Line no"=w1768, "Error Enums"=w1767, "Function names"=w1766) -> ("error out"=w1761:errorcluster)  [unwired: 6 in]
                }
                frame ";;_Char:Character;_Char:Character;" {
                  w1797 = "iir_comb"
                  n819 = call-generic <vilib>:"NIMS_Get Row Vector_w Error - Matrix.vi"("A"=w1813) -> ("Error Enum"=w1805:T1, "Row Vector"=w1812:T2[])  [unwired: 8 in, 1 out]
                  n820 = call <vilib>:"NIMS_CH_Character RV to String.vi"("Character array"=w1812) -> ("String"=w1814:string)  [unwired: 10 in]
                  n821 = call <vilib>:"NIMS_String to Enum.vi"("Input String"=w1814, "Enum choices"=string[] ["notch", "peak"] ("Enum Options")) -> ("Error Enum"=w1804:T1, "Enum Index"=w1815:i32)  [unwired: 8 in]
                  n822 = call <vilib>:"NIMS_CH_Character 2D to U8 2D.vi"("Character 2D array"=w1818) -> ("U8 2D array"=w1817:u8[][])  [unwired: 10 in]
                  n823 = To Double Precision Float(number=w1817) -> (double precision float=w1816:dbl[][])
                  n824 = call-generic <vilib>:"NIMS_Get Scalar_w Error.vi"("A"=w1816) -> ("Error Enum"=w1806:T1, "Scalar"=w1819:dbl)  [unwired: 8 in, 1 out]
                  n825 = call-generic <vilib>:"NIMS_Complex To Real.vi"("A"=w1821) -> ("Error Enum"=w1808:T1, "Real(A)"=w1820:dbl[][])  [unwired: 8 in, 1 out]
                  n826 = call-generic <vilib>:"NIMS_Get Scalar_w Error.vi"("A"=w1820) -> ("Error Enum"=w1807:T1, "Scalar"=w1822:dbl)  [unwired: 8 in, 1 out]
                  n827 = call-generic <vilib>:"NIMS_Complex To Real.vi"("A"=w1825) -> ("Error Enum"=w1810:T1, "Real(A)"=w1824:dbl[][])  [unwired: 8 in, 1 out]
                  n828 = To Long Integer(number=w1824) -> (32bit integer=w1823:i32[][])
                  n829 = call-generic <vilib>:"NIMS_Get Scalar_w Error.vi"("A"=w1823) -> ("Error Enum"=w1809:T1, "Scalar"=w1826:i32)  [unwired: 8 in, 1 out]
                  n830 = call <vilib>:"NIMS_DF_iir_comb(n, bw, ab, t).vi"("type"=w1815, "ab"=w1819, "bw"=w1822, "n"=w1826) -> ("error"=w1803:i32, "a"=w1793:dbl[], "b"=w1794:dbl[])  [unwired: 5 in]
                  n831 = Build Array(w1797, w1797, w1797, w1797, w1797, w1797, w1797, "iir_comb") -> (w1800:string[])
                  n832 = Build Array(w1810, w1809, w1808, w1807, w1806, w1805, w1804, w1803) -> (w1801:i32[])
                  n833 = call <vilib>:"NIMS_Create Error From Enums.vi"("Error Code"=bool[] [FALSE, FALSE, FALSE, FALSE, FALSE, FALSE, FALSE, TRUE], "error in (no error)"=w1799, "Line no"=w1802, "Error Enums"=w1801, "Function names"=w1800) -> ("error out"=w1795:errorcluster)  [unwired: 6 in]
                }
                frame ";_Char:Character;;_Char:Character;" {
                  w1831 = "iir_comb"
                  n834 = call-generic <vilib>:"NIMS_Get Row Vector_w Error - Matrix.vi"("A"=w1847) -> ("Error Enum"=w1839:T1, "Row Vector"=w1846:T2[])  [unwired: 8 in, 1 out]
                  n835 = call <vilib>:"NIMS_CH_Character RV to String.vi"("Character array"=w1846) -> ("String"=w1848:string)  [unwired: 10 in]
                  n836 = call <vilib>:"NIMS_String to Enum.vi"("Input String"=w1848, "Enum choices"=string[] ["notch", "peak"] ("Enum Options")) -> ("Error Enum"=w1838:T1, "Enum Index"=w1849:i32)  [unwired: 8 in]
                  n837 = call-generic <vilib>:"NIMS_Complex To Real.vi"("A"=w1851) -> ("Error Enum"=w1841:T1, "Real(A)"=w1850:dbl[][])  [unwired: 8 in, 1 out]
                  n838 = call-generic <vilib>:"NIMS_Get Scalar_w Error.vi"("A"=w1850) -> ("Error Enum"=w1840:T1, "Scalar"=w1852:dbl)  [unwired: 8 in, 1 out]
                  n839 = call <vilib>:"NIMS_CH_Character 2D to U8 2D.vi"("Character 2D array"=w1855) -> ("U8 2D array"=w1854:u8[][])  [unwired: 10 in]
                  n840 = To Double Precision Float(number=w1854) -> (double precision float=w1853:dbl[][])
                  n841 = call-generic <vilib>:"NIMS_Get Scalar_w Error.vi"("A"=w1853) -> ("Error Enum"=w1842:T1, "Scalar"=w1856:dbl)  [unwired: 8 in, 1 out]
                  n842 = call-generic <vilib>:"NIMS_Complex To Real.vi"("A"=w1859) -> ("Error Enum"=w1844:T1, "Real(A)"=w1858:dbl[][])  [unwired: 8 in, 1 out]
                  n843 = To Long Integer(number=w1858) -> (32bit integer=w1857:i32[][])
                  n844 = call-generic <vilib>:"NIMS_Get Scalar_w Error.vi"("A"=w1857) -> ("Error Enum"=w1843:T1, "Scalar"=w1860:i32)  [unwired: 8 in, 1 out]
                  n845 = call <vilib>:"NIMS_DF_iir_comb(n, bw, ab, t).vi"("type"=w1849, "ab"=w1852, "bw"=w1856, "n"=w1860) -> ("error"=w1837:i32, "a"=w1827:dbl[], "b"=w1828:dbl[])  [unwired: 5 in]
                  n846 = Build Array(w1831, w1831, w1831, w1831, w1831, w1831, w1831, "iir_comb") -> (w1834:string[])
                  n847 = Build Array(w1844, w1843, w1842, w1841, w1840, w1839, w1838, w1837) -> (w1835:i32[])
                  n848 = call <vilib>:"NIMS_Create Error From Enums.vi"("Error Code"=bool[] [FALSE, FALSE, FALSE, FALSE, FALSE, FALSE, FALSE, TRUE], "error in (no error)"=w1833, "Line no"=w1836, "Error Enums"=w1835, "Function names"=w1834) -> ("error out"=w1829:errorcluster)  [unwired: 6 in]
                }
                frame ";_Char:Character;_Char:Character;_Char:Character;" {
                  w1865 = "iir_comb"
                  n849 = call-generic <vilib>:"NIMS_Get Row Vector_w Error - Matrix.vi"("A"=w1880) -> ("Error Enum"=w1873:T1, "Row Vector"=w1879:T2[])  [unwired: 8 in, 1 out]
                  n850 = call <vilib>:"NIMS_CH_Character RV to String.vi"("Character array"=w1879) -> ("String"=w1881:string)  [unwired: 10 in]
                  n851 = call <vilib>:"NIMS_String to Enum.vi"("Input String"=w1881, "Enum choices"=string[] ["notch", "peak"] ("Enum Options")) -> ("Error Enum"=w1872:T1, "Enum Index"=w1882:i32)  [unwired: 8 in]
                  n852 = call <vilib>:"NIMS_CH_Character 2D to U8 2D.vi"("Character 2D array"=w1885) -> ("U8 2D array"=w1884:u8[][])  [unwired: 10 in]
                  n853 = To Double Precision Float(number=w1884) -> (double precision float=w1883:dbl[][])
                  n854 = call-generic <vilib>:"NIMS_Get Scalar_w Error.vi"("A"=w1883) -> ("Error Enum"=w1874:T1, "Scalar"=w1886:dbl)  [unwired: 8 in, 1 out]
                  n855 = call <vilib>:"NIMS_CH_Character 2D to U8 2D.vi"("Character 2D array"=w1889) -> ("U8 2D array"=w1888:u8[][])  [unwired: 10 in]
                  n856 = To Double Precision Float(number=w1888) -> (double precision float=w1887:dbl[][])
                  n857 = call-generic <vilib>:"NIMS_Get Scalar_w Error.vi"("A"=w1887) -> ("Error Enum"=w1875:T1, "Scalar"=w1890:dbl)  [unwired: 8 in, 1 out]
                  n858 = call-generic <vilib>:"NIMS_Complex To Real.vi"("A"=w1893) -> ("Error Enum"=w1877:T1, "Real(A)"=w1892:dbl[][])  [unwired: 8 in, 1 out]
                  n859 = To Long Integer(number=w1892) -> (32bit integer=w1891:i32[][])
                  n860 = call-generic <vilib>:"NIMS_Get Scalar_w Error.vi"("A"=w1891) -> ("Error Enum"=w1876:T1, "Scalar"=w1894:i32)  [unwired: 8 in, 1 out]
                  n861 = call <vilib>:"NIMS_DF_iir_comb(n, bw, ab, t).vi"("type"=w1882, "ab"=w1886, "bw"=w1890, "n"=w1894) -> ("error"=w1871:i32, "a"=w1861:dbl[], "b"=w1862:dbl[])  [unwired: 5 in]
                  n862 = Build Array(w1865, w1865, w1865, w1865, w1865, w1865, "iir_comb") -> (w1868:string[])
                  n863 = Build Array(w1877, w1876, w1875, w1874, w1873, w1872, w1871) -> (w1869:i32[])
                  n864 = call <vilib>:"NIMS_Create Error From Enums.vi"("Error Code"=bool[] [FALSE, FALSE, FALSE, FALSE, FALSE, FALSE, TRUE], "error in (no error)"=w1867, "Line no"=w1870, "Error Enums"=w1869, "Function names"=w1868) -> ("error out"=w1863:errorcluster)  [unwired: 6 in]
                }
                frame "_Char:Character;;;_Char:Character;" {
                  w1899 = "iir_comb"
                  n865 = call-generic <vilib>:"NIMS_Get Row Vector_w Error - Matrix.vi"("A"=w1915) -> ("Error Enum"=w1907:T1, "Row Vector"=w1914:T2[])  [unwired: 8 in, 1 out]
                  n866 = call <vilib>:"NIMS_CH_Character RV to String.vi"("Character array"=w1914) -> ("String"=w1916:string)  [unwired: 10 in]
                  n867 = call <vilib>:"NIMS_String to Enum.vi"("Input String"=w1916, "Enum choices"=string[] ["notch", "peak"] ("Enum Options")) -> ("Error Enum"=w1906:T1, "Enum Index"=w1917:i32)  [unwired: 8 in]
                  n868 = call-generic <vilib>:"NIMS_Complex To Real.vi"("A"=w1919) -> ("Error Enum"=w1909:T1, "Real(A)"=w1918:dbl[][])  [unwired: 8 in, 1 out]
                  n869 = call-generic <vilib>:"NIMS_Get Scalar_w Error.vi"("A"=w1918) -> ("Error Enum"=w1908:T1, "Scalar"=w1920:dbl)  [unwired: 8 in, 1 out]
                  n870 = call-generic <vilib>:"NIMS_Complex To Real.vi"("A"=w1922) -> ("Error Enum"=w1911:T1, "Real(A)"=w1921:dbl[][])  [unwired: 8 in, 1 out]
                  n871 = call-generic <vilib>:"NIMS_Get Scalar_w Error.vi"("A"=w1921) -> ("Error Enum"=w1910:T1, "Scalar"=w1923:dbl)  [unwired: 8 in, 1 out]
                  n872 = call <vilib>:"NIMS_CH_Character 2D to U8 2D.vi"("Character 2D array"=w1926) -> ("U8 2D array"=w1925:u8[][])  [unwired: 10 in]
                  n873 = To Long Integer(number=w1925) -> (32bit integer=w1924:i32[][])
                  n874 = call-generic <vilib>:"NIMS_Get Scalar_w Error.vi"("A"=w1924) -> ("Error Enum"=w1912:T1, "Scalar"=w1927:i32)  [unwired: 8 in, 1 out]
                  n875 = call <vilib>:"NIMS_DF_iir_comb(n, bw, ab, t).vi"("type"=w1917, "ab"=w1920, "bw"=w1923, "n"=w1927) -> ("error"=w1905:i32, "a"=w1895:dbl[], "b"=w1896:dbl[])  [unwired: 5 in]
                  n876 = Build Array(w1899, w1899, w1899, w1899, w1899, w1899, w1899, "iir_comb") -> (w1902:string[])
                  n877 = Build Array(w1912, w1911, w1910, w1909, w1908, w1907, w1906, w1905) -> (w1903:i32[])
                  n878 = call <vilib>:"NIMS_Create Error From Enums.vi"("Error Code"=bool[] [FALSE, FALSE, FALSE, FALSE, FALSE, FALSE, FALSE, TRUE], "error in (no error)"=w1901, "Line no"=w1904, "Error Enums"=w1903, "Function names"=w1902) -> ("error out"=w1897:errorcluster)  [unwired: 6 in]
                }
                frame "_Char:Character;;_Char:Character;_Char:Character;" {
                  w1932 = "iir_comb"
                  n879 = call-generic <vilib>:"NIMS_Get Row Vector_w Error - Matrix.vi"("A"=w1947) -> ("Error Enum"=w1940:T1, "Row Vector"=w1946:T2[])  [unwired: 8 in, 1 out]
                  n880 = call <vilib>:"NIMS_CH_Character RV to String.vi"("Character array"=w1946) -> ("String"=w1948:string)  [unwired: 10 in]
                  n881 = call <vilib>:"NIMS_String to Enum.vi"("Input String"=w1948, "Enum choices"=string[] ["notch", "peak"] ("Enum Options")) -> ("Error Enum"=w1939:T1, "Enum Index"=w1949:i32)  [unwired: 8 in]
                  n882 = call <vilib>:"NIMS_CH_Character 2D to U8 2D.vi"("Character 2D array"=w1952) -> ("U8 2D array"=w1951:u8[][])  [unwired: 10 in]
                  n883 = To Double Precision Float(number=w1951) -> (double precision float=w1950:dbl[][])
                  n884 = call-generic <vilib>:"NIMS_Get Scalar_w Error.vi"("A"=w1950) -> ("Error Enum"=w1941:T1, "Scalar"=w1953:dbl)  [unwired: 8 in, 1 out]
                  n885 = call-generic <vilib>:"NIMS_Complex To Real.vi"("A"=w1955) -> ("Error Enum"=w1943:T1, "Real(A)"=w1954:dbl[][])  [unwired: 8 in, 1 out]
                  n886 = call-generic <vilib>:"NIMS_Get Scalar_w Error.vi"("A"=w1954) -> ("Error Enum"=w1942:T1, "Scalar"=w1956:dbl)  [unwired: 8 in, 1 out]
                  n887 = call <vilib>:"NIMS_CH_Character 2D to U8 2D.vi"("Character 2D array"=w1959) -> ("U8 2D array"=w1958:u8[][])  [unwired: 10 in]
                  n888 = To Long Integer(number=w1958) -> (32bit integer=w1957:i32[][])
                  n889 = call-generic <vilib>:"NIMS_Get Scalar_w Error.vi"("A"=w1957) -> ("Error Enum"=w1944:T1, "Scalar"=w1960:i32)  [unwired: 8 in, 1 out]
                  n890 = call <vilib>:"NIMS_DF_iir_comb(n, bw, ab, t).vi"("type"=w1949, "ab"=w1953, "bw"=w1956, "n"=w1960) -> ("error"=w1938:i32, "a"=w1928:dbl[], "b"=w1929:dbl[])  [unwired: 5 in]
                  n891 = Build Array(w1932, w1932, w1932, w1932, w1932, w1932, "iir_comb") -> (w1935:string[])
                  n892 = Build Array(w1944, w1943, w1942, w1941, w1940, w1939, w1938) -> (w1936:i32[])
                  n893 = call <vilib>:"NIMS_Create Error From Enums.vi"("Error Code"=bool[] [FALSE, FALSE, FALSE, FALSE, FALSE, FALSE, TRUE], "error in (no error)"=w1934, "Line no"=w1937, "Error Enums"=w1936, "Function names"=w1935) -> ("error out"=w1930:errorcluster)  [unwired: 6 in]
                }
                frame "_Char:Character;_Char:Character;;_Char:Character;" {
                  w1965 = "iir_comb"
                  n894 = call-generic <vilib>:"NIMS_Get Row Vector_w Error - Matrix.vi"("A"=w1980) -> ("Error Enum"=w1973:T1, "Row Vector"=w1979:T2[])  [unwired: 8 in, 1 out]
                  n895 = call <vilib>:"NIMS_CH_Character RV to String.vi"("Character array"=w1979) -> ("String"=w1981:string)  [unwired: 10 in]
                  n896 = call <vilib>:"NIMS_String to Enum.vi"("Input String"=w1981, "Enum choices"=string[] ["notch", "peak"] ("Enum Options")) -> ("Error Enum"=w1972:T1, "Enum Index"=w1982:i32)  [unwired: 8 in]
                  n897 = call-generic <vilib>:"NIMS_Complex To Real.vi"("A"=w1984) -> ("Error Enum"=w1975:T1, "Real(A)"=w1983:dbl[][])  [unwired: 8 in, 1 out]
                  n898 = call-generic <vilib>:"NIMS_Get Scalar_w Error.vi"("A"=w1983) -> ("Error Enum"=w1974:T1, "Scalar"=w1985:dbl)  [unwired: 8 in, 1 out]
                  n899 = call <vilib>:"NIMS_CH_Character 2D to U8 2D.vi"("Character 2D array"=w1988) -> ("U8 2D array"=w1987:u8[][])  [unwired: 10 in]
                  n900 = To Double Precision Float(number=w1987) -> (double precision float=w1986:dbl[][])
                  n901 = call-generic <vilib>:"NIMS_Get Scalar_w Error.vi"("A"=w1986) -> ("Error Enum"=w1976:T1, "Scalar"=w1989:dbl)  [unwired: 8 in, 1 out]
                  n902 = call <vilib>:"NIMS_CH_Character 2D to U8 2D.vi"("Character 2D array"=w1992) -> ("U8 2D array"=w1991:u8[][])  [unwired: 10 in]
                  n903 = To Long Integer(number=w1991) -> (32bit integer=w1990:i32[][])
                  n904 = call-generic <vilib>:"NIMS_Get Scalar_w Error.vi"("A"=w1990) -> ("Error Enum"=w1977:T1, "Scalar"=w1993:i32)  [unwired: 8 in, 1 out]
                  n905 = call <vilib>:"NIMS_DF_iir_comb(n, bw, ab, t).vi"("type"=w1982, "ab"=w1985, "bw"=w1989, "n"=w1993) -> ("error"=w1971:i32, "a"=w1961:dbl[], "b"=w1962:dbl[])  [unwired: 5 in]
                  n906 = Build Array(w1965, w1965, w1965, w1965, w1965, w1965, "iir_comb") -> (w1968:string[])
                  n907 = Build Array(w1977, w1976, w1975, w1974, w1973, w1972, w1971) -> (w1969:i32[])
                  n908 = call <vilib>:"NIMS_Create Error From Enums.vi"("Error Code"=bool[] [FALSE, FALSE, FALSE, FALSE, FALSE, FALSE, TRUE], "error in (no error)"=w1967, "Line no"=w1970, "Error Enums"=w1969, "Function names"=w1968) -> ("error out"=w1963:errorcluster)  [unwired: 6 in]
                }
                frame "_Char:Character;_Char:Character;_Char:Character;_Char:Character;" {
                  w1998 = "iir_comb"
                  n909 = call-generic <vilib>:"NIMS_Get Row Vector_w Error - Matrix.vi"("A"=w2012) -> ("Error Enum"=w2006:T1, "Row Vector"=w2011:T2[])  [unwired: 8 in, 1 out]
                  n910 = call <vilib>:"NIMS_CH_Character RV to String.vi"("Character array"=w2011) -> ("String"=w2013:string)  [unwired: 10 in]
                  n911 = call <vilib>:"NIMS_String to Enum.vi"("Input String"=w2013, "Enum choices"=string[] ["notch", "peak"] ("Enum Options")) -> ("Error Enum"=w2005:T1, "Enum Index"=w2014:i32)  [unwired: 8 in]
                  n912 = call <vilib>:"NIMS_CH_Character 2D to U8 2D.vi"("Character 2D array"=w2017) -> ("U8 2D array"=w2016:u8[][])  [unwired: 10 in]
                  n913 = To Double Precision Float(number=w2016) -> (double precision float=w2015:dbl[][])
                  n914 = call-generic <vilib>:"NIMS_Get Scalar_w Error.vi"("A"=w2015) -> ("Error Enum"=w2007:T1, "Scalar"=w2018:dbl)  [unwired: 8 in, 1 out]
                  n915 = call <vilib>:"NIMS_CH_Character 2D to U8 2D.vi"("Character 2D array"=w2021) -> ("U8 2D array"=w2020:u8[][])  [unwired: 10 in]
                  n916 = To Double Precision Float(number=w2020) -> (double precision float=w2019:dbl[][])
                  n917 = call-generic <vilib>:"NIMS_Get Scalar_w Error.vi"("A"=w2019) -> ("Error Enum"=w2008:T1, "Scalar"=w2022:dbl)  [unwired: 8 in, 1 out]
                  n918 = call <vilib>:"NIMS_CH_Character 2D to U8 2D.vi"("Character 2D array"=w2025) -> ("U8 2D array"=w2024:u8[][])  [unwired: 10 in]
                  n919 = To Long Integer(number=w2024) -> (32bit integer=w2023:i32[][])
                  n920 = call-generic <vilib>:"NIMS_Get Scalar_w Error.vi"("A"=w2023) -> ("Error Enum"=w2009:T1, "Scalar"=w2026:i32)  [unwired: 8 in, 1 out]
                  n921 = call <vilib>:"NIMS_DF_iir_comb(n, bw, ab, t).vi"("type"=w2014, "ab"=w2018, "bw"=w2022, "n"=w2026) -> ("error"=w2004:i32, "a"=w1994:dbl[], "b"=w1995:dbl[])  [unwired: 5 in]
                  n922 = Build Array(w1998, w1998, w1998, w1998, w1998, "iir_comb") -> (w2001:string[])
                  n923 = Build Array(w2009, w2008, w2007, w2006, w2005, w2004) -> (w2002:i32[])
                  n924 = call <vilib>:"NIMS_Create Error From Enums.vi"("Error Code"=bool[] [FALSE, FALSE, FALSE, FALSE, FALSE, TRUE], "error in (no error)"=w2000, "Line no"=w2003, "Error Enums"=w2002, "Function names"=w2001) -> ("error out"=w1996:errorcluster)  [unwired: 6 in]
                }
              }
              n925 = Build Array(w1726) -> (w1725:dbl[][])
              n926 = To Double Precision Complex(1:w1725) -> (0:w1724:cdb[][])
              n927 = call-generic <vilib>:"NIMS_RunTimeType_From StrictType (excl LVString).vi"("Plug-In Name"="", "Data In"=w1724) -> ("Data Out"=w1721:variant)  [unwired: 2 in]
              n928 = Build Array(w1730) -> (w1729:dbl[][])
              n929 = To Double Precision Complex(1:w1729) -> (0:w1728:cdb[][])
              n930 = call-generic <vilib>:"NIMS_RunTimeType_From StrictType (excl LVString).vi"("Plug-In Name"="", "Data In"=w1728) -> ("Data Out"=w1722:variant)  [unwired: 2 in]
              n931 = Build Array(w1722, w1721) -> (w1720:variant[])
            }
          }
        }
      }
    }
    frame Error {
    }
  }
  "error out" <- w3
  "[funct(A)]" <- w4
